vi "PC_JKS_v3.vi"() -> ()   [LabVIEW 2014]
panel:
  out "Strains":dbl[](array[numeric])
  out "Bosch.controller.values":dbl[](array[numeric])
  out "Mixed":dbl[](array[numeric])
  out "Override.values":dbl[](array[numeric])
  in  "Plot loop time":i64=50
  out "Comp":dbl[](array[numeric])
  out "Ramp":dbl[](array[numeric])
  out "Valves":dbl[](array[numeric])
  out "Sensors":dbl[](array[numeric])
  out "Time [s]":dbl
  out "Start.log":bool
  out "Log active 2":bool
  in  "Tab Control":T1(tab)
  in  "Stop logging":bool
  out "Numeric":i32
  out "Log active":bool
  in  "Log time (s)":dbl=20.0 caption="Time Target (s)"
  out "Elapsed Time (s)":dbl
  in  "Log frequency [ms]":u32=10
  in  "Start logging":bool
  out "Ready to save":bool
  in  "Filename":string="File"
  in  "Path":string="C:\\Dokumenter\\Dropbox\\Phd\\UiA\\Measurement\\Green_rig_data\\"
  in  "Prepare log":bool
  out "Waiting":bool
  out "U_PVG":dbl
  out "U_HAWE":dbl
  out "u_DCV":dbl=63.567989349365234
  out "P.B.HP":dbl=63.611995697021484
  out "u_Bosch":dbl
  out "FB.DCV":dbl=-1.8625760078430176
  out "P.B":dbl=70.21202850341797
  out "P.A":dbl=21.1690616607666
  out "P.return":dbl=0.036249998956918716
  out "P.pump":dbl=0.9932812452316284
  out "x.c":dbl=-0.41861194372177124
  out "P.B.LP":dbl=-0.3017437160015106
  out "P.A1":dbl=21.6378116607666
  out "Q.B":dbl=0.178985595703125
  out "FB.Bosch":dbl=0.0007812500116415322
  out "P.comp":dbl=0.15499994158744812
  out "u_DCV_comp":dbl
  out "Ramp.tr [s]":dbl
  out "Ramp.t.ramp [s]":dbl
  out "Ramp.ymax":dbl
  out "Ramp.direction":dbl
  out "Ramp.td [s]":dbl
  out "Comp.kF.gain":dbl
  out "Comp.Q.to.U.gain":dbl
  out "U_Bosch":dbl
  out "x.c.dot":dbl=63.611995697021484
  out "P.B.LP.v2":dbl=63.611995697021484
  out "Fake PB pressure":dbl
  out "Bosch Operation mode":dbl
  out "Bosch.p.term":dbl
  out "Bosch.i.term":dbl
  out "Bosch.d.term":dbl
  out "dL lowpass cutoff freq [Hz]":dbl
  out "dL HP cutoff freq [Hz]":dbl
  out "Pb highpass cutoff freq [Hz]":dbl
  out "Pb lowpass cutoff freq [Hz]":dbl
  out "Lower pressure limit [bar]":dbl
  out "Upper pressure limit [bar]":dbl
  out "Pressure (lowpass / direct (off))":dbl
  out "dpOpen (bar)":dbl
  out "Proportional.Gain":dbl
  out "Integral.Gain":dbl
  out "Derivative.Gain":dbl
  out "Bosch.ff.term":dbl
  out "Strain_unfiltered":dbl
  out "Strain_filtered":dbl
  out "plot_p_A_p_B":T2(graph)
  out "Pressure secondary circuit":T3(graph)
  out "plot_pressures":T4(graph)=[{"plot3"=[{"timer"=10600.0390625, "p_A"=21.1690616607666, "p_A1"=-0.41861194372177124}, {"timer"=10599.939453125, "p_A"=21.2081241607666, "p_A1"=-0.3771619200706482}, {"timer"=10599.859375, "p_A"=20.9737491607666, "p_A1"=-0.33571189641952515}, {"timer"=10599.7578125, "p_A"=20.7003116607666, "p_A1"=-0.25281187891960144}, {"timer"=10599.658203125, "p_A"=20.5245304107666, "p_A1"=-0.2942619025707245}, {"timer"=10599.55859375, "p_A"=20.8565616607666, "p_A1"=-0.25281187891960144}, {"timer"=10599.439453125, "p_A"=20.5049991607666, "p_A1"=-0.25281187891960144}, {"timer"=10599.337890625, "p_A"=20.0557804107666, "p_A1"=-0.2113618403673172}, {"timer"=10599.2578125, "p_A"=19.587032318115234, "p_A1"=-0.2942619025707245}, {"timer"=10599.158203125, "p_A"=19.743282318115234, "p_A1"=-0.1284618079662323}, {"timer"=10599.05859375, "p_A"=19.450313568115234, "p_A1"=-0.25281187891960144}, {"timer"=10598.958984375, "p_A"=19.333126068115234, "p_A1"=-0.2113618403673172}, {"timer"=10598.837890625, "p_A"=18.630001068115234, "p_A1"=-0.25281187891960144}, {"timer"=10598.73828125, "p_A"=18.864376068115234, "p_A1"=-0.33571189641952515}, {"timer"=10598.638671875, "p_A"=18.239376068115234, "p_A1"=-0.25281187891960144}, {"timer"=10598.55859375, "p_A"=18.141719818115234, "p_A1"=-0.25281187891960144}, {"timer"=10598.458984375, "p_A"=17.712032318115234, "p_A1"=-0.33571189641952515}, {"timer"=10598.359375, "p_A"=17.477657318115234, "p_A1"=-0.2942619025707245}, {"timer"=10598.23828125, "p_A"=17.380001068115234, "p_A1"=-0.2113618403673172}, {"timer"=10598.138671875, "p_A"=17.145626068115234, "p_A1"=-0.41861194372177124}, {"timer"=10598.05859375, "p_A"=16.891719818115234, "p_A1"=-0.33571189641952515}, {"timer"=10597.958984375, "p_A"=16.520626068115234, "p_A1"=-0.3771619200706482}, {"timer"=10597.859375, "p_A"=16.383907318115234, "p_A1"=-0.3771619200706482}, {"timer"=10597.7578125, "p_A"=15.934687614440918, "p_A1"=-0.41861194372177124}, {"timer"=10597.658203125, "p_A"=15.778437614440918, "p_A1"=-0.41861194372177124}, {"timer"=10597.55859375, "p_A"=15.524531364440918, "p_A1"=-0.2942619025707245}, {"timer"=10597.458984375, "p_A"=15.231562614440918, "p_A1"=-0.2942619025707245}, {"timer"=10597.359375, "p_A"=15.172968864440918, "p_A1"=-0.41861194372177124}, {"timer"=10597.23828125, "p_A"=14.684687614440918, "p_A1"=-0.25281187891960144}, {"timer"=10597.158203125, "p_A"=14.294062614440918, "p_A1"=-0.33571189641952515}, {"timer"=10597.05859375, "p_A"=14.294062614440918, "p_A1"=-0.2942619025707245}, {"timer"=10596.958984375, "p_A"=13.688593864440918, "p_A1"=-0.2942619025707245}, {"timer"=10596.859375, "p_A"=13.766718864440918, "p_A1"=-0.2942619025707245}, {"timer"=10596.7578125, "p_A"=13.571406364440918, "p_A1"=-0.3771619200706482}, {"timer"=10596.658203125, "p_A"=13.180781364440918, "p_A1"=-0.2942619025707245}, {"timer"=10596.55859375, "p_A"=12.809687614440918, "p_A1"=-0.2113618403673172}, {"timer"=10596.458984375, "p_A"=12.653437614440918, "p_A1"=-0.25281187891960144}, {"timer"=10596.359375, "p_A"=12.477656364440918, "p_A1"=-0.25281187891960144}, {"timer"=10596.2578125, "p_A"=12.008906364440918, "p_A1"=-0.2113618403673172}, {"timer"=10596.158203125, "p_A"=12.008906364440918, "p_A1"=-0.2942619025707245}, {"timer"=10596.05859375, "p_A"=11.364375114440918, "p_A1"=-0.25281187891960144}, {"timer"=10595.939453125, "p_A"=11.208125114440918, "p_A1"=-0.25281187891960144}, {"timer"=10595.859375, "p_A"=10.817500114440918, "p_A1"=-0.25281187891960144}, {"timer"=10595.7578125, "p_A"=10.505000114440918, "p_A1"=-0.33571189641952515}, {"timer"=10595.658203125, "p_A"=10.661250114440918, "p_A1"=-0.2942619025707245}, {"timer"=10595.5390625, "p_A"=9.919062614440918, "p_A1"=-0.33571189641952515}, {"timer"=10595.458984375, "p_A"=10.055781364440918, "p_A1"=-0.4600619673728943}, {"timer"=10595.359375, "p_A"=9.567500114440918, "p_A1"=-0.2942619025707245}, {"timer"=10595.2578125, "p_A"=9.274531364440918, "p_A1"=-0.33571189641952515}, {"timer"=10595.158203125, "p_A"=9.020625114440918, "p_A1"=-0.25281187891960144}, {"timer"=10595.0390625, "p_A"=8.981562614440918, "p_A1"=-0.33571189641952515}, {"timer"=10594.958984375, "p_A"=8.766718864440918, "p_A1"=-0.2942619025707245}, {"timer"=10594.859375, "p_A"=8.044062614440918, "p_A1"=-0.3771619200706482}, {"timer"=10594.7578125, "p_A"=7.98546838760376, "p_A1"=-0.2942619025707245}, {"timer"=10594.658203125, "p_A"=7.80968713760376, "p_A1"=-0.2942619025707245}, {"timer"=10594.55859375, "p_A"=7.39953088760376, "p_A1"=-0.41861194372177124}, {"timer"=10594.458984375, "p_A"=7.28234338760376, "p_A1"=-0.25281187891960144}, {"timer"=10594.359375, "p_A"=6.57921838760376, "p_A1"=-0.2113618403673172}, {"timer"=10594.23828125, "p_A"=6.52062463760376, "p_A1"=-0.33571189641952515}, {"timer"=10594.138671875, "p_A"=6.16906213760376, "p_A1"=-0.3771619200706482}, {"timer"=10594.05859375, "p_A"=5.99328088760376, "p_A1"=-0.33571189641952515}, {"timer"=10593.939453125, "p_A"=6.03234338760376, "p_A1"=-0.41861194372177124}, {"timer"=10593.837890625, "p_A"=5.48546838760376, "p_A1"=-0.33571189641952515}, {"timer"=10593.7578125, "p_A"=5.36828088760376, "p_A1"=-0.2942619025707245}, {"timer"=10593.658203125, "p_A"=4.938593864440918, "p_A1"=-0.3771619200706482}, {"timer"=10593.5390625, "p_A"=4.528437614440918, "p_A1"=-0.33571189641952515}, {"timer"=10593.439453125, "p_A"=4.528437614440918, "p_A1"=-0.3771619200706482}, {"timer"=10593.337890625, "p_A"=4.040156364440918, "p_A1"=-0.3771619200706482}, {"timer"=10593.2578125, "p_A"=3.883906364440918, "p_A1"=-0.33571189641952515}, {"timer"=10593.158203125, "p_A"=3.454218864440918, "p_A1"=-0.25281187891960144}, {"timer"=10593.05859375, "p_A"=2.887812614440918, "p_A1"=-0.25281187891960144}, {"timer"=10592.939453125, "p_A"=2.770625114440918, "p_A1"=-0.2942619025707245}, {"timer"=10592.859375, "p_A"=2.419062614440918, "p_A1"=-0.41861194372177124}, {"timer"=10592.7578125, "p_A"=2.106562614440918, "p_A1"=-0.3771619200706482}, {"timer"=10592.658203125, "p_A"=2.087031364440918, "p_A1"=-0.33571189641952515}, {"timer"=10592.5390625, "p_A"=1.598750114440918, "p_A1"=-0.33571189641952515}, {"timer"=10592.458984375, "p_A"=1.0714062452316284, "p_A1"=-0.2942619025707245}, {"timer"=10592.359375, "p_A"=0.8565624952316284, "p_A1"=-0.2942619025707245}, {"timer"=10592.2578125, "p_A"=0.07531249523162842, "p_A1"=-0.41861194372177124}, {"timer"=10592.158203125, "p_A"=-0.0028125010430812836, "p_A1"=-0.5015120506286621}, {"timer"=10592.05859375, "p_A"=0.6221874952316284, "p_A1"=-0.3771619200706482}, {"timer"=10591.958984375, "p_A"=12.380000114440918, "p_A1"=-0.2942619025707245}, {"timer"=10591.859375, "p_A"=45.07530975341797, "p_A1"=-0.2942619025707245}, {"timer"=10591.7578125, "p_A"=45.60265350341797, "p_A1"=-0.25281187891960144}, {"timer"=10591.638671875, "p_A"=46.20812225341797, "p_A1"=-0.41861194372177124}, {"timer"=10591.55859375, "p_A"=64.82140350341797, "p_A1"=-0.16991183161735535}, {"timer"=10591.439453125, "p_A"=96.40343475341797, "p_A1"=1.405189037322998}, {"timer"=10591.337890625, "p_A"=96.32530975341797, "p_A1"=1.6124391555786133}, {"timer"=10591.2578125, "p_A"=88.02452850341797, "p_A1"=1.6538891792297363}, {"timer"=10591.158203125, "p_A"=90.11437225341797, "p_A1"=1.6953392028808594}, {"timer"=10591.0390625, "p_A"=100.99327850341797, "p_A1"=3.8921902179718018}, {"timer"=10590.939453125, "p_A"=90.21202850341797, "p_A1"=4.4724907875061035}, {"timer"=10590.837890625, "p_A"=83.98155975341797, "p_A1"=4.969890594482422}, {"timer"=10590.7578125, "p_A"=99.46984100341797, "p_A1"=5.011341094970703}, {"timer"=10590.658203125, "p_A"=99.46984100341797, "p_A1"=5.177141189575195}, {"timer"=10590.55859375, "p_A"=99.64562225341797, "p_A1"=5.094240665435791}, {"timer"=10590.439453125, "p_A"=99.56749725341797, "p_A1"=5.218591213226318}, {"timer"=10590.359375, "p_A"=99.45030975341797, "p_A1"=5.052791118621826}, {"timer"=10590.2578125, "p_A"=99.60655975341797, "p_A1"=5.135690689086914}, {"timer"=10590.158203125, "p_A"=99.45030975341797, "p_A1"=5.094240665435791}, {"timer"=10590.0390625, "p_A"=99.62609100341797, "p_A1"=5.260040760040283}, {"timer"=10589.939453125, "p_A"=99.62609100341797, "p_A1"=5.135690689086914}, {"timer"=10589.837890625, "p_A"=99.64562225341797, "p_A1"=5.218591213226318}, {"timer"=10589.73828125, "p_A"=99.46984100341797, "p_A1"=5.177141189575195}, {"timer"=10589.658203125, "p_A"=99.60655975341797, "p_A1"=5.177141189575195}, {"timer"=10589.5390625, "p_A"=99.64562225341797, "p_A1"=5.218591213226318}, {"timer"=10589.458984375, "p_A"=99.66515350341797, "p_A1"=5.301490783691406}, {"timer"=10589.359375, "p_A"=99.50890350341797, "p_A1"=5.3429412841796875}, {"timer"=10589.23828125, "p_A"=99.50890350341797, "p_A1"=5.218591213226318}, {"timer"=10589.158203125, "p_A"=99.48937225341797, "p_A1"=5.260040760040283}, {"timer"=10589.05859375, "p_A"=99.45030975341797, "p_A1"=5.260040760040283}, {"timer"=10588.958984375, "p_A"=99.29405975341797, "p_A1"=5.301490783691406}, {"timer"=10588.859375, "p_A"=99.35265350341797, "p_A1"=5.301490783691406}, {"timer"=10588.7578125, "p_A"=99.52843475341797, "p_A1"=5.260040760040283}, {"timer"=10588.658203125, "p_A"=99.39171600341797, "p_A1"=5.3429412841796875}, {"timer"=10588.55859375, "p_A"=99.76280975341797, "p_A1"=5.3843913078308105}, {"timer"=10588.439453125, "p_A"=99.48937225341797, "p_A1"=5.3843913078308105}, {"timer"=10588.359375, "p_A"=99.50890350341797, "p_A1"=5.3429412841796875}, {"timer"=10588.2578125, "p_A"=99.50890350341797, "p_A1"=5.425840854644775}, {"timer"=10588.158203125, "p_A"=99.39171600341797, "p_A1"=5.3843913078308105}, {"timer"=10588.0390625, "p_A"=99.41124725341797, "p_A1"=5.3429412841796875}, {"timer"=10587.939453125, "p_A"=99.48937225341797, "p_A1"=5.467290878295898}, {"timer"=10587.859375, "p_A"=99.46984100341797, "p_A1"=5.425840854644775}, {"timer"=10587.7578125, "p_A"=99.43077850341797, "p_A1"=5.50874137878418}, {"timer"=10587.638671875, "p_A"=99.60655975341797, "p_A1"=5.467290878295898}, {"timer"=10587.55859375, "p_A"=99.41124725341797, "p_A1"=5.425840854644775}, {"timer"=10587.458984375, "p_A"=99.56749725341797, "p_A1"=5.3843913078308105}, {"timer"=10587.337890625, "p_A"=99.17687225341797, "p_A1"=5.50874137878418}, {"timer"=10587.23828125, "p_A"=99.56749725341797, "p_A1"=5.50874137878418}, {"timer"=10587.158203125, "p_A"=99.54796600341797, "p_A1"=5.50874137878418}, {"timer"=10587.05859375, "p_A"=99.45030975341797, "p_A1"=5.467290878295898}, {"timer"=10586.958984375, "p_A"=99.50890350341797, "p_A1"=5.467290878295898}, {"timer"=10586.859375, "p_A"=99.54796600341797, "p_A1"=5.467290878295898}, {"timer"=10586.7578125, "p_A"=99.45030975341797, "p_A1"=5.50874137878418}, {"timer"=10586.658203125, "p_A"=99.46984100341797, "p_A1"=5.50874137878418}, {"timer"=10586.55859375, "p_A"=99.54796600341797, "p_A1"=5.591640949249268}, {"timer"=10586.458984375, "p_A"=99.45030975341797, "p_A1"=5.715991497039795}, {"timer"=10586.359375, "p_A"=99.48937225341797, "p_A1"=5.715991497039795}, {"timer"=10586.2578125, "p_A"=99.25499725341797, "p_A1"=5.591640949249268}, {"timer"=10586.158203125, "p_A"=99.86046600341797, "p_A1"=5.550191402435303}, {"timer"=10586.05859375, "p_A"=99.35265350341797, "p_A1"=5.633090972900391}, {"timer"=10585.958984375, "p_A"=99.54796600341797, "p_A1"=5.591640949249268}, {"timer"=10585.859375, "p_A"=99.31359100341797, "p_A1"=5.550191402435303}, {"timer"=10585.7578125, "p_A"=99.39171600341797, "p_A1"=5.715991497039795}, {"timer"=10585.658203125, "p_A"=99.37218475341797, "p_A1"=5.75744104385376}, {"timer"=10585.55859375, "p_A"=99.37218475341797, "p_A1"=5.633090972900391}, {"timer"=10585.458984375, "p_A"=99.21593475341797, "p_A1"=5.674541473388672}, {"timer"=10585.359375, "p_A"=99.23546600341797, "p_A1"=5.674541473388672}, {"timer"=10585.2578125, "p_A"=99.43077850341797, "p_A1"=5.715991497039795}, {"timer"=10585.158203125, "p_A"=99.37218475341797, "p_A1"=5.75744104385376}, {"timer"=10585.05859375, "p_A"=99.54796600341797, "p_A1"=5.75744104385376}, {"timer"=10584.958984375, "p_A"=99.45030975341797, "p_A1"=5.798891067504883}, {"timer"=10584.837890625, "p_A"=99.39171600341797, "p_A1"=5.715991497039795}, {"timer"=10584.7578125, "p_A"=99.60655975341797, "p_A1"=5.75744104385376}, {"timer"=10584.658203125, "p_A"=99.48937225341797, "p_A1"=5.798891067504883}, {"timer"=10584.55859375, "p_A"=99.39171600341797, "p_A1"=5.715991497039795}, {"timer"=10584.458984375, "p_A"=99.35265350341797, "p_A1"=5.674541473388672}, {"timer"=10584.359375, "p_A"=99.21593475341797, "p_A1"=5.715991497039795}, {"timer"=10584.2578125, "p_A"=99.50890350341797, "p_A1"=5.798891067504883}, {"timer"=10584.158203125, "p_A"=99.58702850341797, "p_A1"=5.840341567993164}, {"timer"=10584.05859375, "p_A"=99.39171600341797, "p_A1"=5.881791591644287}, {"timer"=10583.958984375, "p_A"=99.50890350341797, "p_A1"=5.881791591644287}, {"timer"=10583.859375, "p_A"=99.41124725341797, "p_A1"=5.92324161529541}, {"timer"=10583.7578125, "p_A"=99.33312225341797, "p_A1"=5.840341567993164}, {"timer"=10583.658203125, "p_A"=99.33312225341797, "p_A1"=5.840341567993164}, {"timer"=10583.55859375, "p_A"=99.52843475341797, "p_A1"=5.92324161529541}, {"timer"=10583.458984375, "p_A"=99.33312225341797, "p_A1"=5.840341567993164}, {"timer"=10583.359375, "p_A"=99.52843475341797, "p_A1"=6.006141662597656}, {"timer"=10583.2578125, "p_A"=99.72374725341797, "p_A1"=5.964691162109375}, {"timer"=10583.158203125, "p_A"=99.48937225341797, "p_A1"=6.006141662597656}, {"timer"=10583.05859375, "p_A"=99.41124725341797, "p_A1"=6.006141662597656}, {"timer"=10582.958984375, "p_A"=99.45030975341797, "p_A1"=6.006141662597656}, {"timer"=10582.859375, "p_A"=99.43077850341797, "p_A1"=5.964691162109375}, {"timer"=10582.7578125, "p_A"=99.41124725341797, "p_A1"=6.006141662597656}, {"timer"=10582.658203125, "p_A"=99.37218475341797, "p_A1"=6.006141662597656}, {"timer"=10582.55859375, "p_A"=99.41124725341797, "p_A1"=5.964691162109375}, {"timer"=10582.458984375, "p_A"=99.58702850341797, "p_A1"=6.006141662597656}, {"timer"=10582.359375, "p_A"=99.37218475341797, "p_A1"=6.047591686248779}, {"timer"=10582.2578125, "p_A"=99.50890350341797, "p_A1"=6.089041709899902}, {"timer"=10582.158203125, "p_A"=99.35265350341797, "p_A1"=6.089041709899902}, {"timer"=10582.0390625, "p_A"=99.60655975341797, "p_A1"=6.047591686248779}, {"timer"=10581.958984375, "p_A"=99.76280975341797, "p_A1"=6.089041709899902}, {"timer"=10581.837890625, "p_A"=99.43077850341797, "p_A1"=6.006141662597656}, {"timer"=10581.73828125, "p_A"=99.37218475341797, "p_A1"=6.130491256713867}, {"timer"=10581.658203125, "p_A"=99.27452850341797, "p_A1"=6.089041709899902}, {"timer"=10581.55859375, "p_A"=99.48937225341797, "p_A1"=6.2548418045043945}, {"timer"=10581.458984375, "p_A"=99.46984100341797, "p_A1"=6.171941757202148}, {"timer"=10581.359375, "p_A"=99.33312225341797, "p_A1"=6.2133917808532715}, {"timer"=10581.23828125, "p_A"=99.25499725341797, "p_A1"=6.2133917808532715}, {"timer"=10581.158203125, "p_A"=99.58702850341797, "p_A1"=6.296291351318359}, {"timer"=10581.05859375, "p_A"=99.31359100341797, "p_A1"=6.296291351318359}, {"timer"=10580.958984375, "p_A"=99.37218475341797, "p_A1"=6.2133917808532715}, {"timer"=10580.859375, "p_A"=99.25499725341797, "p_A1"=6.379191875457764}, {"timer"=10580.7578125, "p_A"=99.27452850341797, "p_A1"=6.379191875457764}, {"timer"=10580.658203125, "p_A"=99.41124725341797, "p_A1"=6.379191875457764}, {"timer"=10580.55859375, "p_A"=99.62609100341797, "p_A1"=6.462091445922852}, {"timer"=10580.458984375, "p_A"=99.35265350341797, "p_A1"=6.337741851806641}, {"timer"=10580.359375, "p_A"=99.29405975341797, "p_A1"=6.462091445922852}, {"timer"=10580.2578125, "p_A"=99.09874725341797, "p_A1"=6.420641899108887}, {"timer"=10580.158203125, "p_A"=99.39171600341797, "p_A1"=6.379191875457764}, {"timer"=10580.05859375, "p_A"=99.33312225341797, "p_A1"=6.420641899108887}, {"timer"=10579.939453125, "p_A"=99.39171600341797, "p_A1"=6.544991970062256}, {"timer"=10579.837890625, "p_A"=99.29405975341797, "p_A1"=6.586441993713379}, {"timer"=10579.7578125, "p_A"=99.17687225341797, "p_A1"=6.544991970062256}, {"timer"=10579.658203125, "p_A"=99.48937225341797, "p_A1"=6.586441993713379}, {"timer"=10579.55859375, "p_A"=99.23546600341797, "p_A1"=6.503541946411133}, {"timer"=10579.439453125, "p_A"=99.33312225341797, "p_A1"=6.462091445922852}, {"timer"=10579.337890625, "p_A"=99.21593475341797, "p_A1"=6.586441993713379}, {"timer"=10579.23828125, "p_A"=99.60655975341797, "p_A1"=6.544991970062256}, {"timer"=10579.138671875, "p_A"=99.39171600341797, "p_A1"=6.544991970062256}, {"timer"=10579.0390625, "p_A"=99.46984100341797, "p_A1"=6.462091445922852}, {"timer"=10578.939453125, "p_A"=99.33312225341797, "p_A1"=6.503541946411133}, {"timer"=10578.837890625, "p_A"=99.21593475341797, "p_A1"=6.544991970062256}, {"timer"=10578.73828125, "p_A"=99.35265350341797, "p_A1"=6.586441993713379}, {"timer"=10578.638671875, "p_A"=99.31359100341797, "p_A1"=6.503541946411133}, {"timer"=10578.5390625, "p_A"=99.19640350341797, "p_A1"=6.544991970062256}, {"timer"=10578.439453125, "p_A"=99.68468475341797, "p_A1"=6.627891540527344}, {"timer"=10578.337890625, "p_A"=99.07921600341797, "p_A1"=6.503541946411133}, {"timer"=10578.23828125, "p_A"=99.29405975341797, "p_A1"=6.627891540527344}, {"timer"=10578.138671875, "p_A"=99.41124725341797, "p_A1"=6.669342041015625}, {"timer"=10578.0390625, "p_A"=99.54796600341797, "p_A1"=6.669342041015625}, {"timer"=10577.939453125, "p_A"=99.15734100341797, "p_A1"=6.627891540527344}, {"timer"=10577.837890625, "p_A"=99.33312225341797, "p_A1"=6.627891540527344}, {"timer"=10577.73828125, "p_A"=99.45030975341797, "p_A1"=6.586441993713379}, {"timer"=10577.638671875, "p_A"=99.19640350341797, "p_A1"=6.669342041015625}, {"timer"=10577.5390625, "p_A"=99.17687225341797, "p_A1"=6.627891540527344}, {"timer"=10577.439453125, "p_A"=99.29405975341797, "p_A1"=6.669342041015625}, {"timer"=10577.337890625, "p_A"=99.37218475341797, "p_A1"=6.669342041015625}, {"timer"=10577.23828125, "p_A"=99.45030975341797, "p_A1"=6.669342041015625}, {"timer"=10577.138671875, "p_A"=99.37218475341797, "p_A1"=6.752242088317871}, {"timer"=10577.0390625, "p_A"=99.46984100341797, "p_A1"=6.752242088317871}, {"timer"=10576.939453125, "p_A"=99.27452850341797, "p_A1"=6.835142135620117}, {"timer"=10576.837890625, "p_A"=99.19640350341797, "p_A1"=6.793691635131836}, {"timer"=10576.73828125, "p_A"=99.29405975341797, "p_A1"=6.752242088317871}, {"timer"=10576.638671875, "p_A"=99.29405975341797, "p_A1"=6.793691635131836}, {"timer"=10576.5390625, "p_A"=99.09874725341797, "p_A1"=6.793691635131836}, {"timer"=10576.439453125, "p_A"=99.21593475341797, "p_A1"=6.918042182922363}, {"timer"=10576.337890625, "p_A"=99.25499725341797, "p_A1"=6.835142135620117}, {"timer"=10576.23828125, "p_A"=99.25499725341797, "p_A1"=6.752242088317871}, {"timer"=10576.138671875, "p_A"=99.23546600341797, "p_A1"=6.835142135620117}, {"timer"=10576.0390625, "p_A"=99.09874725341797, "p_A1"=6.87659215927124}, {"timer"=10575.939453125, "p_A"=99.35265350341797, "p_A1"=6.918042182922363}, {"timer"=10575.837890625, "p_A"=99.29405975341797, "p_A1"=6.793691635131836}, {"timer"=10575.73828125, "p_A"=99.33312225341797, "p_A1"=6.87659215927124}, {"timer"=10575.638671875, "p_A"=99.45030975341797, "p_A1"=6.835142135620117}, {"timer"=10575.5390625, "p_A"=99.29405975341797, "p_A1"=6.87659215927124}, {"timer"=10575.439453125, "p_A"=99.17687225341797, "p_A1"=6.918042182922363}, {"timer"=10575.337890625, "p_A"=99.11827850341797, "p_A1"=6.959491729736328}, {"timer"=10575.23828125, "p_A"=99.13780975341797, "p_A1"=6.87659215927124}, {"timer"=10575.138671875, "p_A"=99.09874725341797, "p_A1"=6.918042182922363}, {"timer"=10575.0390625, "p_A"=99.39171600341797, "p_A1"=6.918042182922363}, {"timer"=10574.939453125, "p_A"=99.48937225341797, "p_A1"=7.042392253875732}, {"timer"=10574.837890625, "p_A"=99.41124725341797, "p_A1"=6.918042182922363}, {"timer"=10574.73828125, "p_A"=99.45030975341797, "p_A1"=6.918042182922363}, {"timer"=10574.638671875, "p_A"=99.23546600341797, "p_A1"=7.000941753387451}, {"timer"=10574.5390625, "p_A"=99.29405975341797, "p_A1"=6.87659215927124}, {"timer"=10574.439453125, "p_A"=99.35265350341797, "p_A1"=6.87659215927124}, {"timer"=10574.337890625, "p_A"=99.29405975341797, "p_A1"=6.959491729736328}, {"timer"=10574.23828125, "p_A"=99.37218475341797, "p_A1"=7.042392253875732}, {"timer"=10574.138671875, "p_A"=99.25499725341797, "p_A1"=7.000941753387451}, {"timer"=10574.0390625, "p_A"=99.25499725341797, "p_A1"=7.000941753387451}, {"timer"=10573.939453125, "p_A"=99.25499725341797, "p_A1"=6.959491729736328}, {"timer"=10573.837890625, "p_A"=99.37218475341797, "p_A1"=7.0838422775268555}, {"timer"=10573.73828125, "p_A"=99.23546600341797, "p_A1"=7.000941753387451}, {"timer"=10573.638671875, "p_A"=99.17687225341797, "p_A1"=7.042392253875732}, {"timer"=10573.5390625, "p_A"=99.33312225341797, "p_A1"=7.000941753387451}, {"timer"=10573.439453125, "p_A"=99.19640350341797, "p_A1"=7.042392253875732}, {"timer"=10573.337890625, "p_A"=99.33312225341797, "p_A1"=7.12529182434082}, {"timer"=10573.23828125, "p_A"=99.31359100341797, "p_A1"=6.959491729736328}, {"timer"=10573.138671875, "p_A"=99.15734100341797, "p_A1"=7.000941753387451}, {"timer"=10573.0390625, "p_A"=99.27452850341797, "p_A1"=7.000941753387451}, {"timer"=10572.939453125, "p_A"=98.96202850341797, "p_A1"=6.959491729736328}, {"timer"=10572.837890625, "p_A"=99.33312225341797, "p_A1"=7.0838422775268555}, {"timer"=10572.73828125, "p_A"=99.31359100341797, "p_A1"=7.12529182434082}, {"timer"=10572.638671875, "p_A"=99.27452850341797, "p_A1"=7.042392253875732}, {"timer"=10572.5390625, "p_A"=99.15734100341797, "p_A1"=7.0838422775268555}, {"timer"=10572.439453125, "p_A"=99.33312225341797, "p_A1"=7.0838422775268555}, {"timer"=10572.337890625, "p_A"=99.31359100341797, "p_A1"=7.042392253875732}, {"timer"=10572.23828125, "p_A"=99.25499725341797, "p_A1"=7.0838422775268555}, {"timer"=10572.138671875, "p_A"=99.48937225341797, "p_A1"=7.0838422775268555}, {"timer"=10572.0390625, "p_A"=99.21593475341797, "p_A1"=7.0838422775268555}, {"timer"=10571.939453125, "p_A"=98.96202850341797, "p_A1"=7.0838422775268555}, {"timer"=10571.837890625, "p_A"=99.25499725341797, "p_A1"=7.042392253875732}, {"timer"=10571.73828125, "p_A"=99.17687225341797, "p_A1"=7.12529182434082}, {"timer"=10571.638671875, "p_A"=99.31359100341797, "p_A1"=7.12529182434082}, {"timer"=10571.5390625, "p_A"=99.13780975341797, "p_A1"=7.166741847991943}, {"timer"=10571.439453125, "p_A"=99.41124725341797, "p_A1"=7.0838422775268555}, {"timer"=10571.337890625, "p_A"=99.39171600341797, "p_A1"=7.166741847991943}, {"timer"=10571.23828125, "p_A"=99.09874725341797, "p_A1"=7.12529182434082}, {"timer"=10571.138671875, "p_A"=99.31359100341797, "p_A1"=7.12529182434082}, {"timer"=10571.0390625, "p_A"=99.09874725341797, "p_A1"=7.000941753387451}, {"timer"=10570.939453125, "p_A"=99.25499725341797, "p_A1"=7.166741847991943}, {"timer"=10570.837890625, "p_A"=99.19640350341797, "p_A1"=7.042392253875732}, {"timer"=10570.73828125, "p_A"=99.25499725341797, "p_A1"=7.0838422775268555}, {"timer"=10570.638671875, "p_A"=99.19640350341797, "p_A1"=7.166741847991943}, {"timer"=10570.5390625, "p_A"=99.25499725341797, "p_A1"=7.12529182434082}, {"timer"=10570.439453125, "p_A"=99.21593475341797, "p_A1"=7.166741847991943}, {"timer"=10570.337890625, "p_A"=99.31359100341797, "p_A1"=7.12529182434082}, {"timer"=10570.23828125, "p_A"=99.11827850341797, "p_A1"=7.0838422775268555}, {"timer"=10570.138671875, "p_A"=99.35265350341797, "p_A1"=7.0838422775268555}, {"timer"=10570.0390625, "p_A"=99.35265350341797, "p_A1"=7.12529182434082}, {"timer"=10569.939453125, "p_A"=99.39171600341797, "p_A1"=7.12529182434082}, {"timer"=10569.837890625, "p_A"=98.92296600341797, "p_A1"=7.208192348480225}, {"timer"=10569.73828125, "p_A"=99.00109100341797, "p_A1"=7.166741847991943}, {"timer"=10569.638671875, "p_A"=98.96202850341797, "p_A1"=7.12529182434082}, {"timer"=10569.5390625, "p_A"=99.04015350341797, "p_A1"=7.12529182434082}, {"timer"=10569.439453125, "p_A"=99.07921600341797, "p_A1"=7.166741847991943}, {"timer"=10569.337890625, "p_A"=99.17687225341797, "p_A1"=7.12529182434082}, {"timer"=10569.23828125, "p_A"=99.17687225341797, "p_A1"=7.12529182434082}, {"timer"=10569.138671875, "p_A"=99.11827850341797, "p_A1"=7.166741847991943}, {"timer"=10569.0390625, "p_A"=99.13780975341797, "p_A1"=7.0838422775268555}, {"timer"=10568.939453125, "p_A"=99.02062225341797, "p_A1"=7.166741847991943}, {"timer"=10568.837890625, "p_A"=99.13780975341797, "p_A1"=7.166741847991943}, {"timer"=10568.73828125, "p_A"=99.05968475341797, "p_A1"=7.166741847991943}, {"timer"=10568.638671875, "p_A"=99.21593475341797, "p_A1"=7.12529182434082}, {"timer"=10568.5390625, "p_A"=99.21593475341797, "p_A1"=7.166741847991943}, {"timer"=10568.439453125, "p_A"=99.04015350341797, "p_A1"=7.208192348480225}, {"timer"=10568.337890625, "p_A"=99.09874725341797, "p_A1"=7.12529182434082}, {"timer"=10568.23828125, "p_A"=99.21593475341797, "p_A1"=7.12529182434082}, {"timer"=10568.138671875, "p_A"=99.05968475341797, "p_A1"=7.208192348480225}, {"timer"=10568.0390625, "p_A"=99.37218475341797, "p_A1"=7.208192348480225}, {"timer"=10567.939453125, "p_A"=99.31359100341797, "p_A1"=7.208192348480225}, {"timer"=10567.837890625, "p_A"=99.07921600341797, "p_A1"=7.208192348480225}, {"timer"=10567.73828125, "p_A"=99.05968475341797, "p_A1"=7.208192348480225}, {"timer"=10567.638671875, "p_A"=99.23546600341797, "p_A1"=7.249642372131348}, {"timer"=10567.5390625, "p_A"=99.17687225341797, "p_A1"=7.249642372131348}, {"timer"=10567.439453125, "p_A"=99.07921600341797, "p_A1"=7.208192348480225}, {"timer"=10567.337890625, "p_A"=99.19640350341797, "p_A1"=7.208192348480225}, {"timer"=10567.23828125, "p_A"=99.00109100341797, "p_A1"=7.208192348480225}, {"timer"=10567.138671875, "p_A"=99.02062225341797, "p_A1"=7.208192348480225}, {"timer"=10567.0390625, "p_A"=99.19640350341797, "p_A1"=7.208192348480225}, {"timer"=10566.939453125, "p_A"=99.35265350341797, "p_A1"=7.208192348480225}, {"timer"=10566.837890625, "p_A"=98.94249725341797, "p_A1"=7.208192348480225}, {"timer"=10566.73828125, "p_A"=99.27452850341797, "p_A1"=7.249642372131348}, {"timer"=10566.638671875, "p_A"=98.86437225341797, "p_A1"=7.166741847991943}, {"timer"=10566.5390625, "p_A"=99.00109100341797, "p_A1"=7.249642372131348}, {"timer"=10566.439453125, "p_A"=98.92296600341797, "p_A1"=7.166741847991943}, {"timer"=10566.337890625, "p_A"=99.15734100341797, "p_A1"=7.166741847991943}, {"timer"=10566.23828125, "p_A"=99.04015350341797, "p_A1"=7.166741847991943}, {"timer"=10566.138671875, "p_A"=99.35265350341797, "p_A1"=7.208192348480225}, {"timer"=10566.0390625, "p_A"=99.09874725341797, "p_A1"=7.208192348480225}, {"timer"=10565.939453125, "p_A"=99.13780975341797, "p_A1"=7.249642372131348}, {"timer"=10565.837890625, "p_A"=99.17687225341797, "p_A1"=7.208192348480225}, {"timer"=10565.73828125, "p_A"=99.35265350341797, "p_A1"=7.208192348480225}, {"timer"=10565.638671875, "p_A"=99.15734100341797, "p_A1"=7.249642372131348}, {"timer"=10565.5390625, "p_A"=99.27452850341797, "p_A1"=7.208192348480225}, {"timer"=10565.439453125, "p_A"=98.94249725341797, "p_A1"=7.249642372131348}, {"timer"=10565.337890625, "p_A"=99.04015350341797, "p_A1"=7.208192348480225}, {"timer"=10565.23828125, "p_A"=99.11827850341797, "p_A1"=7.249642372131348}, {"timer"=10565.138671875, "p_A"=98.98155975341797, "p_A1"=7.208192348480225}, {"timer"=10565.0390625, "p_A"=99.02062225341797, "p_A1"=7.249642372131348}, {"timer"=10564.939453125, "p_A"=99.31359100341797, "p_A1"=7.249642372131348}, {"timer"=10564.837890625, "p_A"=99.07921600341797, "p_A1"=7.249642372131348}, {"timer"=10564.73828125, "p_A"=99.21593475341797, "p_A1"=7.208192348480225}, {"timer"=10564.638671875, "p_A"=99.27452850341797, "p_A1"=7.2910919189453125}, {"timer"=10564.5390625, "p_A"=99.27452850341797, "p_A1"=7.249642372131348}, {"timer"=10564.439453125, "p_A"=99.02062225341797, "p_A1"=7.249642372131348}, {"timer"=10564.337890625, "p_A"=99.23546600341797, "p_A1"=7.249642372131348}, {"timer"=10564.23828125, "p_A"=99.00109100341797, "p_A1"=7.249642372131348}, {"timer"=10564.138671875, "p_A"=99.23546600341797, "p_A1"=7.249642372131348}, {"timer"=10564.0390625, "p_A"=99.02062225341797, "p_A1"=7.249642372131348}, {"timer"=10563.939453125, "p_A"=99.19640350341797, "p_A1"=7.249642372131348}, {"timer"=10563.837890625, "p_A"=98.88390350341797, "p_A1"=7.249642372131348}, {"timer"=10563.73828125, "p_A"=99.11827850341797, "p_A1"=7.208192348480225}, {"timer"=10563.638671875, "p_A"=99.23546600341797, "p_A1"=7.249642372131348}, {"timer"=10563.5390625, "p_A"=99.21593475341797, "p_A1"=7.249642372131348}, {"timer"=10563.439453125, "p_A"=99.02062225341797, "p_A1"=7.249642372131348}, {"timer"=10563.337890625, "p_A"=99.11827850341797, "p_A1"=7.2910919189453125}, {"timer"=10563.23828125, "p_A"=99.02062225341797, "p_A1"=7.249642372131348}, {"timer"=10563.138671875, "p_A"=98.88390350341797, "p_A1"=7.249642372131348}, {"timer"=10563.0390625, "p_A"=99.13780975341797, "p_A1"=7.2910919189453125}, {"timer"=10562.939453125, "p_A"=98.68859100341797, "p_A1"=7.249642372131348}, {"timer"=10562.837890625, "p_A"=98.86437225341797, "p_A1"=7.249642372131348}, {"timer"=10562.73828125, "p_A"=98.94249725341797, "p_A1"=7.2910919189453125}, {"timer"=10562.638671875, "p_A"=99.04015350341797, "p_A1"=7.249642372131348}, {"timer"=10562.5390625, "p_A"=99.00109100341797, "p_A1"=7.249642372131348}, {"timer"=10562.439453125, "p_A"=98.84484100341797, "p_A1"=7.249642372131348}, {"timer"=10562.337890625, "p_A"=99.07921600341797, "p_A1"=7.249642372131348}, {"timer"=10562.23828125, "p_A"=99.02062225341797, "p_A1"=7.2910919189453125}, {"timer"=10562.138671875, "p_A"=99.15734100341797, "p_A1"=7.249642372131348}, {"timer"=10562.0390625, "p_A"=99.04015350341797, "p_A1"=7.249642372131348}, {"timer"=10561.939453125, "p_A"=99.13780975341797, "p_A1"=7.249642372131348}, {"timer"=10561.837890625, "p_A"=99.13780975341797, "p_A1"=7.2910919189453125}, {"timer"=10561.73828125, "p_A"=99.21593475341797, "p_A1"=7.2910919189453125}, {"timer"=10561.638671875, "p_A"=98.98155975341797, "p_A1"=7.249642372131348}, {"timer"=10561.5390625, "p_A"=99.04015350341797, "p_A1"=7.249642372131348}, {"timer"=10561.439453125, "p_A"=99.23546600341797, "p_A1"=7.2910919189453125}, {"timer"=10561.337890625, "p_A"=98.88390350341797, "p_A1"=7.249642372131348}, {"timer"=10561.23828125, "p_A"=99.17687225341797, "p_A1"=7.2910919189453125}, {"timer"=10561.138671875, "p_A"=99.27452850341797, "p_A1"=7.2910919189453125}, {"timer"=10561.0390625, "p_A"=99.11827850341797, "p_A1"=7.249642372131348}, {"timer"=10560.939453125, "p_A"=98.80577850341797, "p_A1"=7.249642372131348}, {"timer"=10560.837890625, "p_A"=99.17687225341797, "p_A1"=7.249642372131348}, {"timer"=10560.73828125, "p_A"=99.17687225341797, "p_A1"=7.2910919189453125}, {"timer"=10560.638671875, "p_A"=99.05968475341797, "p_A1"=7.249642372131348}, {"timer"=10560.5390625, "p_A"=99.04015350341797, "p_A1"=7.249642372131348}, {"timer"=10560.439453125, "p_A"=99.04015350341797, "p_A1"=7.249642372131348}, {"timer"=10560.337890625, "p_A"=99.13780975341797, "p_A1"=7.2910919189453125}, {"timer"=10560.23828125, "p_A"=98.94249725341797, "p_A1"=7.249642372131348}, {"timer"=10560.138671875, "p_A"=99.02062225341797, "p_A1"=7.2910919189453125}, {"timer"=10560.0390625, "p_A"=99.04015350341797, "p_A1"=7.249642372131348}, {"timer"=10559.939453125, "p_A"=99.09874725341797, "p_A1"=7.249642372131348}, {"timer"=10559.837890625, "p_A"=98.82530975341797, "p_A1"=7.2910919189453125}, {"timer"=10559.73828125, "p_A"=98.92296600341797, "p_A1"=7.2910919189453125}, {"timer"=10559.638671875, "p_A"=98.98155975341797, "p_A1"=7.249642372131348}, {"timer"=10559.5390625, "p_A"=98.76671600341797, "p_A1"=7.249642372131348}, {"timer"=10559.439453125, "p_A"=99.07921600341797, "p_A1"=7.2910919189453125}, {"timer"=10559.337890625, "p_A"=98.98155975341797, "p_A1"=7.2910919189453125}, {"timer"=10559.23828125, "p_A"=99.04015350341797, "p_A1"=7.2910919189453125}, {"timer"=10559.138671875, "p_A"=99.00109100341797, "p_A1"=7.249642372131348}, {"timer"=10559.0390625, "p_A"=98.96202850341797, "p_A1"=7.2910919189453125}, {"timer"=10558.939453125, "p_A"=99.13780975341797, "p_A1"=7.2910919189453125}, {"timer"=10558.837890625, "p_A"=98.92296600341797, "p_A1"=7.2910919189453125}, {"timer"=10558.73828125, "p_A"=98.82530975341797, "p_A1"=7.2910919189453125}, {"timer"=10558.619140625, "p_A"=99.05968475341797, "p_A1"=7.2910919189453125}, {"timer"=10558.5390625, "p_A"=98.88390350341797, "p_A1"=7.2910919189453125}, {"timer"=10558.439453125, "p_A"=98.92296600341797, "p_A1"=7.2910919189453125}, {"timer"=10558.337890625, "p_A"=98.96202850341797, "p_A1"=7.2910919189453125}, {"timer"=10558.21875, "p_A"=98.68859100341797, "p_A1"=7.2910919189453125}, {"timer"=10558.138671875, "p_A"=98.92296600341797, "p_A1"=7.2910919189453125}, {"timer"=10558.0390625, "p_A"=98.96202850341797, "p_A1"=7.2910919189453125}, {"timer"=10557.939453125, "p_A"=98.88390350341797, "p_A1"=7.249642372131348}, {"timer"=10557.837890625, "p_A"=98.94249725341797, "p_A1"=7.2910919189453125}, {"timer"=10557.73828125, "p_A"=99.15734100341797, "p_A1"=7.2910919189453125}, {"timer"=10557.638671875, "p_A"=99.07921600341797, "p_A1"=7.2910919189453125}, {"timer"=10557.5390625, "p_A"=99.09874725341797, "p_A1"=7.2910919189453125}, {"timer"=10557.439453125, "p_A"=98.82530975341797, "p_A1"=7.2910919189453125}, {"timer"=10557.337890625, "p_A"=98.90343475341797, "p_A1"=7.2910919189453125}, {"timer"=10557.23828125, "p_A"=98.96202850341797, "p_A1"=7.2910919189453125}, {"timer"=10557.138671875, "p_A"=99.07921600341797, "p_A1"=7.2910919189453125}, {"timer"=10557.0390625, "p_A"=98.76671600341797, "p_A1"=7.2910919189453125}, {"timer"=10556.939453125, "p_A"=99.02062225341797, "p_A1"=7.2910919189453125}, {"timer"=10556.837890625, "p_A"=99.00109100341797, "p_A1"=7.2910919189453125}, {"timer"=10556.73828125, "p_A"=98.92296600341797, "p_A1"=7.2910919189453125}, {"timer"=10556.638671875, "p_A"=98.66905975341797, "p_A1"=7.2910919189453125}, {"timer"=10556.5390625, "p_A"=98.80577850341797, "p_A1"=7.2910919189453125}, {"timer"=10556.439453125, "p_A"=98.92296600341797, "p_A1"=7.2910919189453125}, {"timer"=10556.337890625, "p_A"=99.02062225341797, "p_A1"=7.2910919189453125}, {"timer"=10556.21875, "p_A"=98.92296600341797, "p_A1"=7.2910919189453125}, {"timer"=10556.138671875, "p_A"=98.90343475341797, "p_A1"=7.2910919189453125}, {"timer"=10556.0390625, "p_A"=98.90343475341797, "p_A1"=7.2910919189453125}, {"timer"=10555.939453125, "p_A"=98.74718475341797, "p_A1"=7.2910919189453125}, {"timer"=10555.837890625, "p_A"=98.86437225341797, "p_A1"=7.2910919189453125}, {"timer"=10555.73828125, "p_A"=99.09874725341797, "p_A1"=7.2910919189453125}, {"timer"=10555.638671875, "p_A"=98.82530975341797, "p_A1"=7.3325419425964355}, {"timer"=10555.5390625, "p_A"=98.61046600341797, "p_A1"=7.2910919189453125}, {"timer"=10555.439453125, "p_A"=98.82530975341797, "p_A1"=7.3325419425964355}, {"timer"=10555.337890625, "p_A"=98.80577850341797, "p_A1"=7.2910919189453125}, {"timer"=10555.23828125, "p_A"=98.96202850341797, "p_A1"=7.2910919189453125}, {"timer"=10555.138671875, "p_A"=98.82530975341797, "p_A1"=7.2910919189453125}, {"timer"=10555.0390625, "p_A"=98.88390350341797, "p_A1"=7.2910919189453125}, {"timer"=10554.939453125, "p_A"=98.68859100341797, "p_A1"=7.2910919189453125}, {"timer"=10554.837890625, "p_A"=99.09874725341797, "p_A1"=7.2910919189453125}, {"timer"=10554.73828125, "p_A"=98.80577850341797, "p_A1"=7.2910919189453125}, {"timer"=10554.638671875, "p_A"=98.98155975341797, "p_A1"=7.3325419425964355}, {"timer"=10554.5390625, "p_A"=98.88390350341797, "p_A1"=7.2910919189453125}, {"timer"=10554.439453125, "p_A"=98.92296600341797, "p_A1"=7.2910919189453125}, {"timer"=10554.337890625, "p_A"=98.76671600341797, "p_A1"=7.3325419425964355}, {"timer"=10554.23828125, "p_A"=98.82530975341797, "p_A1"=7.2910919189453125}, {"timer"=10554.138671875, "p_A"=98.88390350341797, "p_A1"=7.2910919189453125}, {"timer"=10554.0390625, "p_A"=99.04015350341797, "p_A1"=7.2910919189453125}, {"timer"=10553.939453125, "p_A"=99.19640350341797, "p_A1"=7.2910919189453125}, {"timer"=10553.837890625, "p_A"=98.84484100341797, "p_A1"=7.2910919189453125}, {"timer"=10553.73828125, "p_A"=99.07921600341797, "p_A1"=7.2910919189453125}, {"timer"=10553.638671875, "p_A"=98.61046600341797, "p_A1"=7.2910919189453125}, {"timer"=10553.5390625, "p_A"=98.80577850341797, "p_A1"=7.2910919189453125}, {"timer"=10553.439453125, "p_A"=98.98155975341797, "p_A1"=7.2910919189453125}, {"timer"=10553.337890625, "p_A"=98.82530975341797, "p_A1"=7.2910919189453125}, {"timer"=10553.23828125, "p_A"=98.72765350341797, "p_A1"=7.2910919189453125}, {"timer"=10553.138671875, "p_A"=99.04015350341797, "p_A1"=7.2910919189453125}, {"timer"=10553.0390625, "p_A"=98.80577850341797, "p_A1"=7.3325419425964355}, {"timer"=10552.939453125, "p_A"=98.61046600341797, "p_A1"=7.2910919189453125}, {"timer"=10552.837890625, "p_A"=99.11827850341797, "p_A1"=7.2910919189453125}, {"timer"=10552.73828125, "p_A"=98.92296600341797, "p_A1"=7.2910919189453125}, {"timer"=10552.638671875, "p_A"=98.78624725341797, "p_A1"=7.3325419425964355}, {"timer"=10552.5390625, "p_A"=98.86437225341797, "p_A1"=7.2910919189453125}, {"timer"=10552.439453125, "p_A"=98.66905975341797, "p_A1"=7.3325419425964355}, {"timer"=10552.337890625, "p_A"=98.92296600341797, "p_A1"=7.2910919189453125}, {"timer"=10552.23828125, "p_A"=98.70812225341797, "p_A1"=7.3325419425964355}, {"timer"=10552.138671875, "p_A"=98.78624725341797, "p_A1"=7.3325419425964355}, {"timer"=10552.0390625, "p_A"=98.64952850341797, "p_A1"=7.2910919189453125}, {"timer"=10551.939453125, "p_A"=98.98155975341797, "p_A1"=7.2910919189453125}, {"timer"=10551.818359375, "p_A"=98.78624725341797, "p_A1"=7.2910919189453125}, {"timer"=10551.73828125, "p_A"=98.43468475341797, "p_A1"=7.3325419425964355}, {"timer"=10551.619140625, "p_A"=98.76671600341797, "p_A1"=7.2910919189453125}, {"timer"=10551.5390625, "p_A"=98.68859100341797, "p_A1"=7.2910919189453125}, {"timer"=10551.439453125, "p_A"=98.78624725341797, "p_A1"=7.3325419425964355}, {"timer"=10551.337890625, "p_A"=98.92296600341797, "p_A1"=7.3325419425964355}, {"timer"=10551.23828125, "p_A"=98.74718475341797, "p_A1"=7.3325419425964355}, {"timer"=10551.138671875, "p_A"=98.61046600341797, "p_A1"=7.3325419425964355}, {"timer"=10551.0390625, "p_A"=98.92296600341797, "p_A1"=7.2910919189453125}, {"timer"=10550.939453125, "p_A"=98.88390350341797, "p_A1"=7.2910919189453125}, {"timer"=10550.837890625, "p_A"=98.62999725341797, "p_A1"=7.2910919189453125}, {"timer"=10550.73828125, "p_A"=98.68859100341797, "p_A1"=7.3325419425964355}, {"timer"=10550.638671875, "p_A"=98.84484100341797, "p_A1"=7.3325419425964355}, {"timer"=10550.5390625, "p_A"=98.80577850341797, "p_A1"=7.3325419425964355}, {"timer"=10550.439453125, "p_A"=98.78624725341797, "p_A1"=7.2910919189453125}, {"timer"=10550.337890625, "p_A"=98.57140350341797, "p_A1"=7.3325419425964355}, {"timer"=10550.23828125, "p_A"=98.76671600341797, "p_A1"=7.2910919189453125}, {"timer"=10550.138671875, "p_A"=98.64952850341797, "p_A1"=7.3325419425964355}, {"timer"=10550.0390625, "p_A"=98.59093475341797, "p_A1"=7.3325419425964355}, {"timer"=10549.939453125, "p_A"=98.62999725341797, "p_A1"=7.3325419425964355}, {"timer"=10549.837890625, "p_A"=98.86437225341797, "p_A1"=7.3325419425964355}, {"timer"=10549.73828125, "p_A"=98.78624725341797, "p_A1"=7.3325419425964355}, {"timer"=10549.638671875, "p_A"=98.80577850341797, "p_A1"=7.3325419425964355}, {"timer"=10549.5390625, "p_A"=98.59093475341797, "p_A1"=7.3325419425964355}, {"timer"=10549.439453125, "p_A"=98.66905975341797, "p_A1"=7.3325419425964355}, {"timer"=10549.337890625, "p_A"=98.61046600341797, "p_A1"=7.2910919189453125}, {"timer"=10549.23828125, "p_A"=98.74718475341797, "p_A1"=7.3325419425964355}, {"timer"=10549.138671875, "p_A"=98.84484100341797, "p_A1"=7.3325419425964355}, {"timer"=10549.0390625, "p_A"=98.53234100341797, "p_A1"=7.2910919189453125}, {"timer"=10548.939453125, "p_A"=98.74718475341797, "p_A1"=7.3325419425964355}, {"timer"=10548.837890625, "p_A"=98.86437225341797, "p_A1"=7.3325419425964355}, {"timer"=10548.73828125, "p_A"=98.76671600341797, "p_A1"=7.3325419425964355}, {"timer"=10548.638671875, "p_A"=98.64952850341797, "p_A1"=7.3325419425964355}, {"timer"=10548.5390625, "p_A"=98.68859100341797, "p_A1"=7.3325419425964355}, {"timer"=10548.439453125, "p_A"=98.68859100341797, "p_A1"=7.3325419425964355}, {"timer"=10548.337890625, "p_A"=98.61046600341797, "p_A1"=7.3325419425964355}, {"timer"=10548.23828125, "p_A"=98.72765350341797, "p_A1"=7.3325419425964355}, {"timer"=10548.138671875, "p_A"=98.72765350341797, "p_A1"=7.3325419425964355}, {"timer"=10548.0390625, "p_A"=98.72765350341797, "p_A1"=7.3325419425964355}, {"timer"=10547.939453125, "p_A"=98.68859100341797, "p_A1"=7.3325419425964355}, {"timer"=10547.837890625, "p_A"=98.74718475341797, "p_A1"=7.3325419425964355}, {"timer"=10547.73828125, "p_A"=98.84484100341797, "p_A1"=7.3325419425964355}, {"timer"=10547.638671875, "p_A"=98.80577850341797, "p_A1"=7.3325419425964355}, {"timer"=10547.5390625, "p_A"=98.76671600341797, "p_A1"=7.3325419425964355}, {"timer"=10547.439453125, "p_A"=98.41515350341797, "p_A1"=7.2910919189453125}, {"timer"=10547.337890625, "p_A"=98.39562225341797, "p_A1"=7.3325419425964355}, {"timer"=10547.23828125, "p_A"=98.49327850341797, "p_A1"=7.3325419425964355}, {"timer"=10547.138671875, "p_A"=98.74718475341797, "p_A1"=7.3325419425964355}, {"timer"=10547.0390625, "p_A"=98.94249725341797, "p_A1"=7.3325419425964355}, {"timer"=10546.939453125, "p_A"=98.80577850341797, "p_A1"=7.3325419425964355}, {"timer"=10546.837890625, "p_A"=98.62999725341797, "p_A1"=7.3325419425964355}, {"timer"=10546.73828125, "p_A"=98.66905975341797, "p_A1"=7.3325419425964355}, {"timer"=10546.638671875, "p_A"=98.43468475341797, "p_A1"=7.3325419425964355}, {"timer"=10546.5390625, "p_A"=98.84484100341797, "p_A1"=7.3325419425964355}, {"timer"=10546.439453125, "p_A"=98.74718475341797, "p_A1"=7.3325419425964355}, {"timer"=10546.337890625, "p_A"=98.64952850341797, "p_A1"=7.3325419425964355}, {"timer"=10546.23828125, "p_A"=98.62999725341797, "p_A1"=7.3325419425964355}, {"timer"=10546.138671875, "p_A"=98.62999725341797, "p_A1"=7.3325419425964355}, {"timer"=10546.0390625, "p_A"=98.62999725341797, "p_A1"=7.3325419425964355}, {"timer"=10545.939453125, "p_A"=98.72765350341797, "p_A1"=7.3325419425964355}, {"timer"=10545.837890625, "p_A"=98.43468475341797, "p_A1"=7.3325419425964355}, {"timer"=10545.73828125, "p_A"=98.57140350341797, "p_A1"=7.3325419425964355}, {"timer"=10545.638671875, "p_A"=98.51280975341797, "p_A1"=7.3325419425964355}, {"timer"=10545.5390625, "p_A"=98.49327850341797, "p_A1"=7.3325419425964355}, {"timer"=10545.439453125, "p_A"=98.72765350341797, "p_A1"=7.3325419425964355}, {"timer"=10545.337890625, "p_A"=98.61046600341797, "p_A1"=7.3325419425964355}, {"timer"=10545.23828125, "p_A"=98.53234100341797, "p_A1"=7.3325419425964355}, {"timer"=10545.138671875, "p_A"=98.57140350341797, "p_A1"=7.3325419425964355}, {"timer"=10545.0390625, "p_A"=98.53234100341797, "p_A1"=7.3325419425964355}, {"timer"=10544.939453125, "p_A"=98.64952850341797, "p_A1"=7.3325419425964355}, {"timer"=10544.837890625, "p_A"=98.45421600341797, "p_A1"=7.3325419425964355}, {"timer"=10544.73828125, "p_A"=98.62999725341797, "p_A1"=7.3325419425964355}, {"timer"=10544.638671875, "p_A"=98.74718475341797, "p_A1"=7.3325419425964355}, {"timer"=10544.5390625, "p_A"=98.33702850341797, "p_A1"=7.3325419425964355}, {"timer"=10544.439453125, "p_A"=98.57140350341797, "p_A1"=7.3325419425964355}, {"timer"=10544.337890625, "p_A"=98.70812225341797, "p_A1"=7.3325419425964355}, {"timer"=10544.23828125, "p_A"=98.51280975341797, "p_A1"=7.3325419425964355}, {"timer"=10544.138671875, "p_A"=98.84484100341797, "p_A1"=7.3325419425964355}, {"timer"=10544.0390625, "p_A"=98.59093475341797, "p_A1"=7.3325419425964355}, {"timer"=10543.939453125, "p_A"=98.47374725341797, "p_A1"=7.3325419425964355}, {"timer"=10543.837890625, "p_A"=98.59093475341797, "p_A1"=7.3325419425964355}, {"timer"=10543.73828125, "p_A"=98.53234100341797, "p_A1"=7.3325419425964355}, {"timer"=10543.638671875, "p_A"=98.39562225341797, "p_A1"=7.3325419425964355}, {"timer"=10543.5390625, "p_A"=98.55187225341797, "p_A1"=7.3325419425964355}, {"timer"=10543.439453125, "p_A"=98.49327850341797, "p_A1"=7.3325419425964355}, {"timer"=10543.337890625, "p_A"=98.55187225341797, "p_A1"=7.3325419425964355}, {"timer"=10543.23828125, "p_A"=98.57140350341797, "p_A1"=7.3325419425964355}, {"timer"=10543.138671875, "p_A"=98.55187225341797, "p_A1"=7.3325419425964355}, {"timer"=10543.0390625, "p_A"=98.62999725341797, "p_A1"=7.3325419425964355}, {"timer"=10542.939453125, "p_A"=98.86437225341797, "p_A1"=7.3325419425964355}, {"timer"=10542.837890625, "p_A"=98.68859100341797, "p_A1"=7.3325419425964355}, {"timer"=10542.73828125, "p_A"=98.51280975341797, "p_A1"=7.3325419425964355}, {"timer"=10542.638671875, "p_A"=98.51280975341797, "p_A1"=7.3325419425964355}, {"timer"=10542.5390625, "p_A"=98.21984100341797, "p_A1"=7.3325419425964355}, {"timer"=10542.439453125, "p_A"=98.62999725341797, "p_A1"=7.3325419425964355}, {"timer"=10542.337890625, "p_A"=98.43468475341797, "p_A1"=7.3325419425964355}, {"timer"=10542.23828125, "p_A"=98.35655975341797, "p_A1"=7.3325419425964355}, {"timer"=10542.138671875, "p_A"=98.61046600341797, "p_A1"=7.3325419425964355}, {"timer"=10542.0390625, "p_A"=98.45421600341797, "p_A1"=7.3325419425964355}, {"timer"=10541.939453125, "p_A"=98.37609100341797, "p_A1"=7.3325419425964355}, {"timer"=10541.837890625, "p_A"=98.55187225341797, "p_A1"=7.3325419425964355}, {"timer"=10541.73828125, "p_A"=98.49327850341797, "p_A1"=7.3325419425964355}, {"timer"=10541.638671875, "p_A"=98.39562225341797, "p_A1"=7.3325419425964355}, {"timer"=10541.5390625, "p_A"=98.53234100341797, "p_A1"=7.3325419425964355}, {"timer"=10541.439453125, "p_A"=98.66905975341797, "p_A1"=7.3325419425964355}, {"timer"=10541.337890625, "p_A"=98.39562225341797, "p_A1"=7.3325419425964355}, {"timer"=10541.23828125, "p_A"=98.55187225341797, "p_A1"=7.3325419425964355}, {"timer"=10541.138671875, "p_A"=98.20030975341797, "p_A1"=7.3325419425964355}, {"timer"=10541.0390625, "p_A"=98.45421600341797, "p_A1"=7.3325419425964355}, {"timer"=10540.939453125, "p_A"=98.39562225341797, "p_A1"=7.3325419425964355}, {"timer"=10540.837890625, "p_A"=98.49327850341797, "p_A1"=7.3325419425964355}, {"timer"=10540.73828125, "p_A"=98.51280975341797, "p_A1"=7.3325419425964355}, {"timer"=10540.638671875, "p_A"=98.47374725341797, "p_A1"=7.3325419425964355}, {"timer"=10540.5390625, "p_A"=98.27843475341797, "p_A1"=7.3325419425964355}, {"timer"=10540.439453125, "p_A"=98.55187225341797, "p_A1"=7.3325419425964355}, {"timer"=10540.337890625, "p_A"=98.49327850341797, "p_A1"=7.3325419425964355}, {"timer"=10540.23828125, "p_A"=98.41515350341797, "p_A1"=7.3325419425964355}, {"timer"=10540.138671875, "p_A"=98.59093475341797, "p_A1"=7.3325419425964355}, {"timer"=10540.0390625, "p_A"=98.57140350341797, "p_A1"=7.3325419425964355}]}, ...(3 in all)]
  out "Strain":T5(graph)
  out "l_cyl":T6(graph)
  out "l_cyl_dot":T5(graph)
  out "Q_B":T7(graph)
  out "Valves":T8(graph)
  out "p_A_p_B":cluster{"timer":sgl, "p_A":sgl, "p_A1":sgl}[](array[cluster])=[{"timer"=10600.039, "p_A"=21.169062, "p_A1"=-0.41861194}, {"timer"=10599.939, "p_A"=21.208124, "p_A1"=-0.37716192}, {"timer"=10599.859, "p_A"=20.97375, "p_A1"=-0.3357119}, {"timer"=10599.758, "p_A"=20.700312, "p_A1"=-0.25281188}, {"timer"=10599.658, "p_A"=20.52453, "p_A1"=-0.2942619}, {"timer"=10599.559, "p_A"=20.856562, "p_A1"=-0.25281188}, {"timer"=10599.439, "p_A"=20.505, "p_A1"=-0.25281188}, {"timer"=10599.338, "p_A"=20.05578, "p_A1"=-0.21136184}, {"timer"=10599.258, "p_A"=19.587032, "p_A1"=-0.2942619}, {"timer"=10599.158, "p_A"=19.743282, "p_A1"=-0.12846181}, {"timer"=10599.059, "p_A"=19.450314, "p_A1"=-0.25281188}, {"timer"=10598.959, "p_A"=19.333126, "p_A1"=-0.21136184}, {"timer"=10598.838, "p_A"=18.630001, "p_A1"=-0.25281188}, {"timer"=10598.738, "p_A"=18.864376, "p_A1"=-0.3357119}, {"timer"=10598.639, "p_A"=18.239376, "p_A1"=-0.25281188}, {"timer"=10598.559, "p_A"=18.14172, "p_A1"=-0.25281188}, {"timer"=10598.459, "p_A"=17.712032, "p_A1"=-0.3357119}, {"timer"=10598.359, "p_A"=17.477657, "p_A1"=-0.2942619}, {"timer"=10598.238, "p_A"=17.380001, "p_A1"=-0.21136184}, {"timer"=10598.139, "p_A"=17.145626, "p_A1"=-0.41861194}, {"timer"=10598.059, "p_A"=16.89172, "p_A1"=-0.3357119}, {"timer"=10597.959, "p_A"=16.520626, "p_A1"=-0.37716192}, {"timer"=10597.859, "p_A"=16.383907, "p_A1"=-0.37716192}, {"timer"=10597.758, "p_A"=15.934688, "p_A1"=-0.41861194}, {"timer"=10597.658, "p_A"=15.778438, "p_A1"=-0.41861194}, {"timer"=10597.559, "p_A"=15.524531, "p_A1"=-0.2942619}, {"timer"=10597.459, "p_A"=15.231563, "p_A1"=-0.2942619}, {"timer"=10597.359, "p_A"=15.172969, "p_A1"=-0.41861194}, {"timer"=10597.238, "p_A"=14.684688, "p_A1"=-0.25281188}, {"timer"=10597.158, "p_A"=14.294063, "p_A1"=-0.3357119}, {"timer"=10597.059, "p_A"=14.294063, "p_A1"=-0.2942619}, {"timer"=10596.959, "p_A"=13.688594, "p_A1"=-0.2942619}, {"timer"=10596.859, "p_A"=13.766719, "p_A1"=-0.2942619}, {"timer"=10596.758, "p_A"=13.571406, "p_A1"=-0.37716192}, {"timer"=10596.658, "p_A"=13.180781, "p_A1"=-0.2942619}, {"timer"=10596.559, "p_A"=12.809688, "p_A1"=-0.21136184}, {"timer"=10596.459, "p_A"=12.653438, "p_A1"=-0.25281188}, {"timer"=10596.359, "p_A"=12.477656, "p_A1"=-0.25281188}, {"timer"=10596.258, "p_A"=12.008906, "p_A1"=-0.21136184}, {"timer"=10596.158, "p_A"=12.008906, "p_A1"=-0.2942619}, {"timer"=10596.059, "p_A"=11.364375, "p_A1"=-0.25281188}, {"timer"=10595.939, "p_A"=11.208125, "p_A1"=-0.25281188}, {"timer"=10595.859, "p_A"=10.8175, "p_A1"=-0.25281188}, {"timer"=10595.758, "p_A"=10.505, "p_A1"=-0.3357119}, {"timer"=10595.658, "p_A"=10.66125, "p_A1"=-0.2942619}, {"timer"=10595.539, "p_A"=9.919063, "p_A1"=-0.3357119}, {"timer"=10595.459, "p_A"=10.055781, "p_A1"=-0.46006197}, {"timer"=10595.359, "p_A"=9.5675, "p_A1"=-0.2942619}, {"timer"=10595.258, "p_A"=9.274531, "p_A1"=-0.3357119}, {"timer"=10595.158, "p_A"=9.020625, "p_A1"=-0.25281188}, {"timer"=10595.039, "p_A"=8.981563, "p_A1"=-0.3357119}, {"timer"=10594.959, "p_A"=8.766719, "p_A1"=-0.2942619}, {"timer"=10594.859, "p_A"=8.044063, "p_A1"=-0.37716192}, {"timer"=10594.758, "p_A"=7.9854684, "p_A1"=-0.2942619}, {"timer"=10594.658, "p_A"=7.809687, "p_A1"=-0.2942619}, {"timer"=10594.559, "p_A"=7.399531, "p_A1"=-0.41861194}, {"timer"=10594.459, "p_A"=7.2823434, "p_A1"=-0.25281188}, {"timer"=10594.359, "p_A"=6.5792184, "p_A1"=-0.21136184}, {"timer"=10594.238, "p_A"=6.5206246, "p_A1"=-0.3357119}, {"timer"=10594.139, "p_A"=6.169062, "p_A1"=-0.37716192}, {"timer"=10594.059, "p_A"=5.993281, "p_A1"=-0.3357119}, {"timer"=10593.939, "p_A"=6.0323434, "p_A1"=-0.41861194}, {"timer"=10593.838, "p_A"=5.4854684, "p_A1"=-0.3357119}, {"timer"=10593.758, "p_A"=5.368281, "p_A1"=-0.2942619}, {"timer"=10593.658, "p_A"=4.938594, "p_A1"=-0.37716192}, {"timer"=10593.539, "p_A"=4.5284376, "p_A1"=-0.3357119}, {"timer"=10593.439, "p_A"=4.5284376, "p_A1"=-0.37716192}, {"timer"=10593.338, "p_A"=4.0401564, "p_A1"=-0.37716192}, {"timer"=10593.258, "p_A"=3.8839064, "p_A1"=-0.3357119}, {"timer"=10593.158, "p_A"=3.4542189, "p_A1"=-0.25281188}, {"timer"=10593.059, "p_A"=2.8878126, "p_A1"=-0.25281188}, {"timer"=10592.939, "p_A"=2.770625, "p_A1"=-0.2942619}, {"timer"=10592.859, "p_A"=2.4190626, "p_A1"=-0.41861194}, {"timer"=10592.758, "p_A"=2.1065626, "p_A1"=-0.37716192}, {"timer"=10592.658, "p_A"=2.0870314, "p_A1"=-0.3357119}, {"timer"=10592.539, "p_A"=1.5987501, "p_A1"=-0.3357119}, {"timer"=10592.459, "p_A"=1.0714062, "p_A1"=-0.2942619}, {"timer"=10592.359, "p_A"=0.8565625, "p_A1"=-0.2942619}, {"timer"=10592.258, "p_A"=0.075312495, "p_A1"=-0.41861194}, {"timer"=10592.158, "p_A"=-0.002812501, "p_A1"=-0.50151205}, {"timer"=10592.059, "p_A"=0.6221875, "p_A1"=-0.37716192}, {"timer"=10591.959, "p_A"=12.38, "p_A1"=-0.2942619}, {"timer"=10591.859, "p_A"=45.07531, "p_A1"=-0.2942619}, {"timer"=10591.758, "p_A"=45.602654, "p_A1"=-0.25281188}, {"timer"=10591.639, "p_A"=46.208122, "p_A1"=-0.41861194}, {"timer"=10591.559, "p_A"=64.8214, "p_A1"=-0.16991183}, {"timer"=10591.439, "p_A"=96.403435, "p_A1"=1.405189}, {"timer"=10591.338, "p_A"=96.32531, "p_A1"=1.6124392}, {"timer"=10591.258, "p_A"=88.02453, "p_A1"=1.6538892}, {"timer"=10591.158, "p_A"=90.11437, "p_A1"=1.6953392}, {"timer"=10591.039, "p_A"=100.99328, "p_A1"=3.8921902}, {"timer"=10590.939, "p_A"=90.21203, "p_A1"=4.472491}, {"timer"=10590.838, "p_A"=83.98156, "p_A1"=4.9698906}, {"timer"=10590.758, "p_A"=99.46984, "p_A1"=5.011341}, {"timer"=10590.658, "p_A"=99.46984, "p_A1"=5.177141}, {"timer"=10590.559, "p_A"=99.64562, "p_A1"=5.0942407}, {"timer"=10590.439, "p_A"=99.5675, "p_A1"=5.218591}, {"timer"=10590.359, "p_A"=99.45031, "p_A1"=5.052791}, {"timer"=10590.258, "p_A"=99.60656, "p_A1"=5.1356907}, {"timer"=10590.158, "p_A"=99.45031, "p_A1"=5.0942407}, {"timer"=10590.039, "p_A"=99.62609, "p_A1"=5.2600408}, {"timer"=10589.939, "p_A"=99.62609, "p_A1"=5.1356907}, {"timer"=10589.838, "p_A"=99.64562, "p_A1"=5.218591}, {"timer"=10589.738, "p_A"=99.46984, "p_A1"=5.177141}, {"timer"=10589.658, "p_A"=99.60656, "p_A1"=5.177141}, {"timer"=10589.539, "p_A"=99.64562, "p_A1"=5.218591}, {"timer"=10589.459, "p_A"=99.66515, "p_A1"=5.301491}, {"timer"=10589.359, "p_A"=99.5089, "p_A1"=5.3429413}, {"timer"=10589.238, "p_A"=99.5089, "p_A1"=5.218591}, {"timer"=10589.158, "p_A"=99.48937, "p_A1"=5.2600408}, {"timer"=10589.059, "p_A"=99.45031, "p_A1"=5.2600408}, {"timer"=10588.959, "p_A"=99.29406, "p_A1"=5.301491}, {"timer"=10588.859, "p_A"=99.35265, "p_A1"=5.301491}, {"timer"=10588.758, "p_A"=99.528435, "p_A1"=5.2600408}, {"timer"=10588.658, "p_A"=99.391716, "p_A1"=5.3429413}, {"timer"=10588.559, "p_A"=99.76281, "p_A1"=5.3843913}, {"timer"=10588.439, "p_A"=99.48937, "p_A1"=5.3843913}, {"timer"=10588.359, "p_A"=99.5089, "p_A1"=5.3429413}, {"timer"=10588.258, "p_A"=99.5089, "p_A1"=5.425841}, {"timer"=10588.158, "p_A"=99.391716, "p_A1"=5.3843913}, {"timer"=10588.039, "p_A"=99.41125, "p_A1"=5.3429413}, {"timer"=10587.939, "p_A"=99.48937, "p_A1"=5.467291}, {"timer"=10587.859, "p_A"=99.46984, "p_A1"=5.425841}, {"timer"=10587.758, "p_A"=99.43078, "p_A1"=5.5087414}, {"timer"=10587.639, "p_A"=99.60656, "p_A1"=5.467291}, {"timer"=10587.559, "p_A"=99.41125, "p_A1"=5.425841}, {"timer"=10587.459, "p_A"=99.5675, "p_A1"=5.3843913}, {"timer"=10587.338, "p_A"=99.17687, "p_A1"=5.5087414}, {"timer"=10587.238, "p_A"=99.5675, "p_A1"=5.5087414}, {"timer"=10587.158, "p_A"=99.547966, "p_A1"=5.5087414}, {"timer"=10587.059, "p_A"=99.45031, "p_A1"=5.467291}, {"timer"=10586.959, "p_A"=99.5089, "p_A1"=5.467291}, {"timer"=10586.859, "p_A"=99.547966, "p_A1"=5.467291}, {"timer"=10586.758, "p_A"=99.45031, "p_A1"=5.5087414}, {"timer"=10586.658, "p_A"=99.46984, "p_A1"=5.5087414}, {"timer"=10586.559, "p_A"=99.547966, "p_A1"=5.591641}, {"timer"=10586.459, "p_A"=99.45031, "p_A1"=5.7159915}, {"timer"=10586.359, "p_A"=99.48937, "p_A1"=5.7159915}, {"timer"=10586.258, "p_A"=99.255, "p_A1"=5.591641}, {"timer"=10586.158, "p_A"=99.860466, "p_A1"=5.5501914}, {"timer"=10586.059, "p_A"=99.35265, "p_A1"=5.633091}, {"timer"=10585.959, "p_A"=99.547966, "p_A1"=5.591641}, {"timer"=10585.859, "p_A"=99.31359, "p_A1"=5.5501914}, {"timer"=10585.758, "p_A"=99.391716, "p_A1"=5.7159915}, {"timer"=10585.658, "p_A"=99.372185, "p_A1"=5.757441}, {"timer"=10585.559, "p_A"=99.372185, "p_A1"=5.633091}, {"timer"=10585.459, "p_A"=99.215935, "p_A1"=5.6745415}, {"timer"=10585.359, "p_A"=99.235466, "p_A1"=5.6745415}, {"timer"=10585.258, "p_A"=99.43078, "p_A1"=5.7159915}, {"timer"=10585.158, "p_A"=99.372185, "p_A1"=5.757441}, {"timer"=10585.059, "p_A"=99.547966, "p_A1"=5.757441}, {"timer"=10584.959, "p_A"=99.45031, "p_A1"=5.798891}, {"timer"=10584.838, "p_A"=99.391716, "p_A1"=5.7159915}, {"timer"=10584.758, "p_A"=99.60656, "p_A1"=5.757441}, {"timer"=10584.658, "p_A"=99.48937, "p_A1"=5.798891}, {"timer"=10584.559, "p_A"=99.391716, "p_A1"=5.7159915}, {"timer"=10584.459, "p_A"=99.35265, "p_A1"=5.6745415}, {"timer"=10584.359, "p_A"=99.215935, "p_A1"=5.7159915}, {"timer"=10584.258, "p_A"=99.5089, "p_A1"=5.798891}, {"timer"=10584.158, "p_A"=99.58703, "p_A1"=5.8403416}, {"timer"=10584.059, "p_A"=99.391716, "p_A1"=5.8817916}, {"timer"=10583.959, "p_A"=99.5089, "p_A1"=5.8817916}, {"timer"=10583.859, "p_A"=99.41125, "p_A1"=5.9232416}, {"timer"=10583.758, "p_A"=99.33312, "p_A1"=5.8403416}, {"timer"=10583.658, "p_A"=99.33312, "p_A1"=5.8403416}, {"timer"=10583.559, "p_A"=99.528435, "p_A1"=5.9232416}, {"timer"=10583.459, "p_A"=99.33312, "p_A1"=5.8403416}, {"timer"=10583.359, "p_A"=99.528435, "p_A1"=6.0061417}, {"timer"=10583.258, "p_A"=99.72375, "p_A1"=5.964691}, {"timer"=10583.158, "p_A"=99.48937, "p_A1"=6.0061417}, {"timer"=10583.059, "p_A"=99.41125, "p_A1"=6.0061417}, {"timer"=10582.959, "p_A"=99.45031, "p_A1"=6.0061417}, {"timer"=10582.859, "p_A"=99.43078, "p_A1"=5.964691}, {"timer"=10582.758, "p_A"=99.41125, "p_A1"=6.0061417}, {"timer"=10582.658, "p_A"=99.372185, "p_A1"=6.0061417}, {"timer"=10582.559, "p_A"=99.41125, "p_A1"=5.964691}, {"timer"=10582.459, "p_A"=99.58703, "p_A1"=6.0061417}, {"timer"=10582.359, "p_A"=99.372185, "p_A1"=6.0475917}, {"timer"=10582.258, "p_A"=99.5089, "p_A1"=6.0890417}, {"timer"=10582.158, "p_A"=99.35265, "p_A1"=6.0890417}, {"timer"=10582.039, "p_A"=99.60656, "p_A1"=6.0475917}, {"timer"=10581.959, "p_A"=99.76281, "p_A1"=6.0890417}, {"timer"=10581.838, "p_A"=99.43078, "p_A1"=6.0061417}, {"timer"=10581.738, "p_A"=99.372185, "p_A1"=6.1304913}, {"timer"=10581.658, "p_A"=99.27453, "p_A1"=6.0890417}, {"timer"=10581.559, "p_A"=99.48937, "p_A1"=6.254842}, {"timer"=10581.459, "p_A"=99.46984, "p_A1"=6.1719418}, {"timer"=10581.359, "p_A"=99.33312, "p_A1"=6.213392}, {"timer"=10581.238, "p_A"=99.255, "p_A1"=6.213392}, {"timer"=10581.158, "p_A"=99.58703, "p_A1"=6.2962914}, {"timer"=10581.059, "p_A"=99.31359, "p_A1"=6.2962914}, {"timer"=10580.959, "p_A"=99.372185, "p_A1"=6.213392}, {"timer"=10580.859, "p_A"=99.255, "p_A1"=6.379192}, {"timer"=10580.758, "p_A"=99.27453, "p_A1"=6.379192}, {"timer"=10580.658, "p_A"=99.41125, "p_A1"=6.379192}, {"timer"=10580.559, "p_A"=99.62609, "p_A1"=6.4620914}, {"timer"=10580.459, "p_A"=99.35265, "p_A1"=6.337742}, {"timer"=10580.359, "p_A"=99.29406, "p_A1"=6.4620914}, {"timer"=10580.258, "p_A"=99.09875, "p_A1"=6.420642}, {"timer"=10580.158, "p_A"=99.391716, "p_A1"=6.379192}, {"timer"=10580.059, "p_A"=99.33312, "p_A1"=6.420642}, {"timer"=10579.939, "p_A"=99.391716, "p_A1"=6.544992}, {"timer"=10579.838, "p_A"=99.29406, "p_A1"=6.586442}, {"timer"=10579.758, "p_A"=99.17687, "p_A1"=6.544992}, {"timer"=10579.658, "p_A"=99.48937, "p_A1"=6.586442}, {"timer"=10579.559, "p_A"=99.235466, "p_A1"=6.503542}, {"timer"=10579.439, "p_A"=99.33312, "p_A1"=6.4620914}, {"timer"=10579.338, "p_A"=99.215935, "p_A1"=6.586442}, {"timer"=10579.238, "p_A"=99.60656, "p_A1"=6.544992}, {"timer"=10579.139, "p_A"=99.391716, "p_A1"=6.544992}, {"timer"=10579.039, "p_A"=99.46984, "p_A1"=6.4620914}, {"timer"=10578.939, "p_A"=99.33312, "p_A1"=6.503542}, {"timer"=10578.838, "p_A"=99.215935, "p_A1"=6.544992}, {"timer"=10578.738, "p_A"=99.35265, "p_A1"=6.586442}, {"timer"=10578.639, "p_A"=99.31359, "p_A1"=6.503542}, {"timer"=10578.539, "p_A"=99.1964, "p_A1"=6.544992}, {"timer"=10578.439, "p_A"=99.684685, "p_A1"=6.6278915}, {"timer"=10578.338, "p_A"=99.079216, "p_A1"=6.503542}, {"timer"=10578.238, "p_A"=99.29406, "p_A1"=6.6278915}, {"timer"=10578.139, "p_A"=99.41125, "p_A1"=6.669342}, {"timer"=10578.039, "p_A"=99.547966, "p_A1"=6.669342}, {"timer"=10577.939, "p_A"=99.15734, "p_A1"=6.6278915}, {"timer"=10577.838, "p_A"=99.33312, "p_A1"=6.6278915}, {"timer"=10577.738, "p_A"=99.45031, "p_A1"=6.586442}, {"timer"=10577.639, "p_A"=99.1964, "p_A1"=6.669342}, {"timer"=10577.539, "p_A"=99.17687, "p_A1"=6.6278915}, {"timer"=10577.439, "p_A"=99.29406, "p_A1"=6.669342}, {"timer"=10577.338, "p_A"=99.372185, "p_A1"=6.669342}, {"timer"=10577.238, "p_A"=99.45031, "p_A1"=6.669342}, {"timer"=10577.139, "p_A"=99.372185, "p_A1"=6.752242}, {"timer"=10577.039, "p_A"=99.46984, "p_A1"=6.752242}, {"timer"=10576.939, "p_A"=99.27453, "p_A1"=6.835142}, {"timer"=10576.838, "p_A"=99.1964, "p_A1"=6.7936916}, {"timer"=10576.738, "p_A"=99.29406, "p_A1"=6.752242}, {"timer"=10576.639, "p_A"=99.29406, "p_A1"=6.7936916}, {"timer"=10576.539, "p_A"=99.09875, "p_A1"=6.7936916}, {"timer"=10576.439, "p_A"=99.215935, "p_A1"=6.918042}, {"timer"=10576.338, "p_A"=99.255, "p_A1"=6.835142}, {"timer"=10576.238, "p_A"=99.255, "p_A1"=6.752242}, {"timer"=10576.139, "p_A"=99.235466, "p_A1"=6.835142}, {"timer"=10576.039, "p_A"=99.09875, "p_A1"=6.876592}, {"timer"=10575.939, "p_A"=99.35265, "p_A1"=6.918042}, {"timer"=10575.838, "p_A"=99.29406, "p_A1"=6.7936916}, {"timer"=10575.738, "p_A"=99.33312, "p_A1"=6.876592}, {"timer"=10575.639, "p_A"=99.45031, "p_A1"=6.835142}, {"timer"=10575.539, "p_A"=99.29406, "p_A1"=6.876592}, {"timer"=10575.439, "p_A"=99.17687, "p_A1"=6.918042}, {"timer"=10575.338, "p_A"=99.11828, "p_A1"=6.9594917}, {"timer"=10575.238, "p_A"=99.13781, "p_A1"=6.876592}, {"timer"=10575.139, "p_A"=99.09875, "p_A1"=6.918042}, {"timer"=10575.039, "p_A"=99.391716, "p_A1"=6.918042}, {"timer"=10574.939, "p_A"=99.48937, "p_A1"=7.0423923}, {"timer"=10574.838, "p_A"=99.41125, "p_A1"=6.918042}, {"timer"=10574.738, "p_A"=99.45031, "p_A1"=6.918042}, {"timer"=10574.639, "p_A"=99.235466, "p_A1"=7.0009418}, {"timer"=10574.539, "p_A"=99.29406, "p_A1"=6.876592}, {"timer"=10574.439, "p_A"=99.35265, "p_A1"=6.876592}, {"timer"=10574.338, "p_A"=99.29406, "p_A1"=6.9594917}, {"timer"=10574.238, "p_A"=99.372185, "p_A1"=7.0423923}, {"timer"=10574.139, "p_A"=99.255, "p_A1"=7.0009418}, {"timer"=10574.039, "p_A"=99.255, "p_A1"=7.0009418}, {"timer"=10573.939, "p_A"=99.255, "p_A1"=6.9594917}, {"timer"=10573.838, "p_A"=99.372185, "p_A1"=7.0838423}, {"timer"=10573.738, "p_A"=99.235466, "p_A1"=7.0009418}, {"timer"=10573.639, "p_A"=99.17687, "p_A1"=7.0423923}, {"timer"=10573.539, "p_A"=99.33312, "p_A1"=7.0009418}, {"timer"=10573.439, "p_A"=99.1964, "p_A1"=7.0423923}, {"timer"=10573.338, "p_A"=99.33312, "p_A1"=7.125292}, {"timer"=10573.238, "p_A"=99.31359, "p_A1"=6.9594917}, {"timer"=10573.139, "p_A"=99.15734, "p_A1"=7.0009418}, {"timer"=10573.039, "p_A"=99.27453, "p_A1"=7.0009418}, {"timer"=10572.939, "p_A"=98.96203, "p_A1"=6.9594917}, {"timer"=10572.838, "p_A"=99.33312, "p_A1"=7.0838423}, {"timer"=10572.738, "p_A"=99.31359, "p_A1"=7.125292}, {"timer"=10572.639, "p_A"=99.27453, "p_A1"=7.0423923}, {"timer"=10572.539, "p_A"=99.15734, "p_A1"=7.0838423}, {"timer"=10572.439, "p_A"=99.33312, "p_A1"=7.0838423}, {"timer"=10572.338, "p_A"=99.31359, "p_A1"=7.0423923}, {"timer"=10572.238, "p_A"=99.255, "p_A1"=7.0838423}, {"timer"=10572.139, "p_A"=99.48937, "p_A1"=7.0838423}, {"timer"=10572.039, "p_A"=99.215935, "p_A1"=7.0838423}, {"timer"=10571.939, "p_A"=98.96203, "p_A1"=7.0838423}, {"timer"=10571.838, "p_A"=99.255, "p_A1"=7.0423923}, {"timer"=10571.738, "p_A"=99.17687, "p_A1"=7.125292}, {"timer"=10571.639, "p_A"=99.31359, "p_A1"=7.125292}, {"timer"=10571.539, "p_A"=99.13781, "p_A1"=7.166742}, {"timer"=10571.439, "p_A"=99.41125, "p_A1"=7.0838423}, {"timer"=10571.338, "p_A"=99.391716, "p_A1"=7.166742}, {"timer"=10571.238, "p_A"=99.09875, "p_A1"=7.125292}, {"timer"=10571.139, "p_A"=99.31359, "p_A1"=7.125292}, {"timer"=10571.039, "p_A"=99.09875, "p_A1"=7.0009418}, {"timer"=10570.939, "p_A"=99.255, "p_A1"=7.166742}, {"timer"=10570.838, "p_A"=99.1964, "p_A1"=7.0423923}, {"timer"=10570.738, "p_A"=99.255, "p_A1"=7.0838423}, {"timer"=10570.639, "p_A"=99.1964, "p_A1"=7.166742}, {"timer"=10570.539, "p_A"=99.255, "p_A1"=7.125292}, {"timer"=10570.439, "p_A"=99.215935, "p_A1"=7.166742}, {"timer"=10570.338, "p_A"=99.31359, "p_A1"=7.125292}, {"timer"=10570.238, "p_A"=99.11828, "p_A1"=7.0838423}, {"timer"=10570.139, "p_A"=99.35265, "p_A1"=7.0838423}, {"timer"=10570.039, "p_A"=99.35265, "p_A1"=7.125292}, {"timer"=10569.939, "p_A"=99.391716, "p_A1"=7.125292}, {"timer"=10569.838, "p_A"=98.922966, "p_A1"=7.2081923}, {"timer"=10569.738, "p_A"=99.00109, "p_A1"=7.166742}, {"timer"=10569.639, "p_A"=98.96203, "p_A1"=7.125292}, {"timer"=10569.539, "p_A"=99.04015, "p_A1"=7.125292}, {"timer"=10569.439, "p_A"=99.079216, "p_A1"=7.166742}, {"timer"=10569.338, "p_A"=99.17687, "p_A1"=7.125292}, {"timer"=10569.238, "p_A"=99.17687, "p_A1"=7.125292}, {"timer"=10569.139, "p_A"=99.11828, "p_A1"=7.166742}, {"timer"=10569.039, "p_A"=99.13781, "p_A1"=7.0838423}, {"timer"=10568.939, "p_A"=99.02062, "p_A1"=7.166742}, {"timer"=10568.838, "p_A"=99.13781, "p_A1"=7.166742}, {"timer"=10568.738, "p_A"=99.059685, "p_A1"=7.166742}, {"timer"=10568.639, "p_A"=99.215935, "p_A1"=7.125292}, {"timer"=10568.539, "p_A"=99.215935, "p_A1"=7.166742}, {"timer"=10568.439, "p_A"=99.04015, "p_A1"=7.2081923}, {"timer"=10568.338, "p_A"=99.09875, "p_A1"=7.125292}, {"timer"=10568.238, "p_A"=99.215935, "p_A1"=7.125292}, {"timer"=10568.139, "p_A"=99.059685, "p_A1"=7.2081923}, {"timer"=10568.039, "p_A"=99.372185, "p_A1"=7.2081923}, {"timer"=10567.939, "p_A"=99.31359, "p_A1"=7.2081923}, {"timer"=10567.838, "p_A"=99.079216, "p_A1"=7.2081923}, {"timer"=10567.738, "p_A"=99.059685, "p_A1"=7.2081923}, {"timer"=10567.639, "p_A"=99.235466, "p_A1"=7.2496424}, {"timer"=10567.539, "p_A"=99.17687, "p_A1"=7.2496424}, {"timer"=10567.439, "p_A"=99.079216, "p_A1"=7.2081923}, {"timer"=10567.338, "p_A"=99.1964, "p_A1"=7.2081923}, {"timer"=10567.238, "p_A"=99.00109, "p_A1"=7.2081923}, {"timer"=10567.139, "p_A"=99.02062, "p_A1"=7.2081923}, {"timer"=10567.039, "p_A"=99.1964, "p_A1"=7.2081923}, {"timer"=10566.939, "p_A"=99.35265, "p_A1"=7.2081923}, {"timer"=10566.838, "p_A"=98.9425, "p_A1"=7.2081923}, {"timer"=10566.738, "p_A"=99.27453, "p_A1"=7.2496424}, {"timer"=10566.639, "p_A"=98.86437, "p_A1"=7.166742}, {"timer"=10566.539, "p_A"=99.00109, "p_A1"=7.2496424}, {"timer"=10566.439, "p_A"=98.922966, "p_A1"=7.166742}, {"timer"=10566.338, "p_A"=99.15734, "p_A1"=7.166742}, {"timer"=10566.238, "p_A"=99.04015, "p_A1"=7.166742}, {"timer"=10566.139, "p_A"=99.35265, "p_A1"=7.2081923}, {"timer"=10566.039, "p_A"=99.09875, "p_A1"=7.2081923}, {"timer"=10565.939, "p_A"=99.13781, "p_A1"=7.2496424}, {"timer"=10565.838, "p_A"=99.17687, "p_A1"=7.2081923}, {"timer"=10565.738, "p_A"=99.35265, "p_A1"=7.2081923}, {"timer"=10565.639, "p_A"=99.15734, "p_A1"=7.2496424}, {"timer"=10565.539, "p_A"=99.27453, "p_A1"=7.2081923}, {"timer"=10565.439, "p_A"=98.9425, "p_A1"=7.2496424}, {"timer"=10565.338, "p_A"=99.04015, "p_A1"=7.2081923}, {"timer"=10565.238, "p_A"=99.11828, "p_A1"=7.2496424}, {"timer"=10565.139, "p_A"=98.98156, "p_A1"=7.2081923}, {"timer"=10565.039, "p_A"=99.02062, "p_A1"=7.2496424}, {"timer"=10564.939, "p_A"=99.31359, "p_A1"=7.2496424}, {"timer"=10564.838, "p_A"=99.079216, "p_A1"=7.2496424}, {"timer"=10564.738, "p_A"=99.215935, "p_A1"=7.2081923}, {"timer"=10564.639, "p_A"=99.27453, "p_A1"=7.291092}, {"timer"=10564.539, "p_A"=99.27453, "p_A1"=7.2496424}, {"timer"=10564.439, "p_A"=99.02062, "p_A1"=7.2496424}, {"timer"=10564.338, "p_A"=99.235466, "p_A1"=7.2496424}, {"timer"=10564.238, "p_A"=99.00109, "p_A1"=7.2496424}, {"timer"=10564.139, "p_A"=99.235466, "p_A1"=7.2496424}, {"timer"=10564.039, "p_A"=99.02062, "p_A1"=7.2496424}, {"timer"=10563.939, "p_A"=99.1964, "p_A1"=7.2496424}, {"timer"=10563.838, "p_A"=98.8839, "p_A1"=7.2496424}, {"timer"=10563.738, "p_A"=99.11828, "p_A1"=7.2081923}, {"timer"=10563.639, "p_A"=99.235466, "p_A1"=7.2496424}, {"timer"=10563.539, "p_A"=99.215935, "p_A1"=7.2496424}, {"timer"=10563.439, "p_A"=99.02062, "p_A1"=7.2496424}, {"timer"=10563.338, "p_A"=99.11828, "p_A1"=7.291092}, {"timer"=10563.238, "p_A"=99.02062, "p_A1"=7.2496424}, {"timer"=10563.139, "p_A"=98.8839, "p_A1"=7.2496424}, {"timer"=10563.039, "p_A"=99.13781, "p_A1"=7.291092}, {"timer"=10562.939, "p_A"=98.68859, "p_A1"=7.2496424}, {"timer"=10562.838, "p_A"=98.86437, "p_A1"=7.2496424}, {"timer"=10562.738, "p_A"=98.9425, "p_A1"=7.291092}, {"timer"=10562.639, "p_A"=99.04015, "p_A1"=7.2496424}, {"timer"=10562.539, "p_A"=99.00109, "p_A1"=7.2496424}, {"timer"=10562.439, "p_A"=98.84484, "p_A1"=7.2496424}, {"timer"=10562.338, "p_A"=99.079216, "p_A1"=7.2496424}, {"timer"=10562.238, "p_A"=99.02062, "p_A1"=7.291092}, {"timer"=10562.139, "p_A"=99.15734, "p_A1"=7.2496424}, {"timer"=10562.039, "p_A"=99.04015, "p_A1"=7.2496424}, {"timer"=10561.939, "p_A"=99.13781, "p_A1"=7.2496424}, {"timer"=10561.838, "p_A"=99.13781, "p_A1"=7.291092}, {"timer"=10561.738, "p_A"=99.215935, "p_A1"=7.291092}, {"timer"=10561.639, "p_A"=98.98156, "p_A1"=7.2496424}, {"timer"=10561.539, "p_A"=99.04015, "p_A1"=7.2496424}, {"timer"=10561.439, "p_A"=99.235466, "p_A1"=7.291092}, {"timer"=10561.338, "p_A"=98.8839, "p_A1"=7.2496424}, {"timer"=10561.238, "p_A"=99.17687, "p_A1"=7.291092}, {"timer"=10561.139, "p_A"=99.27453, "p_A1"=7.291092}, {"timer"=10561.039, "p_A"=99.11828, "p_A1"=7.2496424}, {"timer"=10560.939, "p_A"=98.80578, "p_A1"=7.2496424}, {"timer"=10560.838, "p_A"=99.17687, "p_A1"=7.2496424}, {"timer"=10560.738, "p_A"=99.17687, "p_A1"=7.291092}, {"timer"=10560.639, "p_A"=99.059685, "p_A1"=7.2496424}, {"timer"=10560.539, "p_A"=99.04015, "p_A1"=7.2496424}, {"timer"=10560.439, "p_A"=99.04015, "p_A1"=7.2496424}, {"timer"=10560.338, "p_A"=99.13781, "p_A1"=7.291092}, {"timer"=10560.238, "p_A"=98.9425, "p_A1"=7.2496424}, {"timer"=10560.139, "p_A"=99.02062, "p_A1"=7.291092}, {"timer"=10560.039, "p_A"=99.04015, "p_A1"=7.2496424}, {"timer"=10559.939, "p_A"=99.09875, "p_A1"=7.2496424}, {"timer"=10559.838, "p_A"=98.82531, "p_A1"=7.291092}, {"timer"=10559.738, "p_A"=98.922966, "p_A1"=7.291092}, {"timer"=10559.639, "p_A"=98.98156, "p_A1"=7.2496424}, {"timer"=10559.539, "p_A"=98.766716, "p_A1"=7.2496424}, {"timer"=10559.439, "p_A"=99.079216, "p_A1"=7.291092}, {"timer"=10559.338, "p_A"=98.98156, "p_A1"=7.291092}, {"timer"=10559.238, "p_A"=99.04015, "p_A1"=7.291092}, {"timer"=10559.139, "p_A"=99.00109, "p_A1"=7.2496424}, {"timer"=10559.039, "p_A"=98.96203, "p_A1"=7.291092}, {"timer"=10558.939, "p_A"=99.13781, "p_A1"=7.291092}, {"timer"=10558.838, "p_A"=98.922966, "p_A1"=7.291092}, {"timer"=10558.738, "p_A"=98.82531, "p_A1"=7.291092}, {"timer"=10558.619, "p_A"=99.059685, "p_A1"=7.291092}, {"timer"=10558.539, "p_A"=98.8839, "p_A1"=7.291092}, {"timer"=10558.439, "p_A"=98.922966, "p_A1"=7.291092}, {"timer"=10558.338, "p_A"=98.96203, "p_A1"=7.291092}, {"timer"=10558.219, "p_A"=98.68859, "p_A1"=7.291092}, {"timer"=10558.139, "p_A"=98.922966, "p_A1"=7.291092}, {"timer"=10558.039, "p_A"=98.96203, "p_A1"=7.291092}, {"timer"=10557.939, "p_A"=98.8839, "p_A1"=7.2496424}, {"timer"=10557.838, "p_A"=98.9425, "p_A1"=7.291092}, {"timer"=10557.738, "p_A"=99.15734, "p_A1"=7.291092}, {"timer"=10557.639, "p_A"=99.079216, "p_A1"=7.291092}, {"timer"=10557.539, "p_A"=99.09875, "p_A1"=7.291092}, {"timer"=10557.439, "p_A"=98.82531, "p_A1"=7.291092}, {"timer"=10557.338, "p_A"=98.903435, "p_A1"=7.291092}, {"timer"=10557.238, "p_A"=98.96203, "p_A1"=7.291092}, {"timer"=10557.139, "p_A"=99.079216, "p_A1"=7.291092}, {"timer"=10557.039, "p_A"=98.766716, "p_A1"=7.291092}, {"timer"=10556.939, "p_A"=99.02062, "p_A1"=7.291092}, {"timer"=10556.838, "p_A"=99.00109, "p_A1"=7.291092}, {"timer"=10556.738, "p_A"=98.922966, "p_A1"=7.291092}, {"timer"=10556.639, "p_A"=98.66906, "p_A1"=7.291092}, {"timer"=10556.539, "p_A"=98.80578, "p_A1"=7.291092}, {"timer"=10556.439, "p_A"=98.922966, "p_A1"=7.291092}, {"timer"=10556.338, "p_A"=99.02062, "p_A1"=7.291092}, {"timer"=10556.219, "p_A"=98.922966, "p_A1"=7.291092}, {"timer"=10556.139, "p_A"=98.903435, "p_A1"=7.291092}, {"timer"=10556.039, "p_A"=98.903435, "p_A1"=7.291092}, {"timer"=10555.939, "p_A"=98.747185, "p_A1"=7.291092}, {"timer"=10555.838, "p_A"=98.86437, "p_A1"=7.291092}, {"timer"=10555.738, "p_A"=99.09875, "p_A1"=7.291092}, {"timer"=10555.639, "p_A"=98.82531, "p_A1"=7.332542}, {"timer"=10555.539, "p_A"=98.610466, "p_A1"=7.291092}, {"timer"=10555.439, "p_A"=98.82531, "p_A1"=7.332542}, {"timer"=10555.338, "p_A"=98.80578, "p_A1"=7.291092}, {"timer"=10555.238, "p_A"=98.96203, "p_A1"=7.291092}, {"timer"=10555.139, "p_A"=98.82531, "p_A1"=7.291092}, {"timer"=10555.039, "p_A"=98.8839, "p_A1"=7.291092}, {"timer"=10554.939, "p_A"=98.68859, "p_A1"=7.291092}, {"timer"=10554.838, "p_A"=99.09875, "p_A1"=7.291092}, {"timer"=10554.738, "p_A"=98.80578, "p_A1"=7.291092}, {"timer"=10554.639, "p_A"=98.98156, "p_A1"=7.332542}, {"timer"=10554.539, "p_A"=98.8839, "p_A1"=7.291092}, {"timer"=10554.439, "p_A"=98.922966, "p_A1"=7.291092}, {"timer"=10554.338, "p_A"=98.766716, "p_A1"=7.332542}, {"timer"=10554.238, "p_A"=98.82531, "p_A1"=7.291092}, {"timer"=10554.139, "p_A"=98.8839, "p_A1"=7.291092}, {"timer"=10554.039, "p_A"=99.04015, "p_A1"=7.291092}, {"timer"=10553.939, "p_A"=99.1964, "p_A1"=7.291092}, {"timer"=10553.838, "p_A"=98.84484, "p_A1"=7.291092}, {"timer"=10553.738, "p_A"=99.079216, "p_A1"=7.291092}, {"timer"=10553.639, "p_A"=98.610466, "p_A1"=7.291092}, {"timer"=10553.539, "p_A"=98.80578, "p_A1"=7.291092}, {"timer"=10553.439, "p_A"=98.98156, "p_A1"=7.291092}, {"timer"=10553.338, "p_A"=98.82531, "p_A1"=7.291092}, {"timer"=10553.238, "p_A"=98.72765, "p_A1"=7.291092}, {"timer"=10553.139, "p_A"=99.04015, "p_A1"=7.291092}, {"timer"=10553.039, "p_A"=98.80578, "p_A1"=7.332542}, {"timer"=10552.939, "p_A"=98.610466, "p_A1"=7.291092}, {"timer"=10552.838, "p_A"=99.11828, "p_A1"=7.291092}, {"timer"=10552.738, "p_A"=98.922966, "p_A1"=7.291092}, {"timer"=10552.639, "p_A"=98.78625, "p_A1"=7.332542}, {"timer"=10552.539, "p_A"=98.86437, "p_A1"=7.291092}, {"timer"=10552.439, "p_A"=98.66906, "p_A1"=7.332542}, {"timer"=10552.338, "p_A"=98.922966, "p_A1"=7.291092}, {"timer"=10552.238, "p_A"=98.70812, "p_A1"=7.332542}, {"timer"=10552.139, "p_A"=98.78625, "p_A1"=7.332542}, {"timer"=10552.039, "p_A"=98.64953, "p_A1"=7.291092}, {"timer"=10551.939, "p_A"=98.98156, "p_A1"=7.291092}, {"timer"=10551.818, "p_A"=98.78625, "p_A1"=7.291092}, {"timer"=10551.738, "p_A"=98.434685, "p_A1"=7.332542}, {"timer"=10551.619, "p_A"=98.766716, "p_A1"=7.291092}, {"timer"=10551.539, "p_A"=98.68859, "p_A1"=7.291092}, {"timer"=10551.439, "p_A"=98.78625, "p_A1"=7.332542}, {"timer"=10551.338, "p_A"=98.922966, "p_A1"=7.332542}, {"timer"=10551.238, "p_A"=98.747185, "p_A1"=7.332542}, {"timer"=10551.139, "p_A"=98.610466, "p_A1"=7.332542}, {"timer"=10551.039, "p_A"=98.922966, "p_A1"=7.291092}, {"timer"=10550.939, "p_A"=98.8839, "p_A1"=7.291092}, {"timer"=10550.838, "p_A"=98.63, "p_A1"=7.291092}, {"timer"=10550.738, "p_A"=98.68859, "p_A1"=7.332542}, {"timer"=10550.639, "p_A"=98.84484, "p_A1"=7.332542}, {"timer"=10550.539, "p_A"=98.80578, "p_A1"=7.332542}, {"timer"=10550.439, "p_A"=98.78625, "p_A1"=7.291092}, {"timer"=10550.338, "p_A"=98.5714, "p_A1"=7.332542}, {"timer"=10550.238, "p_A"=98.766716, "p_A1"=7.291092}, {"timer"=10550.139, "p_A"=98.64953, "p_A1"=7.332542}, {"timer"=10550.039, "p_A"=98.590935, "p_A1"=7.332542}, {"timer"=10549.939, "p_A"=98.63, "p_A1"=7.332542}, {"timer"=10549.838, "p_A"=98.86437, "p_A1"=7.332542}, {"timer"=10549.738, "p_A"=98.78625, "p_A1"=7.332542}, {"timer"=10549.639, "p_A"=98.80578, "p_A1"=7.332542}, {"timer"=10549.539, "p_A"=98.590935, "p_A1"=7.332542}, {"timer"=10549.439, "p_A"=98.66906, "p_A1"=7.332542}, {"timer"=10549.338, "p_A"=98.610466, "p_A1"=7.291092}, {"timer"=10549.238, "p_A"=98.747185, "p_A1"=7.332542}, {"timer"=10549.139, "p_A"=98.84484, "p_A1"=7.332542}, {"timer"=10549.039, "p_A"=98.53234, "p_A1"=7.291092}, {"timer"=10548.939, "p_A"=98.747185, "p_A1"=7.332542}, {"timer"=10548.838, "p_A"=98.86437, "p_A1"=7.332542}, {"timer"=10548.738, "p_A"=98.766716, "p_A1"=7.332542}, {"timer"=10548.639, "p_A"=98.64953, "p_A1"=7.332542}, {"timer"=10548.539, "p_A"=98.68859, "p_A1"=7.332542}, {"timer"=10548.439, "p_A"=98.68859, "p_A1"=7.332542}, {"timer"=10548.338, "p_A"=98.610466, "p_A1"=7.332542}, {"timer"=10548.238, "p_A"=98.72765, "p_A1"=7.332542}, {"timer"=10548.139, "p_A"=98.72765, "p_A1"=7.332542}, {"timer"=10548.039, "p_A"=98.72765, "p_A1"=7.332542}, {"timer"=10547.939, "p_A"=98.68859, "p_A1"=7.332542}, {"timer"=10547.838, "p_A"=98.747185, "p_A1"=7.332542}, {"timer"=10547.738, "p_A"=98.84484, "p_A1"=7.332542}, {"timer"=10547.639, "p_A"=98.80578, "p_A1"=7.332542}, {"timer"=10547.539, "p_A"=98.766716, "p_A1"=7.332542}, {"timer"=10547.439, "p_A"=98.41515, "p_A1"=7.291092}, {"timer"=10547.338, "p_A"=98.39562, "p_A1"=7.332542}, {"timer"=10547.238, "p_A"=98.49328, "p_A1"=7.332542}, {"timer"=10547.139, "p_A"=98.747185, "p_A1"=7.332542}, {"timer"=10547.039, "p_A"=98.9425, "p_A1"=7.332542}, {"timer"=10546.939, "p_A"=98.80578, "p_A1"=7.332542}, {"timer"=10546.838, "p_A"=98.63, "p_A1"=7.332542}, {"timer"=10546.738, "p_A"=98.66906, "p_A1"=7.332542}, {"timer"=10546.639, "p_A"=98.434685, "p_A1"=7.332542}, {"timer"=10546.539, "p_A"=98.84484, "p_A1"=7.332542}, {"timer"=10546.439, "p_A"=98.747185, "p_A1"=7.332542}, {"timer"=10546.338, "p_A"=98.64953, "p_A1"=7.332542}, {"timer"=10546.238, "p_A"=98.63, "p_A1"=7.332542}, {"timer"=10546.139, "p_A"=98.63, "p_A1"=7.332542}, {"timer"=10546.039, "p_A"=98.63, "p_A1"=7.332542}, {"timer"=10545.939, "p_A"=98.72765, "p_A1"=7.332542}, {"timer"=10545.838, "p_A"=98.434685, "p_A1"=7.332542}, {"timer"=10545.738, "p_A"=98.5714, "p_A1"=7.332542}, {"timer"=10545.639, "p_A"=98.51281, "p_A1"=7.332542}, {"timer"=10545.539, "p_A"=98.49328, "p_A1"=7.332542}, {"timer"=10545.439, "p_A"=98.72765, "p_A1"=7.332542}, {"timer"=10545.338, "p_A"=98.610466, "p_A1"=7.332542}, {"timer"=10545.238, "p_A"=98.53234, "p_A1"=7.332542}, {"timer"=10545.139, "p_A"=98.5714, "p_A1"=7.332542}, {"timer"=10545.039, "p_A"=98.53234, "p_A1"=7.332542}, {"timer"=10544.939, "p_A"=98.64953, "p_A1"=7.332542}, {"timer"=10544.838, "p_A"=98.454216, "p_A1"=7.332542}, {"timer"=10544.738, "p_A"=98.63, "p_A1"=7.332542}, {"timer"=10544.639, "p_A"=98.747185, "p_A1"=7.332542}, {"timer"=10544.539, "p_A"=98.33703, "p_A1"=7.332542}, {"timer"=10544.439, "p_A"=98.5714, "p_A1"=7.332542}, {"timer"=10544.338, "p_A"=98.70812, "p_A1"=7.332542}, {"timer"=10544.238, "p_A"=98.51281, "p_A1"=7.332542}, {"timer"=10544.139, "p_A"=98.84484, "p_A1"=7.332542}, {"timer"=10544.039, "p_A"=98.590935, "p_A1"=7.332542}, {"timer"=10543.939, "p_A"=98.47375, "p_A1"=7.332542}, {"timer"=10543.838, "p_A"=98.590935, "p_A1"=7.332542}, {"timer"=10543.738, "p_A"=98.53234, "p_A1"=7.332542}, {"timer"=10543.639, "p_A"=98.39562, "p_A1"=7.332542}, {"timer"=10543.539, "p_A"=98.55187, "p_A1"=7.332542}, {"timer"=10543.439, "p_A"=98.49328, "p_A1"=7.332542}, {"timer"=10543.338, "p_A"=98.55187, "p_A1"=7.332542}, {"timer"=10543.238, "p_A"=98.5714, "p_A1"=7.332542}, {"timer"=10543.139, "p_A"=98.55187, "p_A1"=7.332542}, {"timer"=10543.039, "p_A"=98.63, "p_A1"=7.332542}, {"timer"=10542.939, "p_A"=98.86437, "p_A1"=7.332542}, {"timer"=10542.838, "p_A"=98.68859, "p_A1"=7.332542}, {"timer"=10542.738, "p_A"=98.51281, "p_A1"=7.332542}, {"timer"=10542.639, "p_A"=98.51281, "p_A1"=7.332542}, {"timer"=10542.539, "p_A"=98.21984, "p_A1"=7.332542}, {"timer"=10542.439, "p_A"=98.63, "p_A1"=7.332542}, {"timer"=10542.338, "p_A"=98.434685, "p_A1"=7.332542}, {"timer"=10542.238, "p_A"=98.35656, "p_A1"=7.332542}, {"timer"=10542.139, "p_A"=98.610466, "p_A1"=7.332542}, {"timer"=10542.039, "p_A"=98.454216, "p_A1"=7.332542}, {"timer"=10541.939, "p_A"=98.37609, "p_A1"=7.332542}, {"timer"=10541.838, "p_A"=98.55187, "p_A1"=7.332542}, {"timer"=10541.738, "p_A"=98.49328, "p_A1"=7.332542}, {"timer"=10541.639, "p_A"=98.39562, "p_A1"=7.332542}, {"timer"=10541.539, "p_A"=98.53234, "p_A1"=7.332542}, {"timer"=10541.439, "p_A"=98.66906, "p_A1"=7.332542}, {"timer"=10541.338, "p_A"=98.39562, "p_A1"=7.332542}, {"timer"=10541.238, "p_A"=98.55187, "p_A1"=7.332542}, {"timer"=10541.139, "p_A"=98.20031, "p_A1"=7.332542}, {"timer"=10541.039, "p_A"=98.454216, "p_A1"=7.332542}, {"timer"=10540.939, "p_A"=98.39562, "p_A1"=7.332542}, {"timer"=10540.838, "p_A"=98.49328, "p_A1"=7.332542}, {"timer"=10540.738, "p_A"=98.51281, "p_A1"=7.332542}, {"timer"=10540.639, "p_A"=98.47375, "p_A1"=7.332542}, {"timer"=10540.539, "p_A"=98.278435, "p_A1"=7.332542}, {"timer"=10540.439, "p_A"=98.55187, "p_A1"=7.332542}, {"timer"=10540.338, "p_A"=98.49328, "p_A1"=7.332542}, {"timer"=10540.238, "p_A"=98.41515, "p_A1"=7.332542}, {"timer"=10540.139, "p_A"=98.590935, "p_A1"=7.332542}, {"timer"=10540.039, "p_A"=98.5714, "p_A1"=7.332542}]
  out "p_A1_p_comp":cluster{"timer":sgl, "p_A":sgl, "p_A1":sgl}[](array[cluster])=[{"timer"=10600.039, "p_A"=21.637812, "p_A1"=0.15499994}, {"timer"=10599.939, "p_A"=21.637812, "p_A1"=0.03781244}, {"timer"=10599.859, "p_A"=21.383905, "p_A1"=0.03781244}, {"timer"=10599.758, "p_A"=21.266718, "p_A1"=-0.0012500584}, {"timer"=10599.658, "p_A"=20.895624, "p_A1"=0.07687494}, {"timer"=10599.559, "p_A"=20.876093, "p_A1"=0.13546869}, {"timer"=10599.439, "p_A"=20.329218, "p_A1"=0.03781244}, {"timer"=10599.338, "p_A"=20.446405, "p_A1"=0.07687494}, {"timer"=10599.258, "p_A"=20.05578, "p_A1"=0.03781244}, {"timer"=10599.158, "p_A"=19.880001, "p_A1"=0.03781244}, {"timer"=10599.059, "p_A"=19.606564, "p_A1"=0.03781244}, {"timer"=10598.959, "p_A"=19.333126, "p_A1"=-0.04031256}, {"timer"=10598.838, "p_A"=19.215939, "p_A1"=-0.0012500584}, {"timer"=10598.738, "p_A"=18.844845, "p_A1"=0.03781244}, {"timer"=10598.639, "p_A"=18.649532, "p_A1"=-0.020781308}, {"timer"=10598.559, "p_A"=18.45422, "p_A1"=0.07687494}, {"timer"=10598.459, "p_A"=18.239376, "p_A1"=0.018281192}, {"timer"=10598.359, "p_A"=17.98547, "p_A1"=0.018281192}, {"timer"=10598.238, "p_A"=17.67297, "p_A1"=-0.0012500584}, {"timer"=10598.139, "p_A"=17.438595, "p_A1"=0.07687494}, {"timer"=10598.059, "p_A"=17.04797, "p_A1"=0.05734369}, {"timer"=10597.959, "p_A"=16.89172, "p_A1"=0.018281192}, {"timer"=10597.859, "p_A"=16.833126, "p_A1"=-0.0012500584}, {"timer"=10597.758, "p_A"=16.42297, "p_A1"=0.07687494}, {"timer"=10597.658, "p_A"=15.993281, "p_A1"=-0.05984381}, {"timer"=10597.559, "p_A"=15.915156, "p_A1"=-0.0012500584}, {"timer"=10597.459, "p_A"=15.524531, "p_A1"=0.018281192}, {"timer"=10597.359, "p_A"=15.290156, "p_A1"=0.018281192}, {"timer"=10597.238, "p_A"=14.938594, "p_A1"=-0.04031256}, {"timer"=10597.158, "p_A"=14.5675, "p_A1"=-0.04031256}, {"timer"=10597.059, "p_A"=14.333125, "p_A1"=0.07687494}, {"timer"=10596.959, "p_A"=14.391719, "p_A1"=0.07687494}, {"timer"=10596.859, "p_A"=14.118281, "p_A1"=0.11593744}, {"timer"=10596.758, "p_A"=13.844844, "p_A1"=0.11593744}, {"timer"=10596.658, "p_A"=13.3175, "p_A1"=0.05734369}, {"timer"=10596.559, "p_A"=13.024531, "p_A1"=0.018281192}, {"timer"=10596.459, "p_A"=12.790156, "p_A1"=-0.0012500584}, {"timer"=10596.359, "p_A"=12.594844, "p_A1"=-0.0012500584}, {"timer"=10596.258, "p_A"=12.477656, "p_A1"=0.05734369}, {"timer"=10596.158, "p_A"=12.028438, "p_A1"=0.13546869}, {"timer"=10596.059, "p_A"=12.145625, "p_A1"=0.11593744}, {"timer"=10595.939, "p_A"=11.676875, "p_A1"=0.07687494}, {"timer"=10595.859, "p_A"=11.110469, "p_A1"=0.09640619}, {"timer"=10595.758, "p_A"=10.778438, "p_A1"=0.018281192}, {"timer"=10595.658, "p_A"=10.758906, "p_A1"=0.07687494}, {"timer"=10595.539, "p_A"=10.563594, "p_A1"=0.09640619}, {"timer"=10595.459, "p_A"=9.958125, "p_A1"=0.07687494}, {"timer"=10595.359, "p_A"=9.821406, "p_A1"=0.17453119}, {"timer"=10595.258, "p_A"=9.606563, "p_A1"=0.11593744}, {"timer"=10595.158, "p_A"=9.489375, "p_A1"=0.09640619}, {"timer"=10595.039, "p_A"=9.196406, "p_A1"=-0.0012500584}, {"timer"=10594.959, "p_A"=8.981563, "p_A1"=0.03781244}, {"timer"=10594.859, "p_A"=8.571406, "p_A1"=0.09640619}, {"timer"=10594.758, "p_A"=8.141719, "p_A1"=0.05734369}, {"timer"=10594.658, "p_A"=7.7510934, "p_A1"=0.03781244}, {"timer"=10594.559, "p_A"=7.497187, "p_A1"=0.09640619}, {"timer"=10594.459, "p_A"=7.633906, "p_A1"=0.17453119}, {"timer"=10594.359, "p_A"=7.0674996, "p_A1"=0.018281192}, {"timer"=10594.238, "p_A"=6.715937, "p_A1"=0.03781244}, {"timer"=10594.139, "p_A"=6.462031, "p_A1"=0.03781244}, {"timer"=10594.059, "p_A"=6.4424996, "p_A1"=-0.0012500584}, {"timer"=10593.939, "p_A"=6.012812, "p_A1"=0.05734369}, {"timer"=10593.838, "p_A"=5.622187, "p_A1"=-0.0012500584}, {"timer"=10593.758, "p_A"=5.368281, "p_A1"=0.07687494}, {"timer"=10593.658, "p_A"=5.231562, "p_A1"=0.03781244}, {"timer"=10593.539, "p_A"=4.8214064, "p_A1"=0.018281192}, {"timer"=10593.439, "p_A"=4.626094, "p_A1"=0.13546869}, {"timer"=10593.338, "p_A"=4.3526564, "p_A1"=-0.020781308}, {"timer"=10593.258, "p_A"=3.9815626, "p_A1"=0.07687494}, {"timer"=10593.158, "p_A"=3.7471876, "p_A1"=0.05734369}, {"timer"=10593.059, "p_A"=3.239375, "p_A1"=-0.04031256}, {"timer"=10592.939, "p_A"=3.1221876, "p_A1"=0.05734369}, {"timer"=10592.859, "p_A"=2.7510939, "p_A1"=-0.020781308}, {"timer"=10592.758, "p_A"=2.458125, "p_A1"=0.018281192}, {"timer"=10592.658, "p_A"=1.8526564, "p_A1"=0.13546869}, {"timer"=10592.539, "p_A"=1.6768751, "p_A1"=0.15499994}, {"timer"=10592.459, "p_A"=1.5206251, "p_A1"=0.07687494}, {"timer"=10592.359, "p_A"=1.3643751, "p_A1"=-0.0012500584}, {"timer"=10592.258, "p_A"=1.051875, "p_A1"=0.018281192}, {"timer"=10592.158, "p_A"=0.64171875, "p_A1"=-0.0012500584}, {"timer"=10592.059, "p_A"=0.87609375, "p_A1"=0.09640619}, {"timer"=10591.959, "p_A"=10.97375, "p_A1"=0.11593744}, {"timer"=10591.859, "p_A"=2.7901564, "p_A1"=0.018281192}, {"timer"=10591.758, "p_A"=4.079219, "p_A1"=-0.020781308}, {"timer"=10591.639, "p_A"=-0.06140625, "p_A1"=0.018281192}, {"timer"=10591.559, "p_A"=2.7315626, "p_A1"=0.018281192}, {"timer"=10591.439, "p_A"=8.044063, "p_A1"=0.07687494}, {"timer"=10591.338, "p_A"=6.774531, "p_A1"=-0.07937506}, {"timer"=10591.258, "p_A"=5.680781, "p_A1"=-0.05984381}, {"timer"=10591.158, "p_A"=5.055781, "p_A1"=-0.04031256}, {"timer"=10591.039, "p_A"=9.665156, "p_A1"=0.03781244}, {"timer"=10590.939, "p_A"=15.34875, "p_A1"=0.07687494}, {"timer"=10590.838, "p_A"=51.364372, "p_A1"=0.5260937}, {"timer"=10590.758, "p_A"=99.78234, "p_A1"=0.07687494}, {"timer"=10590.658, "p_A"=99.62609, "p_A1"=-0.0012500584}, {"timer"=10590.559, "p_A"=99.860466, "p_A1"=0.07687494}, {"timer"=10590.439, "p_A"=99.58703, "p_A1"=0.03781244}, {"timer"=10590.359, "p_A"=99.72375, "p_A1"=0.018281192}, {"timer"=10590.258, "p_A"=99.8214, "p_A1"=0.03781244}, {"timer"=10590.158, "p_A"=99.8214, "p_A1"=0.07687494}, {"timer"=10590.039, "p_A"=99.704216, "p_A1"=0.018281192}, {"timer"=10589.939, "p_A"=99.76281, "p_A1"=-0.04031256}, {"timer"=10589.838, "p_A"=99.547966, "p_A1"=0.018281192}, {"timer"=10589.738, "p_A"=99.95812, "p_A1"=0.05734369}, {"timer"=10589.658, "p_A"=99.80187, "p_A1"=0.05734369}, {"timer"=10589.539, "p_A"=99.78234, "p_A1"=0.03781244}, {"timer"=10589.459, "p_A"=99.64562, "p_A1"=0.05734369}, {"timer"=10589.359, "p_A"=99.58703, "p_A1"=0.018281192}, {"timer"=10589.238, "p_A"=99.89953, "p_A1"=-0.0012500584}, {"timer"=10589.158, "p_A"=99.66515, "p_A1"=0.03781244}, {"timer"=10589.059, "p_A"=99.66515, "p_A1"=0.09640619}, {"timer"=10588.959, "p_A"=99.45031, "p_A1"=-0.0012500584}, {"timer"=10588.859, "p_A"=99.97765, "p_A1"=0.07687494}, {"timer"=10588.758, "p_A"=99.89953, "p_A1"=0.15499994}, {"timer"=10588.658, "p_A"=99.62609, "p_A1"=0.07687494}, {"timer"=10588.559, "p_A"=99.58703, "p_A1"=0.03781244}, {"timer"=10588.439, "p_A"=99.8214, "p_A1"=0.07687494}, {"timer"=10588.359, "p_A"=99.66515, "p_A1"=0.03781244}, {"timer"=10588.258, "p_A"=99.88, "p_A1"=0.13546869}, {"timer"=10588.158, "p_A"=99.528435, "p_A1"=-0.04031256}, {"timer"=10588.039, "p_A"=99.62609, "p_A1"=-0.05984381}, {"timer"=10587.939, "p_A"=99.840935, "p_A1"=0.13546869}, {"timer"=10587.859, "p_A"=99.78234, "p_A1"=0.07687494}, {"timer"=10587.758, "p_A"=99.5089, "p_A1"=0.13546869}, {"timer"=10587.639, "p_A"=99.62609, "p_A1"=0.018281192}, {"timer"=10587.559, "p_A"=99.60656, "p_A1"=-0.020781308}, {"timer"=10587.459, "p_A"=99.31359, "p_A1"=0.05734369}, {"timer"=10587.338, "p_A"=99.528435, "p_A1"=-0.0012500584}, {"timer"=10587.238, "p_A"=99.17687, "p_A1"=0.05734369}, {"timer"=10587.158, "p_A"=99.5675, "p_A1"=0.19406244}, {"timer"=10587.059, "p_A"=99.35265, "p_A1"=-0.020781308}, {"timer"=10586.959, "p_A"=99.78234, "p_A1"=0.09640619}, {"timer"=10586.859, "p_A"=99.76281, "p_A1"=0.09640619}, {"timer"=10586.758, "p_A"=99.35265, "p_A1"=0.09640619}, {"timer"=10586.658, "p_A"=99.91906, "p_A1"=-0.020781308}, {"timer"=10586.559, "p_A"=99.684685, "p_A1"=0.05734369}, {"timer"=10586.459, "p_A"=99.74328, "p_A1"=0.09640619}, {"timer"=10586.359, "p_A"=99.60656, "p_A1"=0.11593744}, {"timer"=10586.258, "p_A"=99.8214, "p_A1"=-0.04031256}, {"timer"=10586.158, "p_A"=99.8214, "p_A1"=0.09640619}, {"timer"=10586.059, "p_A"=99.547966, "p_A1"=0.07687494}, {"timer"=10585.959, "p_A"=99.60656, "p_A1"=0.11593744}, {"timer"=10585.859, "p_A"=99.93859, "p_A1"=-0.020781308}, {"timer"=10585.758, "p_A"=99.684685, "p_A1"=0.05734369}, {"timer"=10585.658, "p_A"=99.547966, "p_A1"=0.09640619}, {"timer"=10585.559, "p_A"=99.89953, "p_A1"=-0.04031256}, {"timer"=10585.459, "p_A"=99.684685, "p_A1"=0.018281192}, {"timer"=10585.359, "p_A"=99.684685, "p_A1"=0.05734369}, {"timer"=10585.258, "p_A"=99.72375, "p_A1"=0.15499994}, {"timer"=10585.158, "p_A"=99.46984, "p_A1"=0.03781244}, {"timer"=10585.059, "p_A"=99.76281, "p_A1"=0.09640619}, {"timer"=10584.959, "p_A"=99.62609, "p_A1"=-0.05984381}, {"timer"=10584.838, "p_A"=99.60656, "p_A1"=0.07687494}, {"timer"=10584.758, "p_A"=99.547966, "p_A1"=0.07687494}, {"timer"=10584.658, "p_A"=99.58703, "p_A1"=0.17453119}, {"timer"=10584.559, "p_A"=99.684685, "p_A1"=0.05734369}, {"timer"=10584.459, "p_A"=99.60656, "p_A1"=0.07687494}, {"timer"=10584.359, "p_A"=99.704216, "p_A1"=-0.020781308}, {"timer"=10584.258, "p_A"=99.860466, "p_A1"=0.03781244}, {"timer"=10584.158, "p_A"=99.684685, "p_A1"=-0.05984381}, {"timer"=10584.059, "p_A"=99.704216, "p_A1"=0.05734369}, {"timer"=10583.959, "p_A"=99.8214, "p_A1"=0.11593744}, {"timer"=10583.859, "p_A"=99.66515, "p_A1"=0.13546869}, {"timer"=10583.758, "p_A"=99.64562, "p_A1"=0.018281192}, {"timer"=10583.658, "p_A"=99.74328, "p_A1"=0.05734369}, {"timer"=10583.559, "p_A"=99.95812, "p_A1"=0.13546869}, {"timer"=10583.459, "p_A"=99.528435, "p_A1"=0.018281192}, {"timer"=10583.359, "p_A"=99.64562, "p_A1"=0.018281192}, {"timer"=10583.258, "p_A"=99.60656, "p_A1"=-0.0012500584}, {"timer"=10583.158, "p_A"=99.72375, "p_A1"=0.05734369}, {"timer"=10583.059, "p_A"=99.74328, "p_A1"=-0.0012500584}, {"timer"=10582.959, "p_A"=99.33312, "p_A1"=0.05734369}, {"timer"=10582.859, "p_A"=99.58703, "p_A1"=0.05734369}, {"timer"=10582.758, "p_A"=99.41125, "p_A1"=0.018281192}, {"timer"=10582.658, "p_A"=99.60656, "p_A1"=0.05734369}, {"timer"=10582.559, "p_A"=99.48937, "p_A1"=0.07687494}, {"timer"=10582.459, "p_A"=99.78234, "p_A1"=0.07687494}, {"timer"=10582.359, "p_A"=99.45031, "p_A1"=-0.0012500584}, {"timer"=10582.258, "p_A"=99.5089, "p_A1"=0.05734369}, {"timer"=10582.158, "p_A"=99.62609, "p_A1"=-0.04031256}, {"timer"=10582.039, "p_A"=99.684685, "p_A1"=0.31124994}, {"timer"=10581.959, "p_A"=99.60656, "p_A1"=-0.020781308}, {"timer"=10581.838, "p_A"=99.35265, "p_A1"=0.07687494}, {"timer"=10581.738, "p_A"=99.58703, "p_A1"=0.05734369}, {"timer"=10581.658, "p_A"=99.64562, "p_A1"=0.11593744}, {"timer"=10581.559, "p_A"=99.58703, "p_A1"=0.05734369}, {"timer"=10581.459, "p_A"=99.64562, "p_A1"=0.018281192}, {"timer"=10581.359, "p_A"=99.46984, "p_A1"=0.03781244}, {"timer"=10581.238, "p_A"=99.547966, "p_A1"=0.05734369}, {"timer"=10581.158, "p_A"=99.64562, "p_A1"=0.05734369}, {"timer"=10581.059, "p_A"=99.46984, "p_A1"=-0.0012500584}, {"timer"=10580.959, "p_A"=99.41125, "p_A1"=-0.020781308}, {"timer"=10580.859, "p_A"=99.72375, "p_A1"=0.03781244}, {"timer"=10580.758, "p_A"=99.547966, "p_A1"=0.09640619}, {"timer"=10580.658, "p_A"=99.78234, "p_A1"=0.09640619}, {"timer"=10580.559, "p_A"=99.391716, "p_A1"=-0.0012500584}, {"timer"=10580.459, "p_A"=99.5675, "p_A1"=0.13546869}, {"timer"=10580.359, "p_A"=99.60656, "p_A1"=0.03781244}, {"timer"=10580.258, "p_A"=99.13781, "p_A1"=-0.0012500584}, {"timer"=10580.158, "p_A"=99.684685, "p_A1"=0.15499994}, {"timer"=10580.059, "p_A"=99.41125, "p_A1"=0.11593744}, {"timer"=10579.939, "p_A"=99.45031, "p_A1"=-0.020781308}, {"timer"=10579.838, "p_A"=99.547966, "p_A1"=0.018281192}, {"timer"=10579.758, "p_A"=99.58703, "p_A1"=0.11593744}, {"timer"=10579.658, "p_A"=99.48937, "p_A1"=0.13546869}, {"timer"=10579.559, "p_A"=99.58703, "p_A1"=-0.04031256}, {"timer"=10579.439, "p_A"=99.860466, "p_A1"=0.018281192}, {"timer"=10579.338, "p_A"=99.5089, "p_A1"=0.03781244}, {"timer"=10579.238, "p_A"=99.5675, "p_A1"=0.03781244}, {"timer"=10579.139, "p_A"=99.46984, "p_A1"=0.05734369}, {"timer"=10579.039, "p_A"=99.31359, "p_A1"=-0.0012500584}, {"timer"=10578.939, "p_A"=99.29406, "p_A1"=0.11593744}, {"timer"=10578.838, "p_A"=99.5675, "p_A1"=-0.0012500584}, {"timer"=10578.738, "p_A"=99.76281, "p_A1"=-0.0012500584}, {"timer"=10578.639, "p_A"=99.58703, "p_A1"=0.07687494}, {"timer"=10578.539, "p_A"=99.372185, "p_A1"=-0.020781308}, {"timer"=10578.439, "p_A"=99.547966, "p_A1"=0.15499994}, {"timer"=10578.338, "p_A"=99.35265, "p_A1"=0.11593744}, {"timer"=10578.238, "p_A"=99.33312, "p_A1"=-0.04031256}, {"timer"=10578.139, "p_A"=99.5675, "p_A1"=0.05734369}, {"timer"=10578.039, "p_A"=99.528435, "p_A1"=0.15499994}, {"timer"=10577.939, "p_A"=99.58703, "p_A1"=0.07687494}, {"timer"=10577.838, "p_A"=99.13781, "p_A1"=0.03781244}, {"timer"=10577.738, "p_A"=99.5675, "p_A1"=0.09640619}, {"timer"=10577.639, "p_A"=99.840935, "p_A1"=0.03781244}, {"timer"=10577.539, "p_A"=99.58703, "p_A1"=0.15499994}, {"timer"=10577.439, "p_A"=99.255, "p_A1"=0.05734369}, {"timer"=10577.338, "p_A"=99.372185, "p_A1"=0.09640619}, {"timer"=10577.238, "p_A"=99.62609, "p_A1"=0.13546869}, {"timer"=10577.139, "p_A"=99.46984, "p_A1"=0.05734369}, {"timer"=10577.039, "p_A"=99.5089, "p_A1"=0.17453119}, {"timer"=10576.939, "p_A"=99.33312, "p_A1"=0.03781244}, {"timer"=10576.838, "p_A"=99.46984, "p_A1"=0.03781244}, {"timer"=10576.738, "p_A"=99.35265, "p_A1"=0.09640619}, {"timer"=10576.639, "p_A"=99.5089, "p_A1"=0.018281192}, {"timer"=10576.539, "p_A"=99.58703, "p_A1"=0.13546869}, {"timer"=10576.439, "p_A"=99.27453, "p_A1"=-0.04031256}, {"timer"=10576.338, "p_A"=99.46984, "p_A1"=0.018281192}, {"timer"=10576.238, "p_A"=99.5089, "p_A1"=0.03781244}, {"timer"=10576.139, "p_A"=99.684685, "p_A1"=-0.04031256}, {"timer"=10576.039, "p_A"=99.41125, "p_A1"=0.018281192}, {"timer"=10575.939, "p_A"=99.35265, "p_A1"=0.09640619}, {"timer"=10575.838, "p_A"=99.72375, "p_A1"=0.07687494}, {"timer"=10575.738, "p_A"=99.528435, "p_A1"=0.03781244}, {"timer"=10575.639, "p_A"=99.391716, "p_A1"=0.13546869}, {"timer"=10575.539, "p_A"=99.43078, "p_A1"=0.11593744}, {"timer"=10575.439, "p_A"=99.43078, "p_A1"=0.09640619}, {"timer"=10575.338, "p_A"=99.391716, "p_A1"=0.05734369}, {"timer"=10575.238, "p_A"=99.45031, "p_A1"=0.03781244}, {"timer"=10575.139, "p_A"=99.60656, "p_A1"=0.07687494}, {"timer"=10575.039, "p_A"=99.58703, "p_A1"=0.03781244}, {"timer"=10574.939, "p_A"=99.64562, "p_A1"=0.11593744}, {"timer"=10574.838, "p_A"=99.46984, "p_A1"=-0.0012500584}, {"timer"=10574.738, "p_A"=99.72375, "p_A1"=0.07687494}, {"timer"=10574.639, "p_A"=99.5675, "p_A1"=-0.09890631}, {"timer"=10574.539, "p_A"=99.391716, "p_A1"=0.03781244}, {"timer"=10574.439, "p_A"=99.372185, "p_A1"=-0.020781308}, {"timer"=10574.338, "p_A"=99.64562, "p_A1"=0.23312494}, {"timer"=10574.238, "p_A"=99.528435, "p_A1"=0.13546869}, {"timer"=10574.139, "p_A"=99.46984, "p_A1"=0.07687494}, {"timer"=10574.039, "p_A"=99.46984, "p_A1"=0.07687494}, {"timer"=10573.939, "p_A"=99.43078, "p_A1"=0.018281192}, {"timer"=10573.838, "p_A"=99.45031, "p_A1"=0.09640619}, {"timer"=10573.738, "p_A"=99.5675, "p_A1"=0.13546869}, {"timer"=10573.639, "p_A"=99.33312, "p_A1"=-0.020781308}, {"timer"=10573.539, "p_A"=99.547966, "p_A1"=-0.020781308}, {"timer"=10573.439, "p_A"=99.46984, "p_A1"=0.03781244}, {"timer"=10573.338, "p_A"=99.41125, "p_A1"=0.018281192}, {"timer"=10573.238, "p_A"=99.43078, "p_A1"=0.03781244}, {"timer"=10573.139, "p_A"=99.62609, "p_A1"=0.09640619}, {"timer"=10573.039, "p_A"=99.528435, "p_A1"=-0.05984381}, {"timer"=10572.939, "p_A"=99.255, "p_A1"=-0.0012500584}, {"timer"=10572.838, "p_A"=99.079216, "p_A1"=0.05734369}, {"timer"=10572.738, "p_A"=99.391716, "p_A1"=-0.04031256}, {"timer"=10572.639, "p_A"=99.46984, "p_A1"=0.07687494}, {"timer"=10572.539, "p_A"=99.11828, "p_A1"=0.03781244}, {"timer"=10572.439, "p_A"=99.33312, "p_A1"=0.05734369}, {"timer"=10572.338, "p_A"=99.62609, "p_A1"=0.11593744}, {"timer"=10572.238, "p_A"=99.46984, "p_A1"=0.018281192}, {"timer"=10572.139, "p_A"=99.60656, "p_A1"=0.03781244}, {"timer"=10572.039, "p_A"=99.372185, "p_A1"=0.018281192}, {"timer"=10571.939, "p_A"=99.5675, "p_A1"=-0.020781308}, {"timer"=10571.838, "p_A"=99.27453, "p_A1"=0.09640619}, {"timer"=10571.738, "p_A"=99.41125, "p_A1"=-0.0012500584}, {"timer"=10571.639, "p_A"=99.31359, "p_A1"=0.03781244}, {"timer"=10571.539, "p_A"=99.528435, "p_A1"=0.05734369}, {"timer"=10571.439, "p_A"=99.1964, "p_A1"=0.03781244}, {"timer"=10571.338, "p_A"=99.13781, "p_A1"=0.15499994}, {"timer"=10571.238, "p_A"=99.41125, "p_A1"=0.11593744}, {"timer"=10571.139, "p_A"=99.29406, "p_A1"=0.07687494}, {"timer"=10571.039, "p_A"=99.48937, "p_A1"=-0.020781308}, {"timer"=10570.939, "p_A"=99.391716, "p_A1"=0.03781244}, {"timer"=10570.838, "p_A"=99.391716, "p_A1"=0.05734369}, {"timer"=10570.738, "p_A"=99.27453, "p_A1"=0.07687494}, {"timer"=10570.639, "p_A"=99.31359, "p_A1"=0.07687494}, {"timer"=10570.539, "p_A"=99.17687, "p_A1"=0.018281192}, {"timer"=10570.439, "p_A"=99.547966, "p_A1"=0.11593744}, {"timer"=10570.338, "p_A"=99.48937, "p_A1"=-0.05984381}, {"timer"=10570.238, "p_A"=99.58703, "p_A1"=0.07687494}, {"timer"=10570.139, "p_A"=99.29406, "p_A1"=0.03781244}, {"timer"=10570.039, "p_A"=99.35265, "p_A1"=0.09640619}, {"timer"=10569.939, "p_A"=99.45031, "p_A1"=0.09640619}, {"timer"=10569.838, "p_A"=99.45031, "p_A1"=0.05734369}, {"timer"=10569.738, "p_A"=99.17687, "p_A1"=0.018281192}, {"timer"=10569.639, "p_A"=99.391716, "p_A1"=0.018281192}, {"timer"=10569.539, "p_A"=99.29406, "p_A1"=0.018281192}, {"timer"=10569.439, "p_A"=99.33312, "p_A1"=-0.020781308}, {"timer"=10569.338, "p_A"=99.5675, "p_A1"=-0.04031256}, {"timer"=10569.238, "p_A"=99.46984, "p_A1"=-0.020781308}, {"timer"=10569.139, "p_A"=99.62609, "p_A1"=-0.020781308}, {"timer"=10569.039, "p_A"=99.33312, "p_A1"=-0.05984381}, {"timer"=10568.939, "p_A"=99.46984, "p_A1"=0.07687494}, {"timer"=10568.838, "p_A"=99.5675, "p_A1"=-0.020781308}, {"timer"=10568.738, "p_A"=99.528435, "p_A1"=-0.0012500584}, {"timer"=10568.639, "p_A"=99.35265, "p_A1"=0.03781244}, {"timer"=10568.539, "p_A"=99.235466, "p_A1"=0.03781244}, {"timer"=10568.439, "p_A"=99.255, "p_A1"=0.05734369}, {"timer"=10568.338, "p_A"=99.31359, "p_A1"=0.03781244}, {"timer"=10568.238, "p_A"=99.27453, "p_A1"=0.07687494}, {"timer"=10568.139, "p_A"=99.35265, "p_A1"=-0.0012500584}, {"timer"=10568.039, "p_A"=99.215935, "p_A1"=0.018281192}, {"timer"=10567.939, "p_A"=99.372185, "p_A1"=-0.04031256}, {"timer"=10567.838, "p_A"=99.58703, "p_A1"=-0.0012500584}, {"timer"=10567.738, "p_A"=99.11828, "p_A1"=-0.020781308}, {"timer"=10567.639, "p_A"=99.391716, "p_A1"=0.05734369}, {"timer"=10567.539, "p_A"=99.41125, "p_A1"=-0.020781308}, {"timer"=10567.439, "p_A"=99.29406, "p_A1"=0.03781244}, {"timer"=10567.338, "p_A"=99.255, "p_A1"=0.13546869}, {"timer"=10567.238, "p_A"=99.31359, "p_A1"=0.05734369}, {"timer"=10567.139, "p_A"=99.45031, "p_A1"=0.018281192}, {"timer"=10567.039, "p_A"=99.5089, "p_A1"=-0.020781308}, {"timer"=10566.939, "p_A"=99.46984, "p_A1"=0.11593744}, {"timer"=10566.838, "p_A"=99.079216, "p_A1"=0.03781244}, {"timer"=10566.738, "p_A"=99.235466, "p_A1"=0.07687494}, {"timer"=10566.639, "p_A"=99.31359, "p_A1"=0.05734369}, {"timer"=10566.539, "p_A"=99.5675, "p_A1"=0.05734369}, {"timer"=10566.439, "p_A"=99.43078, "p_A1"=-0.05984381}, {"timer"=10566.338, "p_A"=99.255, "p_A1"=0.018281192}, {"timer"=10566.238, "p_A"=99.46984, "p_A1"=-0.05984381}, {"timer"=10566.139, "p_A"=99.41125, "p_A1"=0.09640619}, {"timer"=10566.039, "p_A"=99.235466, "p_A1"=0.15499994}, {"timer"=10565.939, "p_A"=99.41125, "p_A1"=-0.020781308}, {"timer"=10565.838, "p_A"=99.1964, "p_A1"=0.05734369}, {"timer"=10565.738, "p_A"=99.391716, "p_A1"=0.13546869}, {"timer"=10565.639, "p_A"=99.29406, "p_A1"=-0.020781308}, {"timer"=10565.539, "p_A"=99.15734, "p_A1"=0.03781244}, {"timer"=10565.439, "p_A"=99.372185, "p_A1"=0.018281192}, {"timer"=10565.338, "p_A"=99.33312, "p_A1"=0.018281192}, {"timer"=10565.238, "p_A"=99.235466, "p_A1"=0.11593744}, {"timer"=10565.139, "p_A"=99.215935, "p_A1"=0.018281192}, {"timer"=10565.039, "p_A"=99.391716, "p_A1"=0.03781244}, {"timer"=10564.939, "p_A"=98.9425, "p_A1"=0.03781244}, {"timer"=10564.838, "p_A"=99.059685, "p_A1"=-0.0012500584}, {"timer"=10564.738, "p_A"=99.35265, "p_A1"=0.018281192}, {"timer"=10564.639, "p_A"=99.33312, "p_A1"=0.018281192}, {"timer"=10564.539, "p_A"=99.29406, "p_A1"=-0.020781308}, {"timer"=10564.439, "p_A"=99.547966, "p_A1"=0.07687494}, {"timer"=10564.338, "p_A"=99.391716, "p_A1"=-0.04031256}, {"timer"=10564.238, "p_A"=99.31359, "p_A1"=-0.020781308}, {"timer"=10564.139, "p_A"=99.27453, "p_A1"=0.018281192}, {"timer"=10564.039, "p_A"=99.27453, "p_A1"=-0.0012500584}, {"timer"=10563.939, "p_A"=99.215935, "p_A1"=0.03781244}, {"timer"=10563.838, "p_A"=99.255, "p_A1"=0.03781244}, {"timer"=10563.738, "p_A"=99.17687, "p_A1"=0.018281192}, {"timer"=10563.639, "p_A"=99.13781, "p_A1"=0.03781244}, {"timer"=10563.539, "p_A"=99.13781, "p_A1"=0.17453119}, {"timer"=10563.439, "p_A"=99.15734, "p_A1"=0.07687494}, {"timer"=10563.338, "p_A"=99.41125, "p_A1"=-0.020781308}, {"timer"=10563.238, "p_A"=99.391716, "p_A1"=0.17453119}, {"timer"=10563.139, "p_A"=99.1964, "p_A1"=0.05734369}, {"timer"=10563.039, "p_A"=99.079216, "p_A1"=-0.09890631}, {"timer"=10562.939, "p_A"=99.13781, "p_A1"=-0.020781308}, {"timer"=10562.838, "p_A"=99.15734, "p_A1"=0.018281192}, {"timer"=10562.738, "p_A"=99.35265, "p_A1"=0.09640619}, {"timer"=10562.639, "p_A"=99.15734, "p_A1"=0.15499994}, {"timer"=10562.539, "p_A"=99.17687, "p_A1"=0.05734369}, {"timer"=10562.439, "p_A"=99.1964, "p_A1"=0.03781244}, {"timer"=10562.338, "p_A"=99.27453, "p_A1"=0.15499994}, {"timer"=10562.238, "p_A"=99.48937, "p_A1"=0.018281192}, {"timer"=10562.139, "p_A"=99.41125, "p_A1"=0.05734369}, {"timer"=10562.039, "p_A"=99.17687, "p_A1"=0.018281192}, {"timer"=10561.939, "p_A"=99.255, "p_A1"=0.018281192}, {"timer"=10561.838, "p_A"=99.17687, "p_A1"=0.05734369}, {"timer"=10561.738, "p_A"=99.29406, "p_A1"=0.07687494}, {"timer"=10561.639, "p_A"=99.11828, "p_A1"=0.07687494}, {"timer"=10561.539, "p_A"=99.33312, "p_A1"=0.07687494}, {"timer"=10561.439, "p_A"=99.11828, "p_A1"=-0.09890631}, {"timer"=10561.338, "p_A"=99.15734, "p_A1"=0.018281192}, {"timer"=10561.238, "p_A"=99.00109, "p_A1"=0.11593744}, {"timer"=10561.139, "p_A"=99.215935, "p_A1"=0.05734369}, {"timer"=10561.039, "p_A"=99.11828, "p_A1"=0.05734369}, {"timer"=10560.939, "p_A"=99.255, "p_A1"=-0.020781308}, {"timer"=10560.838, "p_A"=99.17687, "p_A1"=0.11593744}, {"timer"=10560.738, "p_A"=99.11828, "p_A1"=-0.020781308}, {"timer"=10560.639, "p_A"=99.04015, "p_A1"=0.03781244}, {"timer"=10560.539, "p_A"=99.31359, "p_A1"=0.05734369}, {"timer"=10560.439, "p_A"=99.17687, "p_A1"=0.03781244}, {"timer"=10560.338, "p_A"=98.82531, "p_A1"=0.09640619}, {"timer"=10560.238, "p_A"=99.215935, "p_A1"=-0.020781308}, {"timer"=10560.139, "p_A"=99.079216, "p_A1"=0.018281192}, {"timer"=10560.039, "p_A"=99.17687, "p_A1"=0.03781244}, {"timer"=10559.939, "p_A"=99.02062, "p_A1"=-0.0012500584}, {"timer"=10559.838, "p_A"=99.059685, "p_A1"=-0.0012500584}, {"timer"=10559.738, "p_A"=99.17687, "p_A1"=0.11593744}, {"timer"=10559.639, "p_A"=99.09875, "p_A1"=0.05734369}, {"timer"=10559.539, "p_A"=99.15734, "p_A1"=0.03781244}, {"timer"=10559.439, "p_A"=99.1964, "p_A1"=0.018281192}, {"timer"=10559.338, "p_A"=99.15734, "p_A1"=-0.04031256}, {"timer"=10559.238, "p_A"=99.15734, "p_A1"=-0.04031256}, {"timer"=10559.139, "p_A"=99.079216, "p_A1"=0.03781244}, {"timer"=10559.039, "p_A"=99.15734, "p_A1"=0.03781244}, {"timer"=10558.939, "p_A"=99.29406, "p_A1"=0.13546869}, {"timer"=10558.838, "p_A"=98.86437, "p_A1"=0.05734369}, {"timer"=10558.738, "p_A"=99.09875, "p_A1"=0.11593744}, {"timer"=10558.619, "p_A"=98.96203, "p_A1"=0.11593744}, {"timer"=10558.539, "p_A"=99.15734, "p_A1"=-0.020781308}, {"timer"=10558.439, "p_A"=99.33312, "p_A1"=0.11593744}, {"timer"=10558.338, "p_A"=98.903435, "p_A1"=-0.0012500584}, {"timer"=10558.219, "p_A"=98.96203, "p_A1"=0.03781244}, {"timer"=10558.139, "p_A"=98.8839, "p_A1"=0.07687494}, {"timer"=10558.039, "p_A"=99.17687, "p_A1"=0.09640619}, {"timer"=10557.939, "p_A"=98.98156, "p_A1"=0.05734369}, {"timer"=10557.838, "p_A"=99.29406, "p_A1"=0.05734369}, {"timer"=10557.738, "p_A"=99.255, "p_A1"=0.018281192}, {"timer"=10557.639, "p_A"=99.13781, "p_A1"=0.05734369}, {"timer"=10557.539, "p_A"=99.35265, "p_A1"=0.19406244}, {"timer"=10557.439, "p_A"=98.8839, "p_A1"=0.03781244}, {"timer"=10557.338, "p_A"=98.98156, "p_A1"=0.018281192}, {"timer"=10557.238, "p_A"=98.96203, "p_A1"=0.09640619}, {"timer"=10557.139, "p_A"=99.255, "p_A1"=0.05734369}, {"timer"=10557.039, "p_A"=99.31359, "p_A1"=0.13546869}, {"timer"=10556.939, "p_A"=99.059685, "p_A1"=0.11593744}, {"timer"=10556.838, "p_A"=99.13781, "p_A1"=0.03781244}, {"timer"=10556.738, "p_A"=99.255, "p_A1"=0.07687494}, {"timer"=10556.639, "p_A"=99.09875, "p_A1"=0.018281192}, {"timer"=10556.539, "p_A"=99.059685, "p_A1"=0.11593744}, {"timer"=10556.439, "p_A"=99.33312, "p_A1"=0.07687494}, {"timer"=10556.338, "p_A"=99.079216, "p_A1"=-0.0012500584}, {"timer"=10556.219, "p_A"=99.15734, "p_A1"=0.03781244}, {"timer"=10556.139, "p_A"=98.82531, "p_A1"=0.03781244}, {"timer"=10556.039, "p_A"=98.82531, "p_A1"=0.07687494}, {"timer"=10555.939, "p_A"=99.35265, "p_A1"=0.07687494}, {"timer"=10555.838, "p_A"=98.9425, "p_A1"=0.05734369}, {"timer"=10555.738, "p_A"=99.09875, "p_A1"=-0.020781308}, {"timer"=10555.639, "p_A"=98.96203, "p_A1"=-0.04031256}, {"timer"=10555.539, "p_A"=99.09875, "p_A1"=0.018281192}, {"timer"=10555.439, "p_A"=99.079216, "p_A1"=0.03781244}, {"timer"=10555.338, "p_A"=99.00109, "p_A1"=-0.0012500584}, {"timer"=10555.238, "p_A"=99.079216, "p_A1"=0.03781244}, {"timer"=10555.139, "p_A"=98.9425, "p_A1"=0.13546869}, {"timer"=10555.039, "p_A"=99.11828, "p_A1"=-0.04031256}, {"timer"=10554.939, "p_A"=99.35265, "p_A1"=0.03781244}, {"timer"=10554.838, "p_A"=98.96203, "p_A1"=0.09640619}, {"timer"=10554.738, "p_A"=98.98156, "p_A1"=0.05734369}, {"timer"=10554.639, "p_A"=99.11828, "p_A1"=0.07687494}, {"timer"=10554.539, "p_A"=99.079216, "p_A1"=0.07687494}, {"timer"=10554.439, "p_A"=99.079216, "p_A1"=0.03781244}, {"timer"=10554.338, "p_A"=99.11828, "p_A1"=0.05734369}, {"timer"=10554.238, "p_A"=98.9425, "p_A1"=0.11593744}, {"timer"=10554.139, "p_A"=99.29406, "p_A1"=-0.0012500584}, {"timer"=10554.039, "p_A"=99.29406, "p_A1"=0.03781244}, {"timer"=10553.939, "p_A"=98.766716, "p_A1"=-0.0012500584}, {"timer"=10553.838, "p_A"=99.02062, "p_A1"=0.07687494}, {"timer"=10553.738, "p_A"=99.00109, "p_A1"=0.07687494}, {"timer"=10553.639, "p_A"=99.04015, "p_A1"=0.03781244}, {"timer"=10553.539, "p_A"=98.96203, "p_A1"=0.05734369}, {"timer"=10553.439, "p_A"=98.86437, "p_A1"=-0.020781308}, {"timer"=10553.338, "p_A"=99.04015, "p_A1"=0.07687494}, {"timer"=10553.238, "p_A"=99.059685, "p_A1"=0.17453119}, {"timer"=10553.139, "p_A"=98.80578, "p_A1"=0.05734369}, {"timer"=10553.039, "p_A"=99.15734, "p_A1"=-0.04031256}, {"timer"=10552.939, "p_A"=98.903435, "p_A1"=0.07687494}, {"timer"=10552.838, "p_A"=99.059685, "p_A1"=0.15499994}, {"timer"=10552.738, "p_A"=99.00109, "p_A1"=0.07687494}, {"timer"=10552.639, "p_A"=99.11828, "p_A1"=0.07687494}, {"timer"=10552.539, "p_A"=98.922966, "p_A1"=0.03781244}, {"timer"=10552.439, "p_A"=99.17687, "p_A1"=0.05734369}, {"timer"=10552.338, "p_A"=99.04015, "p_A1"=-0.0012500584}, {"timer"=10552.238, "p_A"=98.9425, "p_A1"=0.03781244}, {"timer"=10552.139, "p_A"=98.84484, "p_A1"=0.03781244}, {"timer"=10552.039, "p_A"=99.04015, "p_A1"=0.11593744}, {"timer"=10551.939, "p_A"=98.766716, "p_A1"=0.03781244}, {"timer"=10551.818, "p_A"=98.86437, "p_A1"=0.05734369}, {"timer"=10551.738, "p_A"=99.13781, "p_A1"=0.05734369}, {"timer"=10551.619, "p_A"=98.747185, "p_A1"=0.07687494}, {"timer"=10551.539, "p_A"=98.96203, "p_A1"=0.018281192}, {"timer"=10551.439, "p_A"=99.079216, "p_A1"=0.13546869}, {"timer"=10551.338, "p_A"=98.70812, "p_A1"=0.15499994}, {"timer"=10551.238, "p_A"=99.059685, "p_A1"=-0.05984381}, {"timer"=10551.139, "p_A"=98.8839, "p_A1"=0.05734369}, {"timer"=10551.039, "p_A"=98.922966, "p_A1"=0.11593744}, {"timer"=10550.939, "p_A"=99.09875, "p_A1"=0.03781244}, {"timer"=10550.838, "p_A"=98.68859, "p_A1"=0.09640619}, {"timer"=10550.738, "p_A"=99.00109, "p_A1"=0.11593744}, {"timer"=10550.639, "p_A"=98.747185, "p_A1"=0.018281192}, {"timer"=10550.539, "p_A"=98.86437, "p_A1"=0.05734369}, {"timer"=10550.439, "p_A"=98.98156, "p_A1"=0.17453119}, {"timer"=10550.338, "p_A"=99.02062, "p_A1"=0.21359369}, {"timer"=10550.238, "p_A"=98.922966, "p_A1"=0.09640619}, {"timer"=10550.139, "p_A"=98.9425, "p_A1"=0.05734369}, {"timer"=10550.039, "p_A"=98.98156, "p_A1"=-0.04031256}, {"timer"=10549.939, "p_A"=99.079216, "p_A1"=0.15499994}, {"timer"=10549.838, "p_A"=99.00109, "p_A1"=0.05734369}, {"timer"=10549.738, "p_A"=98.86437, "p_A1"=0.11593744}, {"timer"=10549.639, "p_A"=98.98156, "p_A1"=0.17453119}, {"timer"=10549.539, "p_A"=98.84484, "p_A1"=-0.020781308}, {"timer"=10549.439, "p_A"=98.86437, "p_A1"=0.03781244}, {"timer"=10549.338, "p_A"=99.02062, "p_A1"=0.07687494}, {"timer"=10549.238, "p_A"=99.04015, "p_A1"=0.03781244}, {"timer"=10549.139, "p_A"=98.8839, "p_A1"=0.018281192}, {"timer"=10549.039, "p_A"=99.11828, "p_A1"=-0.0012500584}, {"timer"=10548.939, "p_A"=98.9425, "p_A1"=0.05734369}, {"timer"=10548.838, "p_A"=98.82531, "p_A1"=0.03781244}, {"timer"=10548.738, "p_A"=99.079216, "p_A1"=0.018281192}, {"timer"=10548.639, "p_A"=99.09875, "p_A1"=0.05734369}, {"timer"=10548.539, "p_A"=98.86437, "p_A1"=-0.0012500584}, {"timer"=10548.439, "p_A"=98.96203, "p_A1"=0.03781244}, {"timer"=10548.338, "p_A"=98.64953, "p_A1"=0.05734369}, {"timer"=10548.238, "p_A"=98.84484, "p_A1"=-0.020781308}, {"timer"=10548.139, "p_A"=98.86437, "p_A1"=0.19406244}, {"timer"=10548.039, "p_A"=99.02062, "p_A1"=0.03781244}, {"timer"=10547.939, "p_A"=98.922966, "p_A1"=0.15499994}, {"timer"=10547.838, "p_A"=98.96203, "p_A1"=-0.05984381}, {"timer"=10547.738, "p_A"=98.64953, "p_A1"=0.05734369}, {"timer"=10547.639, "p_A"=98.922966, "p_A1"=0.07687494}, {"timer"=10547.539, "p_A"=98.84484, "p_A1"=-0.020781308}, {"timer"=10547.439, "p_A"=98.82531, "p_A1"=0.018281192}, {"timer"=10547.338, "p_A"=98.922966, "p_A1"=0.11593744}, {"timer"=10547.238, "p_A"=98.63, "p_A1"=0.07687494}, {"timer"=10547.139, "p_A"=98.86437, "p_A1"=0.05734369}, {"timer"=10547.039, "p_A"=98.78625, "p_A1"=0.03781244}, {"timer"=10546.939, "p_A"=98.70812, "p_A1"=0.05734369}, {"timer"=10546.838, "p_A"=98.64953, "p_A1"=0.03781244}, {"timer"=10546.738, "p_A"=98.55187, "p_A1"=0.05734369}, {"timer"=10546.639, "p_A"=99.059685, "p_A1"=-0.0012500584}, {"timer"=10546.539, "p_A"=98.766716, "p_A1"=-0.020781308}, {"timer"=10546.439, "p_A"=98.96203, "p_A1"=0.11593744}, {"timer"=10546.338, "p_A"=98.766716, "p_A1"=0.018281192}, {"timer"=10546.238, "p_A"=98.82531, "p_A1"=-0.020781308}, {"timer"=10546.139, "p_A"=98.766716, "p_A1"=0.11593744}, {"timer"=10546.039, "p_A"=98.64953, "p_A1"=0.018281192}, {"timer"=10545.939, "p_A"=98.766716, "p_A1"=0.19406244}, {"timer"=10545.838, "p_A"=98.84484, "p_A1"=0.018281192}, {"timer"=10545.738, "p_A"=98.80578, "p_A1"=-0.0012500584}, {"timer"=10545.639, "p_A"=98.9425, "p_A1"=0.09640619}, {"timer"=10545.539, "p_A"=98.55187, "p_A1"=-0.0012500584}, {"timer"=10545.439, "p_A"=98.64953, "p_A1"=0.018281192}, {"timer"=10545.338, "p_A"=98.80578, "p_A1"=-0.0012500584}, {"timer"=10545.238, "p_A"=98.78625, "p_A1"=-0.0012500584}, {"timer"=10545.139, "p_A"=98.9425, "p_A1"=-0.0012500584}, {"timer"=10545.039, "p_A"=98.84484, "p_A1"=0.018281192}, {"timer"=10544.939, "p_A"=98.66906, "p_A1"=0.03781244}, {"timer"=10544.838, "p_A"=98.78625, "p_A1"=0.03781244}, {"timer"=10544.738, "p_A"=98.747185, "p_A1"=0.03781244}, {"timer"=10544.639, "p_A"=98.63, "p_A1"=0.07687494}, {"timer"=10544.539, "p_A"=98.64953, "p_A1"=0.09640619}, {"timer"=10544.439, "p_A"=98.903435, "p_A1"=0.11593744}, {"timer"=10544.338, "p_A"=98.86437, "p_A1"=-0.04031256}, {"timer"=10544.238, "p_A"=98.64953, "p_A1"=-0.020781308}, {"timer"=10544.139, "p_A"=98.922966, "p_A1"=-0.020781308}, {"timer"=10544.039, "p_A"=98.86437, "p_A1"=0.05734369}, {"timer"=10543.939, "p_A"=98.63, "p_A1"=0.018281192}, {"timer"=10543.838, "p_A"=98.84484, "p_A1"=-0.05984381}, {"timer"=10543.738, "p_A"=98.66906, "p_A1"=0.07687494}, {"timer"=10543.639, "p_A"=98.903435, "p_A1"=-0.04031256}, {"timer"=10543.539, "p_A"=98.55187, "p_A1"=0.09640619}, {"timer"=10543.439, "p_A"=98.55187, "p_A1"=-0.0012500584}, {"timer"=10543.338, "p_A"=98.8839, "p_A1"=0.11593744}, {"timer"=10543.238, "p_A"=98.84484, "p_A1"=0.018281192}, {"timer"=10543.139, "p_A"=98.68859, "p_A1"=0.03781244}, {"timer"=10543.039, "p_A"=98.590935, "p_A1"=0.018281192}, {"timer"=10542.939, "p_A"=98.5714, "p_A1"=0.21359369}, {"timer"=10542.838, "p_A"=98.68859, "p_A1"=-0.0012500584}, {"timer"=10542.738, "p_A"=98.610466, "p_A1"=0.018281192}, {"timer"=10542.639, "p_A"=98.47375, "p_A1"=0.11593744}, {"timer"=10542.539, "p_A"=98.66906, "p_A1"=0.07687494}, {"timer"=10542.439, "p_A"=98.903435, "p_A1"=0.07687494}, {"timer"=10542.338, "p_A"=98.766716, "p_A1"=0.13546869}, {"timer"=10542.238, "p_A"=98.55187, "p_A1"=0.03781244}, {"timer"=10542.139, "p_A"=98.66906, "p_A1"=0.03781244}, {"timer"=10542.039, "p_A"=98.82531, "p_A1"=0.15499994}, {"timer"=10541.939, "p_A"=98.68859, "p_A1"=0.018281192}, {"timer"=10541.838, "p_A"=98.434685, "p_A1"=-0.04031256}, {"timer"=10541.738, "p_A"=98.80578, "p_A1"=0.018281192}, {"timer"=10541.639, "p_A"=98.434685, "p_A1"=-0.020781308}, {"timer"=10541.539, "p_A"=98.590935, "p_A1"=0.05734369}, {"timer"=10541.439, "p_A"=98.55187, "p_A1"=0.05734369}, {"timer"=10541.338, "p_A"=98.5714, "p_A1"=0.05734369}, {"timer"=10541.238, "p_A"=98.68859, "p_A1"=0.07687494}, {"timer"=10541.139, "p_A"=98.63, "p_A1"=-0.020781308}, {"timer"=10541.039, "p_A"=98.55187, "p_A1"=0.03781244}, {"timer"=10540.939, "p_A"=98.47375, "p_A1"=-0.020781308}, {"timer"=10540.838, "p_A"=98.66906, "p_A1"=0.11593744}, {"timer"=10540.738, "p_A"=98.63, "p_A1"=0.05734369}, {"timer"=10540.639, "p_A"=98.70812, "p_A1"=-0.020781308}, {"timer"=10540.539, "p_A"=98.55187, "p_A1"=0.11593744}, {"timer"=10540.439, "p_A"=98.33703, "p_A1"=-0.07937506}, {"timer"=10540.338, "p_A"=98.53234, "p_A1"=-0.0012500584}, {"timer"=10540.238, "p_A"=98.5714, "p_A1"=0.03781244}, {"timer"=10540.139, "p_A"=98.590935, "p_A1"=-0.020781308}, {"timer"=10540.039, "p_A"=98.747185, "p_A1"=-0.0012500584}]
  out "p_pump_p_return":cluster{"timer":sgl, "p_A":sgl, "p_A1":sgl}[](array[cluster])=[{"timer"=10600.039, "p_A"=0.99328125, "p_A1"=0.03625}, {"timer"=10599.939, "p_A"=27.165155, "p_A1"=0.03625}, {"timer"=10599.859, "p_A"=79.48937, "p_A1"=-0.022343751}, {"timer"=10599.758, "p_A"=127.55578, "p_A1"=0.114374995}, {"timer"=10599.658, "p_A"=147.4972, "p_A1"=0.05578125}, {"timer"=10599.559, "p_A"=151.91125, "p_A1"=0.114374995}, {"timer"=10599.439, "p_A"=152.55579, "p_A1"=0.075312495}, {"timer"=10599.338, "p_A"=152.36047, "p_A1"=0.03625}, {"timer"=10599.258, "p_A"=154.43079, "p_A1"=-0.002812501}, {"timer"=10599.158, "p_A"=154.82141, "p_A1"=-0.022343751}, {"timer"=10599.059, "p_A"=154.23547, "p_A1"=0.016718749}, {"timer"=10598.959, "p_A"=154.6847, "p_A1"=0.016718749}, {"timer"=10598.838, "p_A"=154.74329, "p_A1"=-0.100468755}, {"timer"=10598.738, "p_A"=154.02063, "p_A1"=-0.002812501}, {"timer"=10598.639, "p_A"=155.05579, "p_A1"=-0.041875}, {"timer"=10598.559, "p_A"=153.96204, "p_A1"=0.016718749}, {"timer"=10598.459, "p_A"=155.11438, "p_A1"=-0.022343751}, {"timer"=10598.359, "p_A"=154.33313, "p_A1"=-0.002812501}, {"timer"=10598.238, "p_A"=154.76282, "p_A1"=0.016718749}, {"timer"=10598.139, "p_A"=154.72375, "p_A1"=0.03625}, {"timer"=10598.059, "p_A"=154.0011, "p_A1"=0.114374995}, {"timer"=10597.959, "p_A"=154.9972, "p_A1"=0.114374995}, {"timer"=10597.859, "p_A"=154.11829, "p_A1"=-0.002812501}, {"timer"=10597.758, "p_A"=154.76282, "p_A1"=0.05578125}, {"timer"=10597.658, "p_A"=154.78235, "p_A1"=0.05578125}, {"timer"=10597.559, "p_A"=154.35266, "p_A1"=0.016718749}, {"timer"=10597.459, "p_A"=155.34875, "p_A1"=0.016718749}, {"timer"=10597.359, "p_A"=154.11829, "p_A1"=-0.002812501}, {"timer"=10597.238, "p_A"=154.97766, "p_A1"=-0.022343751}, {"timer"=10597.158, "p_A"=154.58704, "p_A1"=0.075312495}, {"timer"=10597.059, "p_A"=154.41125, "p_A1"=-0.080937505}, {"timer"=10596.959, "p_A"=155.07532, "p_A1"=0.016718749}, {"timer"=10596.859, "p_A"=154.15735, "p_A1"=0.03625}, {"timer"=10596.758, "p_A"=154.0011, "p_A1"=0.05578125}, {"timer"=10596.658, "p_A"=154.35266, "p_A1"=0.05578125}, {"timer"=10596.559, "p_A"=154.84094, "p_A1"=-0.002812501}, {"timer"=10596.459, "p_A"=154.86047, "p_A1"=0.03625}, {"timer"=10596.359, "p_A"=154.11829, "p_A1"=-0.002812501}, {"timer"=10596.258, "p_A"=155.13391, "p_A1"=0.016718749}, {"timer"=10596.158, "p_A"=154.11829, "p_A1"=0.016718749}, {"timer"=10596.059, "p_A"=155.09485, "p_A1"=0.016718749}, {"timer"=10595.939, "p_A"=154.66516, "p_A1"=0.03625}, {"timer"=10595.859, "p_A"=154.3136, "p_A1"=0.03625}, {"timer"=10595.758, "p_A"=155.1925, "p_A1"=0.016718749}, {"timer"=10595.658, "p_A"=154.0597, "p_A1"=-0.002812501}, {"timer"=10595.539, "p_A"=155.29016, "p_A1"=0.016718749}, {"timer"=10595.459, "p_A"=154.3136, "p_A1"=-0.041875}, {"timer"=10595.359, "p_A"=154.84094, "p_A1"=-0.041875}, {"timer"=10595.258, "p_A"=155.13391, "p_A1"=0.016718749}, {"timer"=10595.158, "p_A"=154.07922, "p_A1"=0.05578125}, {"timer"=10595.039, "p_A"=155.1925, "p_A1"=0.016718749}, {"timer"=10594.959, "p_A"=154.13782, "p_A1"=0.075312495}, {"timer"=10594.859, "p_A"=155.05579, "p_A1"=0.016718749}, {"timer"=10594.758, "p_A"=154.5675, "p_A1"=-0.120000005}, {"timer"=10594.658, "p_A"=154.19641, "p_A1"=0.114374995}, {"timer"=10594.559, "p_A"=155.3097, "p_A1"=0.114374995}, {"timer"=10594.459, "p_A"=154.04016, "p_A1"=0.075312495}, {"timer"=10594.359, "p_A"=155.29016, "p_A1"=0.114374995}, {"timer"=10594.238, "p_A"=154.21594, "p_A1"=0.114374995}, {"timer"=10594.139, "p_A"=154.86047, "p_A1"=0.016718749}, {"timer"=10594.059, "p_A"=154.88, "p_A1"=0.03625}, {"timer"=10593.939, "p_A"=154.21594, "p_A1"=0.05578125}, {"timer"=10593.838, "p_A"=155.15344, "p_A1"=-0.080937505}, {"timer"=10593.758, "p_A"=154.45032, "p_A1"=0.075312495}, {"timer"=10593.658, "p_A"=154.89954, "p_A1"=0.094843745}, {"timer"=10593.539, "p_A"=154.86047, "p_A1"=0.03625}, {"timer"=10593.439, "p_A"=154.19641, "p_A1"=-0.002812501}, {"timer"=10593.338, "p_A"=155.11438, "p_A1"=-0.022343751}, {"timer"=10593.258, "p_A"=154.0597, "p_A1"=0.016718749}, {"timer"=10593.158, "p_A"=155.13391, "p_A1"=-0.002812501}, {"timer"=10593.059, "p_A"=154.46985, "p_A1"=-0.002812501}, {"timer"=10592.939, "p_A"=154.29407, "p_A1"=0.03625}, {"timer"=10592.859, "p_A"=155.03625, "p_A1"=0.075312495}, {"timer"=10592.758, "p_A"=154.11829, "p_A1"=0.016718749}, {"timer"=10592.658, "p_A"=155.01672, "p_A1"=0.094843745}, {"timer"=10592.539, "p_A"=154.17688, "p_A1"=0.05578125}, {"timer"=10592.459, "p_A"=154.46985, "p_A1"=-0.022343751}, {"timer"=10592.359, "p_A"=155.2511, "p_A1"=0.016718749}, {"timer"=10592.258, "p_A"=154.66516, "p_A1"=0.075312495}, {"timer"=10592.158, "p_A"=154.23547, "p_A1"=0.03625}, {"timer"=10592.059, "p_A"=154.43079, "p_A1"=0.075312495}, {"timer"=10591.959, "p_A"=153.84485, "p_A1"=-0.041875}, {"timer"=10591.859, "p_A"=154.76282, "p_A1"=-0.002812501}, {"timer"=10591.758, "p_A"=154.82141, "p_A1"=0.016718749}, {"timer"=10591.639, "p_A"=154.23547, "p_A1"=0.05578125}, {"timer"=10591.559, "p_A"=153.86438, "p_A1"=0.03625}, {"timer"=10591.439, "p_A"=154.60657, "p_A1"=-0.002812501}, {"timer"=10591.338, "p_A"=154.27454, "p_A1"=0.03625}, {"timer"=10591.258, "p_A"=154.19641, "p_A1"=0.016718749}, {"timer"=10591.158, "p_A"=154.58704, "p_A1"=0.075312495}, {"timer"=10591.039, "p_A"=154.43079, "p_A1"=-0.041875}, {"timer"=10590.939, "p_A"=154.3722, "p_A1"=0.05578125}, {"timer"=10590.838, "p_A"=153.76672, "p_A1"=0.1925}, {"timer"=10590.758, "p_A"=154.88, "p_A1"=0.016718749}, {"timer"=10590.658, "p_A"=155.11438, "p_A1"=0.05578125}, {"timer"=10590.559, "p_A"=154.13782, "p_A1"=-0.002812501}, {"timer"=10590.439, "p_A"=155.32922, "p_A1"=0.094843745}, {"timer"=10590.359, "p_A"=153.98157, "p_A1"=0.05578125}, {"timer"=10590.258, "p_A"=154.84094, "p_A1"=0.03625}, {"timer"=10590.158, "p_A"=154.66516, "p_A1"=0.03625}, {"timer"=10590.039, "p_A"=154.48938, "p_A1"=0.03625}, {"timer"=10589.939, "p_A"=155.13391, "p_A1"=-0.002812501}, {"timer"=10589.838, "p_A"=154.21594, "p_A1"=0.075312495}, {"timer"=10589.738, "p_A"=155.1925, "p_A1"=0.03625}, {"timer"=10589.658, "p_A"=154.6847, "p_A1"=-0.022343751}, {"timer"=10589.539, "p_A"=154.70422, "p_A1"=0.075312495}, {"timer"=10589.459, "p_A"=155.13391, "p_A1"=0.094843745}, {"timer"=10589.359, "p_A"=154.04016, "p_A1"=0.114374995}, {"timer"=10589.238, "p_A"=155.13391, "p_A1"=-0.002812501}, {"timer"=10589.158, "p_A"=154.17688, "p_A1"=0.05578125}, {"timer"=10589.059, "p_A"=154.64563, "p_A1"=0.075312495}, {"timer"=10588.959, "p_A"=154.9972, "p_A1"=0.03625}, {"timer"=10588.859, "p_A"=154.3722, "p_A1"=0.05578125}, {"timer"=10588.758, "p_A"=155.23157, "p_A1"=0.05578125}, {"timer"=10588.658, "p_A"=153.9425, "p_A1"=0.016718749}, {"timer"=10588.559, "p_A"=154.88, "p_A1"=0.05578125}, {"timer"=10588.439, "p_A"=154.76282, "p_A1"=0.03625}, {"timer"=10588.359, "p_A"=154.04016, "p_A1"=0.016718749}, {"timer"=10588.258, "p_A"=155.34875, "p_A1"=-0.002812501}, {"timer"=10588.158, "p_A"=154.11829, "p_A1"=-0.041875}, {"timer"=10588.039, "p_A"=155.15344, "p_A1"=0.094843745}, {"timer"=10587.939, "p_A"=154.35266, "p_A1"=0.05578125}, {"timer"=10587.859, "p_A"=154.48938, "p_A1"=0.114374995}, {"timer"=10587.758, "p_A"=155.09485, "p_A1"=0.075312495}, {"timer"=10587.639, "p_A"=154.0597, "p_A1"=0.13390625}, {"timer"=10587.559, "p_A"=155.3097, "p_A1"=0.03625}, {"timer"=10587.459, "p_A"=154.27454, "p_A1"=0.05578125}, {"timer"=10587.338, "p_A"=154.70422, "p_A1"=0.016718749}, {"timer"=10587.238, "p_A"=155.17297, "p_A1"=0.016718749}, {"timer"=10587.158, "p_A"=154.19641, "p_A1"=0.21203125}, {"timer"=10587.059, "p_A"=155.2511, "p_A1"=0.016718749}, {"timer"=10586.959, "p_A"=154.11829, "p_A1"=0.075312495}, {"timer"=10586.859, "p_A"=154.88, "p_A1"=-0.041875}, {"timer"=10586.758, "p_A"=154.54797, "p_A1"=0.17296875}, {"timer"=10586.658, "p_A"=154.48938, "p_A1"=-0.041875}, {"timer"=10586.559, "p_A"=154.255, "p_A1"=0.05578125}, {"timer"=10586.459, "p_A"=154.11829, "p_A1"=0.114374995}, {"timer"=10586.359, "p_A"=155.17297, "p_A1"=0.05578125}, {"timer"=10586.258, "p_A"=154.52844, "p_A1"=0.05578125}, {"timer"=10586.158, "p_A"=154.74329, "p_A1"=0.05578125}, {"timer"=10586.059, "p_A"=155.01672, "p_A1"=0.114374995}, {"timer"=10585.959, "p_A"=153.9425, "p_A1"=0.03625}, {"timer"=10585.859, "p_A"=155.3097, "p_A1"=0.21203125}, {"timer"=10585.758, "p_A"=154.19641, "p_A1"=0.016718749}, {"timer"=10585.658, "p_A"=154.78235, "p_A1"=0.016718749}, {"timer"=10585.559, "p_A"=155.03625, "p_A1"=-0.06140625}, {"timer"=10585.459, "p_A"=154.41125, "p_A1"=0.094843745}, {"timer"=10585.359, "p_A"=155.29016, "p_A1"=0.05578125}, {"timer"=10585.258, "p_A"=154.09875, "p_A1"=0.075312495}, {"timer"=10585.158, "p_A"=155.07532, "p_A1"=-0.022343751}, {"timer"=10585.059, "p_A"=154.78235, "p_A1"=-0.06140625}, {"timer"=10584.959, "p_A"=154.82141, "p_A1"=0.114374995}, {"timer"=10584.838, "p_A"=155.23157, "p_A1"=0.114374995}, {"timer"=10584.758, "p_A"=153.96204, "p_A1"=-0.002812501}, {"timer"=10584.658, "p_A"=155.05579, "p_A1"=0.114374995}, {"timer"=10584.559, "p_A"=154.5675, "p_A1"=0.05578125}, {"timer"=10584.459, "p_A"=154.70422, "p_A1"=0.094843745}, {"timer"=10584.359, "p_A"=155.21204, "p_A1"=0.075312495}, {"timer"=10584.258, "p_A"=154.0597, "p_A1"=0.03625}, {"timer"=10584.158, "p_A"=155.40735, "p_A1"=-0.022343751}, {"timer"=10584.059, "p_A"=154.09875, "p_A1"=0.03625}, {"timer"=10583.959, "p_A"=154.74329, "p_A1"=0.1534375}, {"timer"=10583.859, "p_A"=154.66516, "p_A1"=0.13390625}, {"timer"=10583.758, "p_A"=154.23547, "p_A1"=-0.041875}, {"timer"=10583.658, "p_A"=154.97766, "p_A1"=0.094843745}, {"timer"=10583.559, "p_A"=154.29407, "p_A1"=0.05578125}, {"timer"=10583.459, "p_A"=155.05579, "p_A1"=0.05578125}, {"timer"=10583.359, "p_A"=154.58704, "p_A1"=0.075312495}, {"timer"=10583.258, "p_A"=154.27454, "p_A1"=0.05578125}, {"timer"=10583.158, "p_A"=155.15344, "p_A1"=0.05578125}, {"timer"=10583.059, "p_A"=154.0597, "p_A1"=0.075312495}, {"timer"=10582.959, "p_A"=155.13391, "p_A1"=0.03625}, {"timer"=10582.859, "p_A"=154.54797, "p_A1"=0.05578125}, {"timer"=10582.758, "p_A"=154.39172, "p_A1"=-0.041875}, {"timer"=10582.658, "p_A"=155.32922, "p_A1"=0.114374995}, {"timer"=10582.559, "p_A"=154.255, "p_A1"=-0.041875}, {"timer"=10582.459, "p_A"=155.2511, "p_A1"=0.05578125}, {"timer"=10582.359, "p_A"=154.9386, "p_A1"=0.016718749}, {"timer"=10582.258, "p_A"=154.54797, "p_A1"=0.03625}, {"timer"=10582.158, "p_A"=154.84094, "p_A1"=-0.100468755}, {"timer"=10582.039, "p_A"=154.17688, "p_A1"=0.075312495}, {"timer"=10581.959, "p_A"=155.38782, "p_A1"=0.094843745}, {"timer"=10581.838, "p_A"=154.07922, "p_A1"=0.075312495}, {"timer"=10581.738, "p_A"=155.01672, "p_A1"=0.016718749}, {"timer"=10581.658, "p_A"=154.74329, "p_A1"=0.075312495}, {"timer"=10581.559, "p_A"=154.13782, "p_A1"=-0.022343751}, {"timer"=10581.459, "p_A"=155.2511, "p_A1"=-0.022343751}, {"timer"=10581.359, "p_A"=154.0011, "p_A1"=-0.06140625}, {"timer"=10581.238, "p_A"=154.72375, "p_A1"=0.114374995}, {"timer"=10581.158, "p_A"=154.39172, "p_A1"=0.016718749}, {"timer"=10581.059, "p_A"=154.17688, "p_A1"=0.05578125}, {"timer"=10580.959, "p_A"=155.13391, "p_A1"=-0.022343751}, {"timer"=10580.859, "p_A"=154.0597, "p_A1"=0.016718749}, {"timer"=10580.758, "p_A"=154.86047, "p_A1"=-0.002812501}, {"timer"=10580.658, "p_A"=154.74329, "p_A1"=-0.002812501}, {"timer"=10580.559, "p_A"=154.3722, "p_A1"=0.016718749}, {"timer"=10580.459, "p_A"=155.17297, "p_A1"=-0.022343751}, {"timer"=10580.359, "p_A"=153.90344, "p_A1"=0.016718749}, {"timer"=10580.258, "p_A"=155.01672, "p_A1"=0.05578125}, {"timer"=10580.158, "p_A"=154.33313, "p_A1"=0.094843745}, {"timer"=10580.059, "p_A"=154.66516, "p_A1"=-0.002812501}, {"timer"=10579.939, "p_A"=154.9972, "p_A1"=0.05578125}, {"timer"=10579.838, "p_A"=154.13782, "p_A1"=0.016718749}, {"timer"=10579.758, "p_A"=155.21204, "p_A1"=0.05578125}, {"timer"=10579.658, "p_A"=154.29407, "p_A1"=0.016718749}, {"timer"=10579.559, "p_A"=154.6847, "p_A1"=-0.002812501}, {"timer"=10579.439, "p_A"=154.84094, "p_A1"=0.075312495}, {"timer"=10579.338, "p_A"=153.9425, "p_A1"=-0.002812501}, {"timer"=10579.238, "p_A"=155.32922, "p_A1"=0.03625}, {"timer"=10579.139, "p_A"=153.90344, "p_A1"=0.075312495}, {"timer"=10579.039, "p_A"=154.84094, "p_A1"=0.016718749}, {"timer"=10578.939, "p_A"=154.76282, "p_A1"=0.075312495}, {"timer"=10578.838, "p_A"=154.15735, "p_A1"=0.075312495}, {"timer"=10578.738, "p_A"=155.11438, "p_A1"=0.016718749}, {"timer"=10578.639, "p_A"=154.02063, "p_A1"=0.114374995}, {"timer"=10578.539, "p_A"=154.86047, "p_A1"=0.016718749}, {"timer"=10578.439, "p_A"=154.52844, "p_A1"=-0.022343751}, {"timer"=10578.338, "p_A"=154.11829, "p_A1"=-0.041875}, {"timer"=10578.238, "p_A"=155.23157, "p_A1"=0.03625}, {"timer"=10578.139, "p_A"=154.09875, "p_A1"=0.075312495}, {"timer"=10578.039, "p_A"=155.13391, "p_A1"=0.05578125}, {"timer"=10577.939, "p_A"=154.13782, "p_A1"=-0.041875}, {"timer"=10577.838, "p_A"=154.41125, "p_A1"=-0.002812501}, {"timer"=10577.738, "p_A"=155.03625, "p_A1"=0.13390625}, {"timer"=10577.639, "p_A"=154.09875, "p_A1"=0.03625}, {"timer"=10577.539, "p_A"=154.88, "p_A1"=0.075312495}, {"timer"=10577.439, "p_A"=154.29407, "p_A1"=0.016718749}, {"timer"=10577.338, "p_A"=154.52844, "p_A1"=0.094843745}, {"timer"=10577.238, "p_A"=155.05579, "p_A1"=0.016718749}, {"timer"=10577.139, "p_A"=153.98157, "p_A1"=0.03625}, {"timer"=10577.039, "p_A"=155.27063, "p_A1"=0.075312495}, {"timer"=10576.939, "p_A"=154.46985, "p_A1"=0.016718749}, {"timer"=10576.838, "p_A"=154.86047, "p_A1"=0.05578125}, {"timer"=10576.738, "p_A"=155.11438, "p_A1"=0.13390625}, {"timer"=10576.639, "p_A"=154.07922, "p_A1"=0.075312495}, {"timer"=10576.539, "p_A"=155.05579, "p_A1"=0.1925}, {"timer"=10576.439, "p_A"=154.255, "p_A1"=0.016718749}, {"timer"=10576.338, "p_A"=154.80188, "p_A1"=0.094843745}, {"timer"=10576.238, "p_A"=154.9972, "p_A1"=0.016718749}, {"timer"=10576.139, "p_A"=154.21594, "p_A1"=-0.022343751}, {"timer"=10576.039, "p_A"=155.34875, "p_A1"=0.016718749}, {"timer"=10575.939, "p_A"=154.07922, "p_A1"=0.03625}, {"timer"=10575.838, "p_A"=154.9972, "p_A1"=0.05578125}, {"timer"=10575.738, "p_A"=154.60657, "p_A1"=0.075312495}, {"timer"=10575.639, "p_A"=154.11829, "p_A1"=0.075312495}, {"timer"=10575.539, "p_A"=155.15344, "p_A1"=0.075312495}, {"timer"=10575.439, "p_A"=154.17688, "p_A1"=-0.002812501}, {"timer"=10575.338, "p_A"=155.03625, "p_A1"=-0.041875}, {"timer"=10575.238, "p_A"=154.82141, "p_A1"=0.094843745}, {"timer"=10575.139, "p_A"=154.41125, "p_A1"=-0.041875}, {"timer"=10575.039, "p_A"=154.91907, "p_A1"=0.114374995}, {"timer"=10574.939, "p_A"=154.07922, "p_A1"=0.114374995}, {"timer"=10574.838, "p_A"=155.01672, "p_A1"=0.05578125}, {"timer"=10574.738, "p_A"=154.78235, "p_A1"=0.016718749}, {"timer"=10574.639, "p_A"=154.07922, "p_A1"=-0.06140625}, {"timer"=10574.539, "p_A"=155.21204, "p_A1"=0.05578125}, {"timer"=10574.439, "p_A"=154.02063, "p_A1"=0.114374995}, {"timer"=10574.338, "p_A"=155.1925, "p_A1"=0.05578125}, {"timer"=10574.238, "p_A"=154.52844, "p_A1"=0.075312495}, {"timer"=10574.139, "p_A"=154.0597, "p_A1"=-0.002812501}, {"timer"=10574.039, "p_A"=154.97766, "p_A1"=0.075312495}, {"timer"=10573.939, "p_A"=153.86438, "p_A1"=0.03625}, {"timer"=10573.838, "p_A"=154.76282, "p_A1"=-0.041875}, {"timer"=10573.738, "p_A"=154.74329, "p_A1"=0.05578125}, {"timer"=10573.639, "p_A"=154.41125, "p_A1"=0.075312495}, {"timer"=10573.539, "p_A"=155.11438, "p_A1"=-0.002812501}, {"timer"=10573.439, "p_A"=154.0597, "p_A1"=0.03625}, {"timer"=10573.338, "p_A"=155.07532, "p_A1"=-0.041875}, {"timer"=10573.238, "p_A"=154.45032, "p_A1"=0.114374995}, {"timer"=10573.139, "p_A"=154.255, "p_A1"=0.114374995}, {"timer"=10573.039, "p_A"=155.09485, "p_A1"=0.075312495}, {"timer"=10572.939, "p_A"=154.11829, "p_A1"=0.094843745}, {"timer"=10572.838, "p_A"=155.17297, "p_A1"=0.114374995}, {"timer"=10572.738, "p_A"=154.50891, "p_A1"=0.05578125}, {"timer"=10572.639, "p_A"=154.58704, "p_A1"=0.114374995}, {"timer"=10572.539, "p_A"=155.05579, "p_A1"=-0.06140625}, {"timer"=10572.439, "p_A"=154.09875, "p_A1"=0.13390625}, {"timer"=10572.338, "p_A"=155.15344, "p_A1"=0.094843745}, {"timer"=10572.238, "p_A"=154.11829, "p_A1"=-0.002812501}, {"timer"=10572.139, "p_A"=154.46985, "p_A1"=0.03625}, {"timer"=10572.039, "p_A"=154.70422, "p_A1"=0.114374995}, {"timer"=10571.939, "p_A"=154.09875, "p_A1"=0.03625}, {"timer"=10571.838, "p_A"=155.40735, "p_A1"=0.17296875}, {"timer"=10571.738, "p_A"=154.23547, "p_A1"=-0.002812501}, {"timer"=10571.639, "p_A"=154.41125, "p_A1"=0.016718749}, {"timer"=10571.539, "p_A"=155.11438, "p_A1"=0.05578125}, {"timer"=10571.439, "p_A"=154.17688, "p_A1"=-0.002812501}, {"timer"=10571.338, "p_A"=155.27063, "p_A1"=-0.080937505}, {"timer"=10571.238, "p_A"=154.255, "p_A1"=0.094843745}, {"timer"=10571.139, "p_A"=154.52844, "p_A1"=-0.022343751}, {"timer"=10571.039, "p_A"=155.15344, "p_A1"=-0.041875}, {"timer"=10570.939, "p_A"=154.13782, "p_A1"=-0.041875}, {"timer"=10570.838, "p_A"=155.2511, "p_A1"=-0.06140625}, {"timer"=10570.738, "p_A"=154.19641, "p_A1"=0.03625}, {"timer"=10570.639, "p_A"=154.95813, "p_A1"=-0.022343751}, {"timer"=10570.539, "p_A"=154.82141, "p_A1"=0.03625}, {"timer"=10570.439, "p_A"=153.90344, "p_A1"=-0.041875}, {"timer"=10570.338, "p_A"=155.03625, "p_A1"=-0.022343751}, {"timer"=10570.238, "p_A"=153.9425, "p_A1"=-0.041875}, {"timer"=10570.139, "p_A"=154.95813, "p_A1"=0.075312495}, {"timer"=10570.039, "p_A"=154.82141, "p_A1"=0.075312495}, {"timer"=10569.939, "p_A"=153.98157, "p_A1"=0.016718749}, {"timer"=10569.838, "p_A"=155.32922, "p_A1"=0.03625}, {"timer"=10569.738, "p_A"=154.45032, "p_A1"=0.05578125}, {"timer"=10569.639, "p_A"=154.72375, "p_A1"=-0.022343751}, {"timer"=10569.539, "p_A"=154.74329, "p_A1"=0.016718749}, {"timer"=10569.439, "p_A"=154.3136, "p_A1"=0.05578125}, {"timer"=10569.338, "p_A"=154.88, "p_A1"=-0.041875}, {"timer"=10569.238, "p_A"=154.19641, "p_A1"=0.13390625}, {"timer"=10569.139, "p_A"=154.95813, "p_A1"=-0.002812501}, {"timer"=10569.039, "p_A"=155.05579, "p_A1"=0.03625}, {"timer"=10568.939, "p_A"=154.6261, "p_A1"=0.03625}, {"timer"=10568.838, "p_A"=155.2511, "p_A1"=0.05578125}, {"timer"=10568.738, "p_A"=153.96204, "p_A1"=-0.080937505}, {"timer"=10568.639, "p_A"=154.82141, "p_A1"=0.03625}, {"timer"=10568.539, "p_A"=154.46985, "p_A1"=-0.06140625}, {"timer"=10568.439, "p_A"=154.27454, "p_A1"=0.05578125}, {"timer"=10568.338, "p_A"=155.21204, "p_A1"=0.075312495}, {"timer"=10568.238, "p_A"=154.04016, "p_A1"=0.03625}, {"timer"=10568.139, "p_A"=154.95813, "p_A1"=0.094843745}, {"timer"=10568.039, "p_A"=154.78235, "p_A1"=0.05578125}, {"timer"=10567.939, "p_A"=154.29407, "p_A1"=0.016718749}, {"timer"=10567.838, "p_A"=155.23157, "p_A1"=0.03625}, {"timer"=10567.738, "p_A"=154.15735, "p_A1"=0.05578125}, {"timer"=10567.639, "p_A"=154.84094, "p_A1"=-0.002812501}, {"timer"=10567.539, "p_A"=154.86047, "p_A1"=-0.022343751}, {"timer"=10567.439, "p_A"=154.64563, "p_A1"=0.05578125}, {"timer"=10567.338, "p_A"=155.07532, "p_A1"=0.094843745}, {"timer"=10567.238, "p_A"=154.0597, "p_A1"=-0.002812501}, {"timer"=10567.139, "p_A"=155.01672, "p_A1"=0.075312495}, {"timer"=10567.039, "p_A"=154.76282, "p_A1"=0.016718749}, {"timer"=10566.939, "p_A"=154.27454, "p_A1"=-0.002812501}, {"timer"=10566.838, "p_A"=155.11438, "p_A1"=0.114374995}, {"timer"=10566.738, "p_A"=153.96204, "p_A1"=0.075312495}, {"timer"=10566.639, "p_A"=155.07532, "p_A1"=-0.002812501}, {"timer"=10566.539, "p_A"=154.3722, "p_A1"=-0.06140625}, {"timer"=10566.439, "p_A"=154.29407, "p_A1"=0.05578125}, {"timer"=10566.338, "p_A"=155.29016, "p_A1"=-0.002812501}, {"timer"=10566.238, "p_A"=154.27454, "p_A1"=0.075312495}, {"timer"=10566.139, "p_A"=155.17297, "p_A1"=0.03625}, {"timer"=10566.039, "p_A"=154.3722, "p_A1"=0.03625}, {"timer"=10565.939, "p_A"=154.21594, "p_A1"=-0.022343751}, {"timer"=10565.838, "p_A"=155.01672, "p_A1"=-0.041875}, {"timer"=10565.738, "p_A"=153.98157, "p_A1"=0.016718749}, {"timer"=10565.639, "p_A"=154.86047, "p_A1"=0.05578125}, {"timer"=10565.539, "p_A"=154.84094, "p_A1"=0.03625}, {"timer"=10565.439, "p_A"=154.23547, "p_A1"=0.114374995}, {"timer"=10565.338, "p_A"=155.15344, "p_A1"=0.13390625}, {"timer"=10565.238, "p_A"=154.07922, "p_A1"=0.05578125}, {"timer"=10565.139, "p_A"=155.11438, "p_A1"=0.03625}, {"timer"=10565.039, "p_A"=154.70422, "p_A1"=-0.022343751}, {"timer"=10564.939, "p_A"=154.41125, "p_A1"=0.03625}, {"timer"=10564.838, "p_A"=154.91907, "p_A1"=0.075312495}, {"timer"=10564.738, "p_A"=154.11829, "p_A1"=0.016718749}, {"timer"=10564.639, "p_A"=155.09485, "p_A1"=0.016718749}, {"timer"=10564.539, "p_A"=154.76282, "p_A1"=-0.041875}, {"timer"=10564.439, "p_A"=154.29407, "p_A1"=0.05578125}, {"timer"=10564.338, "p_A"=155.29016, "p_A1"=-0.002812501}, {"timer"=10564.238, "p_A"=154.27454, "p_A1"=0.016718749}, {"timer"=10564.139, "p_A"=155.07532, "p_A1"=-0.041875}, {"timer"=10564.039, "p_A"=154.70422, "p_A1"=0.05578125}, {"timer"=10563.939, "p_A"=154.27454, "p_A1"=-0.022343751}, {"timer"=10563.838, "p_A"=155.17297, "p_A1"=0.075312495}, {"timer"=10563.738, "p_A"=153.9425, "p_A1"=0.03625}, {"timer"=10563.639, "p_A"=155.3097, "p_A1"=0.114374995}, {"timer"=10563.539, "p_A"=154.74329, "p_A1"=0.03625}, {"timer"=10563.439, "p_A"=154.46985, "p_A1"=0.05578125}, {"timer"=10563.338, "p_A"=155.505, "p_A1"=-0.002812501}, {"timer"=10563.238, "p_A"=154.09875, "p_A1"=0.03625}, {"timer"=10563.139, "p_A"=155.09485, "p_A1"=-0.002812501}, {"timer"=10563.039, "p_A"=154.54797, "p_A1"=0.05578125}, {"timer"=10562.939, "p_A"=154.3136, "p_A1"=-0.002812501}, {"timer"=10562.838, "p_A"=154.9972, "p_A1"=-0.002812501}, {"timer"=10562.738, "p_A"=153.9425, "p_A1"=0.114374995}, {"timer"=10562.639, "p_A"=154.84094, "p_A1"=-0.022343751}, {"timer"=10562.539, "p_A"=154.60657, "p_A1"=0.016718749}, {"timer"=10562.439, "p_A"=154.33313, "p_A1"=0.016718749}, {"timer"=10562.338, "p_A"=155.05579, "p_A1"=0.05578125}, {"timer"=10562.238, "p_A"=154.21594, "p_A1"=0.016718749}, {"timer"=10562.139, "p_A"=154.80188, "p_A1"=-0.022343751}, {"timer"=10562.039, "p_A"=154.6847, "p_A1"=0.075312495}, {"timer"=10561.939, "p_A"=154.255, "p_A1"=0.094843745}, {"timer"=10561.838, "p_A"=155.11438, "p_A1"=-0.002812501}, {"timer"=10561.738, "p_A"=154.19641, "p_A1"=0.075312495}, {"timer"=10561.639, "p_A"=155.3097, "p_A1"=-0.06140625}, {"timer"=10561.539, "p_A"=154.58704, "p_A1"=-0.041875}, {"timer"=10561.439, "p_A"=154.52844, "p_A1"=0.016718749}, {"timer"=10561.338, "p_A"=154.84094, "p_A1"=0.075312495}, {"timer"=10561.238, "p_A"=154.0011, "p_A1"=0.1925}, {"timer"=10561.139, "p_A"=155.01672, "p_A1"=0.03625}, {"timer"=10561.039, "p_A"=154.70422, "p_A1"=0.075312495}, {"timer"=10560.939, "p_A"=154.17688, "p_A1"=0.114374995}, {"timer"=10560.838, "p_A"=155.09485, "p_A1"=0.075312495}, {"timer"=10560.738, "p_A"=154.09875, "p_A1"=0.03625}, {"timer"=10560.639, "p_A"=154.86047, "p_A1"=-0.002812501}, {"timer"=10560.539, "p_A"=154.66516, "p_A1"=0.075312495}, {"timer"=10560.439, "p_A"=154.255, "p_A1"=0.094843745}, {"timer"=10560.338, "p_A"=155.03625, "p_A1"=0.016718749}, {"timer"=10560.238, "p_A"=154.02063, "p_A1"=0.05578125}, {"timer"=10560.139, "p_A"=154.91907, "p_A1"=0.016718749}, {"timer"=10560.039, "p_A"=154.6847, "p_A1"=0.05578125}, {"timer"=10559.939, "p_A"=154.3722, "p_A1"=0.05578125}, {"timer"=10559.838, "p_A"=155.15344, "p_A1"=-0.002812501}, {"timer"=10559.738, "p_A"=153.92297, "p_A1"=-0.041875}, {"timer"=10559.639, "p_A"=154.88, "p_A1"=0.1534375}, {"timer"=10559.539, "p_A"=154.5675, "p_A1"=-0.002812501}, {"timer"=10559.439, "p_A"=154.3136, "p_A1"=0.016718749}, {"timer"=10559.338, "p_A"=155.07532, "p_A1"=0.03625}, {"timer"=10559.238, "p_A"=154.0597, "p_A1"=0.075312495}, {"timer"=10559.139, "p_A"=154.9972, "p_A1"=0.05578125}, {"timer"=10559.039, "p_A"=154.72375, "p_A1"=-0.041875}, {"timer"=10558.939, "p_A"=154.88, "p_A1"=0.075312495}, {"timer"=10558.838, "p_A"=155.505, "p_A1"=0.114374995}, {"timer"=10558.738, "p_A"=153.98157, "p_A1"=0.075312495}, {"timer"=10558.619, "p_A"=155.07532, "p_A1"=0.075312495}, {"timer"=10558.539, "p_A"=154.60657, "p_A1"=-0.002812501}, {"timer"=10558.439, "p_A"=154.50891, "p_A1"=0.016718749}, {"timer"=10558.338, "p_A"=155.13391, "p_A1"=0.03625}, {"timer"=10558.219, "p_A"=154.27454, "p_A1"=-0.041875}, {"timer"=10558.139, "p_A"=154.21594, "p_A1"=-0.002812501}, {"timer"=10558.039, "p_A"=154.76282, "p_A1"=0.05578125}, {"timer"=10557.939, "p_A"=154.3722, "p_A1"=-0.022343751}, {"timer"=10557.838, "p_A"=154.97766, "p_A1"=0.094843745}, {"timer"=10557.738, "p_A"=153.84485, "p_A1"=-0.041875}, {"timer"=10557.639, "p_A"=155.05579, "p_A1"=-0.002812501}, {"timer"=10557.539, "p_A"=154.46985, "p_A1"=0.05578125}, {"timer"=10557.439, "p_A"=154.35266, "p_A1"=0.094843745}, {"timer"=10557.338, "p_A"=155.09485, "p_A1"=0.05578125}, {"timer"=10557.238, "p_A"=154.0597, "p_A1"=0.03625}, {"timer"=10557.139, "p_A"=155.1925, "p_A1"=0.114374995}, {"timer"=10557.039, "p_A"=154.33313, "p_A1"=0.1534375}, {"timer"=10556.939, "p_A"=154.52844, "p_A1"=0.03625}, {"timer"=10556.838, "p_A"=154.9972, "p_A1"=0.114374995}, {"timer"=10556.738, "p_A"=154.07922, "p_A1"=0.114374995}, {"timer"=10556.639, "p_A"=155.07532, "p_A1"=0.05578125}, {"timer"=10556.539, "p_A"=154.11829, "p_A1"=0.03625}, {"timer"=10556.439, "p_A"=154.3722, "p_A1"=0.13390625}, {"timer"=10556.338, "p_A"=155.03625, "p_A1"=-0.002812501}, {"timer"=10556.219, "p_A"=153.82532, "p_A1"=0.03625}, {"timer"=10556.139, "p_A"=154.07922, "p_A1"=-0.06140625}, {"timer"=10556.039, "p_A"=154.33313, "p_A1"=-0.022343751}, {"timer"=10555.939, "p_A"=154.86047, "p_A1"=0.016718749}, {"timer"=10555.838, "p_A"=154.9972, "p_A1"=0.094843745}, {"timer"=10555.738, "p_A"=154.09875, "p_A1"=0.13390625}, {"timer"=10555.639, "p_A"=154.91907, "p_A1"=-0.022343751}, {"timer"=10555.539, "p_A"=154.3136, "p_A1"=0.075312495}, {"timer"=10555.439, "p_A"=154.35266, "p_A1"=-0.002812501}, {"timer"=10555.338, "p_A"=154.9972, "p_A1"=-0.002812501}, {"timer"=10555.238, "p_A"=154.0011, "p_A1"=0.05578125}, {"timer"=10555.139, "p_A"=155.09485, "p_A1"=0.03625}, {"timer"=10555.039, "p_A"=154.3136, "p_A1"=0.075312495}, {"timer"=10554.939, "p_A"=154.45032, "p_A1"=0.05578125}, {"timer"=10554.838, "p_A"=154.86047, "p_A1"=0.114374995}, {"timer"=10554.738, "p_A"=154.0011, "p_A1"=-0.002812501}, {"timer"=10554.639, "p_A"=155.07532, "p_A1"=0.094843745}, {"timer"=10554.539, "p_A"=154.39172, "p_A1"=0.016718749}, {"timer"=10554.439, "p_A"=154.64563, "p_A1"=0.016718749}, {"timer"=10554.338, "p_A"=155.03625, "p_A1"=0.114374995}, {"timer"=10554.238, "p_A"=153.90344, "p_A1"=0.016718749}, {"timer"=10554.139, "p_A"=154.9386, "p_A1"=-0.041875}, {"timer"=10554.039, "p_A"=154.0011, "p_A1"=0.03625}, {"timer"=10553.939, "p_A"=154.29407, "p_A1"=-0.002812501}, {"timer"=10553.838, "p_A"=154.66516, "p_A1"=0.13390625}, {"timer"=10553.738, "p_A"=153.90344, "p_A1"=0.114374995}, {"timer"=10553.639, "p_A"=155.15344, "p_A1"=-0.041875}, {"timer"=10553.539, "p_A"=154.6847, "p_A1"=0.094843745}, {"timer"=10553.439, "p_A"=154.82141, "p_A1"=0.03625}, {"timer"=10553.338, "p_A"=155.21204, "p_A1"=0.13390625}, {"timer"=10553.238, "p_A"=154.3136, "p_A1"=0.075312495}, {"timer"=10553.139, "p_A"=155.38782, "p_A1"=0.016718749}, {"timer"=10553.039, "p_A"=154.41125, "p_A1"=-0.080937505}, {"timer"=10552.939, "p_A"=154.6847, "p_A1"=-0.022343751}, {"timer"=10552.838, "p_A"=155.2511, "p_A1"=-0.002812501}, {"timer"=10552.738, "p_A"=154.39172, "p_A1"=-0.002812501}, {"timer"=10552.639, "p_A"=155.29016, "p_A1"=0.114374995}, {"timer"=10552.539, "p_A"=154.76282, "p_A1"=-0.002812501}, {"timer"=10552.439, "p_A"=155.13391, "p_A1"=0.075312495}, {"timer"=10552.338, "p_A"=154.5675, "p_A1"=-0.022343751}, {"timer"=10552.238, "p_A"=154.07922, "p_A1"=0.075312495}, {"timer"=10552.139, "p_A"=155.34875, "p_A1"=-0.041875}, {"timer"=10552.039, "p_A"=154.74329, "p_A1"=-0.041875}, {"timer"=10551.939, "p_A"=154.97766, "p_A1"=0.05578125}, {"timer"=10551.818, "p_A"=155.21204, "p_A1"=0.03625}, {"timer"=10551.738, "p_A"=155.5636, "p_A1"=-0.041875}, {"timer"=10551.619, "p_A"=155.27063, "p_A1"=0.075312495}, {"timer"=10551.539, "p_A"=154.9972, "p_A1"=0.05578125}, {"timer"=10551.439, "p_A"=154.76282, "p_A1"=0.05578125}, {"timer"=10551.338, "p_A"=155.2511, "p_A1"=-0.002812501}, {"timer"=10551.238, "p_A"=154.15735, "p_A1"=0.05578125}, {"timer"=10551.139, "p_A"=154.5675, "p_A1"=0.094843745}, {"timer"=10551.039, "p_A"=154.88, "p_A1"=-0.002812501}, {"timer"=10550.939, "p_A"=154.64563, "p_A1"=0.03625}, {"timer"=10550.838, "p_A"=155.34875, "p_A1"=0.03625}, {"timer"=10550.738, "p_A"=154.33313, "p_A1"=0.05578125}, {"timer"=10550.639, "p_A"=155.36829, "p_A1"=0.05578125}, {"timer"=10550.539, "p_A"=154.95813, "p_A1"=0.1534375}, {"timer"=10550.439, "p_A"=154.66516, "p_A1"=-0.002812501}, {"timer"=10550.338, "p_A"=155.11438, "p_A1"=0.075312495}, {"timer"=10550.238, "p_A"=154.29407, "p_A1"=-0.022343751}, {"timer"=10550.139, "p_A"=155.23157, "p_A1"=0.075312495}, {"timer"=10550.039, "p_A"=154.89954, "p_A1"=-0.06140625}, {"timer"=10549.939, "p_A"=154.27454, "p_A1"=0.114374995}, {"timer"=10549.838, "p_A"=155.3097, "p_A1"=-0.022343751}, {"timer"=10549.738, "p_A"=154.19641, "p_A1"=0.016718749}, {"timer"=10549.639, "p_A"=155.15344, "p_A1"=-0.120000005}, {"timer"=10549.539, "p_A"=154.64563, "p_A1"=0.03625}, {"timer"=10549.439, "p_A"=154.255, "p_A1"=0.1925}, {"timer"=10549.338, "p_A"=154.50891, "p_A1"=0.016718749}, {"timer"=10549.238, "p_A"=154.48938, "p_A1"=0.05578125}, {"timer"=10549.139, "p_A"=155.07532, "p_A1"=0.05578125}, {"timer"=10549.039, "p_A"=155.32922, "p_A1"=0.016718749}, {"timer"=10548.939, "p_A"=154.3722, "p_A1"=0.094843745}, {"timer"=10548.838, "p_A"=155.27063, "p_A1"=0.03625}, {"timer"=10548.738, "p_A"=154.5675, "p_A1"=0.016718749}, {"timer"=10548.639, "p_A"=154.64563, "p_A1"=-0.022343751}, {"timer"=10548.539, "p_A"=155.27063, "p_A1"=0.03625}, {"timer"=10548.439, "p_A"=154.15735, "p_A1"=-0.041875}, {"timer"=10548.338, "p_A"=155.34875, "p_A1"=-0.002812501}, {"timer"=10548.238, "p_A"=154.60657, "p_A1"=-0.022343751}, {"timer"=10548.139, "p_A"=154.54797, "p_A1"=0.03625}, {"timer"=10548.039, "p_A"=155.36829, "p_A1"=0.016718749}, {"timer"=10547.939, "p_A"=154.45032, "p_A1"=0.094843745}, {"timer"=10547.838, "p_A"=155.05579, "p_A1"=-0.002812501}, {"timer"=10547.738, "p_A"=154.74329, "p_A1"=-0.002812501}, {"timer"=10547.639, "p_A"=154.15735, "p_A1"=0.114374995}, {"timer"=10547.539, "p_A"=155.2511, "p_A1"=0.016718749}, {"timer"=10547.439, "p_A"=154.27454, "p_A1"=-0.002812501}, {"timer"=10547.338, "p_A"=154.9386, "p_A1"=0.13390625}, {"timer"=10547.238, "p_A"=155.29016, "p_A1"=0.075312495}, {"timer"=10547.139, "p_A"=154.29407, "p_A1"=0.075312495}, {"timer"=10547.039, "p_A"=155.38782, "p_A1"=0.075312495}, {"timer"=10546.939, "p_A"=154.74329, "p_A1"=0.016718749}, {"timer"=10546.838, "p_A"=154.5675, "p_A1"=0.016718749}, {"timer"=10546.738, "p_A"=155.11438, "p_A1"=0.016718749}, {"timer"=10546.639, "p_A"=154.13782, "p_A1"=0.03625}, {"timer"=10546.539, "p_A"=155.13391, "p_A1"=0.075312495}, {"timer"=10546.439, "p_A"=154.97766, "p_A1"=0.075312495}, {"timer"=10546.338, "p_A"=154.50891, "p_A1"=0.016718749}, {"timer"=10546.238, "p_A"=155.40735, "p_A1"=0.016718749}, {"timer"=10546.139, "p_A"=154.50891, "p_A1"=0.075312495}, {"timer"=10546.039, "p_A"=155.15344, "p_A1"=-0.002812501}, {"timer"=10545.939, "p_A"=155.09485, "p_A1"=0.016718749}, {"timer"=10545.838, "p_A"=154.255, "p_A1"=0.094843745}, {"timer"=10545.738, "p_A"=155.11438, "p_A1"=0.05578125}, {"timer"=10545.639, "p_A"=154.5675, "p_A1"=0.016718749}, {"timer"=10545.539, "p_A"=154.9386, "p_A1"=-0.06140625}, {"timer"=10545.439, "p_A"=155.34875, "p_A1"=0.114374995}, {"timer"=10545.338, "p_A"=154.29407, "p_A1"=0.05578125}, {"timer"=10545.238, "p_A"=155.13391, "p_A1"=-0.002812501}, {"timer"=10545.139, "p_A"=154.84094, "p_A1"=0.03625}, {"timer"=10545.039, "p_A"=154.45032, "p_A1"=0.016718749}, {"timer"=10544.939, "p_A"=155.34875, "p_A1"=0.094843745}, {"timer"=10544.838, "p_A"=154.29407, "p_A1"=0.03625}, {"timer"=10544.738, "p_A"=155.05579, "p_A1"=-0.022343751}, {"timer"=10544.639, "p_A"=154.95813, "p_A1"=0.03625}, {"timer"=10544.539, "p_A"=154.45032, "p_A1"=-0.022343751}, {"timer"=10544.439, "p_A"=155.68079, "p_A1"=0.075312495}, {"timer"=10544.338, "p_A"=154.19641, "p_A1"=-0.002812501}, {"timer"=10544.238, "p_A"=154.91907, "p_A1"=-0.022343751}, {"timer"=10544.139, "p_A"=155.15344, "p_A1"=-0.100468755}, {"timer"=10544.039, "p_A"=154.255, "p_A1"=-0.002812501}, {"timer"=10543.939, "p_A"=155.1925, "p_A1"=0.05578125}, {"timer"=10543.838, "p_A"=154.5675, "p_A1"=0.075312495}, {"timer"=10543.738, "p_A"=154.6847, "p_A1"=0.075312495}, {"timer"=10543.639, "p_A"=155.505, "p_A1"=0.05578125}, {"timer"=10543.539, "p_A"=154.39172, "p_A1"=0.016718749}, {"timer"=10543.439, "p_A"=155.11438, "p_A1"=0.05578125}, {"timer"=10543.338, "p_A"=154.9972, "p_A1"=0.016718749}, {"timer"=10543.238, "p_A"=154.15735, "p_A1"=-0.100468755}, {"timer"=10543.139, "p_A"=155.3097, "p_A1"=0.075312495}, {"timer"=10543.039, "p_A"=154.52844, "p_A1"=0.05578125}, {"timer"=10542.939, "p_A"=154.9972, "p_A1"=0.03625}, {"timer"=10542.838, "p_A"=155.40735, "p_A1"=0.05578125}, {"timer"=10542.738, "p_A"=154.41125, "p_A1"=0.016718749}, {"timer"=10542.639, "p_A"=155.60266, "p_A1"=0.016718749}, {"timer"=10542.539, "p_A"=154.80188, "p_A1"=-0.002812501}, {"timer"=10542.439, "p_A"=154.60657, "p_A1"=0.03625}, {"timer"=10542.338, "p_A"=155.32922, "p_A1"=0.075312495}, {"timer"=10542.238, "p_A"=154.21594, "p_A1"=-0.002812501}, {"timer"=10542.139, "p_A"=154.78235, "p_A1"=0.03625}, {"timer"=10542.039, "p_A"=154.89954, "p_A1"=0.03625}, {"timer"=10541.939, "p_A"=154.64563, "p_A1"=0.075312495}, {"timer"=10541.838, "p_A"=155.40735, "p_A1"=0.094843745}, {"timer"=10541.738, "p_A"=154.46985, "p_A1"=0.03625}, {"timer"=10541.639, "p_A"=155.05579, "p_A1"=0.016718749}, {"timer"=10541.539, "p_A"=155.1925, "p_A1"=0.05578125}, {"timer"=10541.439, "p_A"=154.3136, "p_A1"=0.114374995}, {"timer"=10541.338, "p_A"=155.21204, "p_A1"=0.05578125}, {"timer"=10541.238, "p_A"=154.48938, "p_A1"=0.13390625}, {"timer"=10541.139, "p_A"=154.64563, "p_A1"=-0.022343751}, {"timer"=10541.039, "p_A"=155.15344, "p_A1"=0.016718749}, {"timer"=10540.939, "p_A"=154.46985, "p_A1"=0.075312495}, {"timer"=10540.838, "p_A"=155.36829, "p_A1"=0.075312495}, {"timer"=10540.738, "p_A"=154.66516, "p_A1"=-0.002812501}, {"timer"=10540.639, "p_A"=154.66516, "p_A1"=-0.002812501}, {"timer"=10540.539, "p_A"=155.46594, "p_A1"=0.094843745}, {"timer"=10540.439, "p_A"=154.29407, "p_A1"=0.05578125}, {"timer"=10540.338, "p_A"=155.13391, "p_A1"=0.016718749}, {"timer"=10540.238, "p_A"=154.80188, "p_A1"=-0.06140625}, {"timer"=10540.139, "p_A"=154.29407, "p_A1"=-0.002812501}, {"timer"=10540.039, "p_A"=155.42688, "p_A1"=0.075312495}]
  in  "reset_plots":bool
  in  "plot_limiter_(sec)":i32=60
  in  "Limit plot size?":bool=TRUE
  out "time_at_plot_start":dbl=14729.029296875
  out "plot_timer":dbl=10600.119140625
  out "timer":dbl=25329.1484375
  # "LOG CONTROL"
  # "LOG"
  # "PLOT CONTROL"
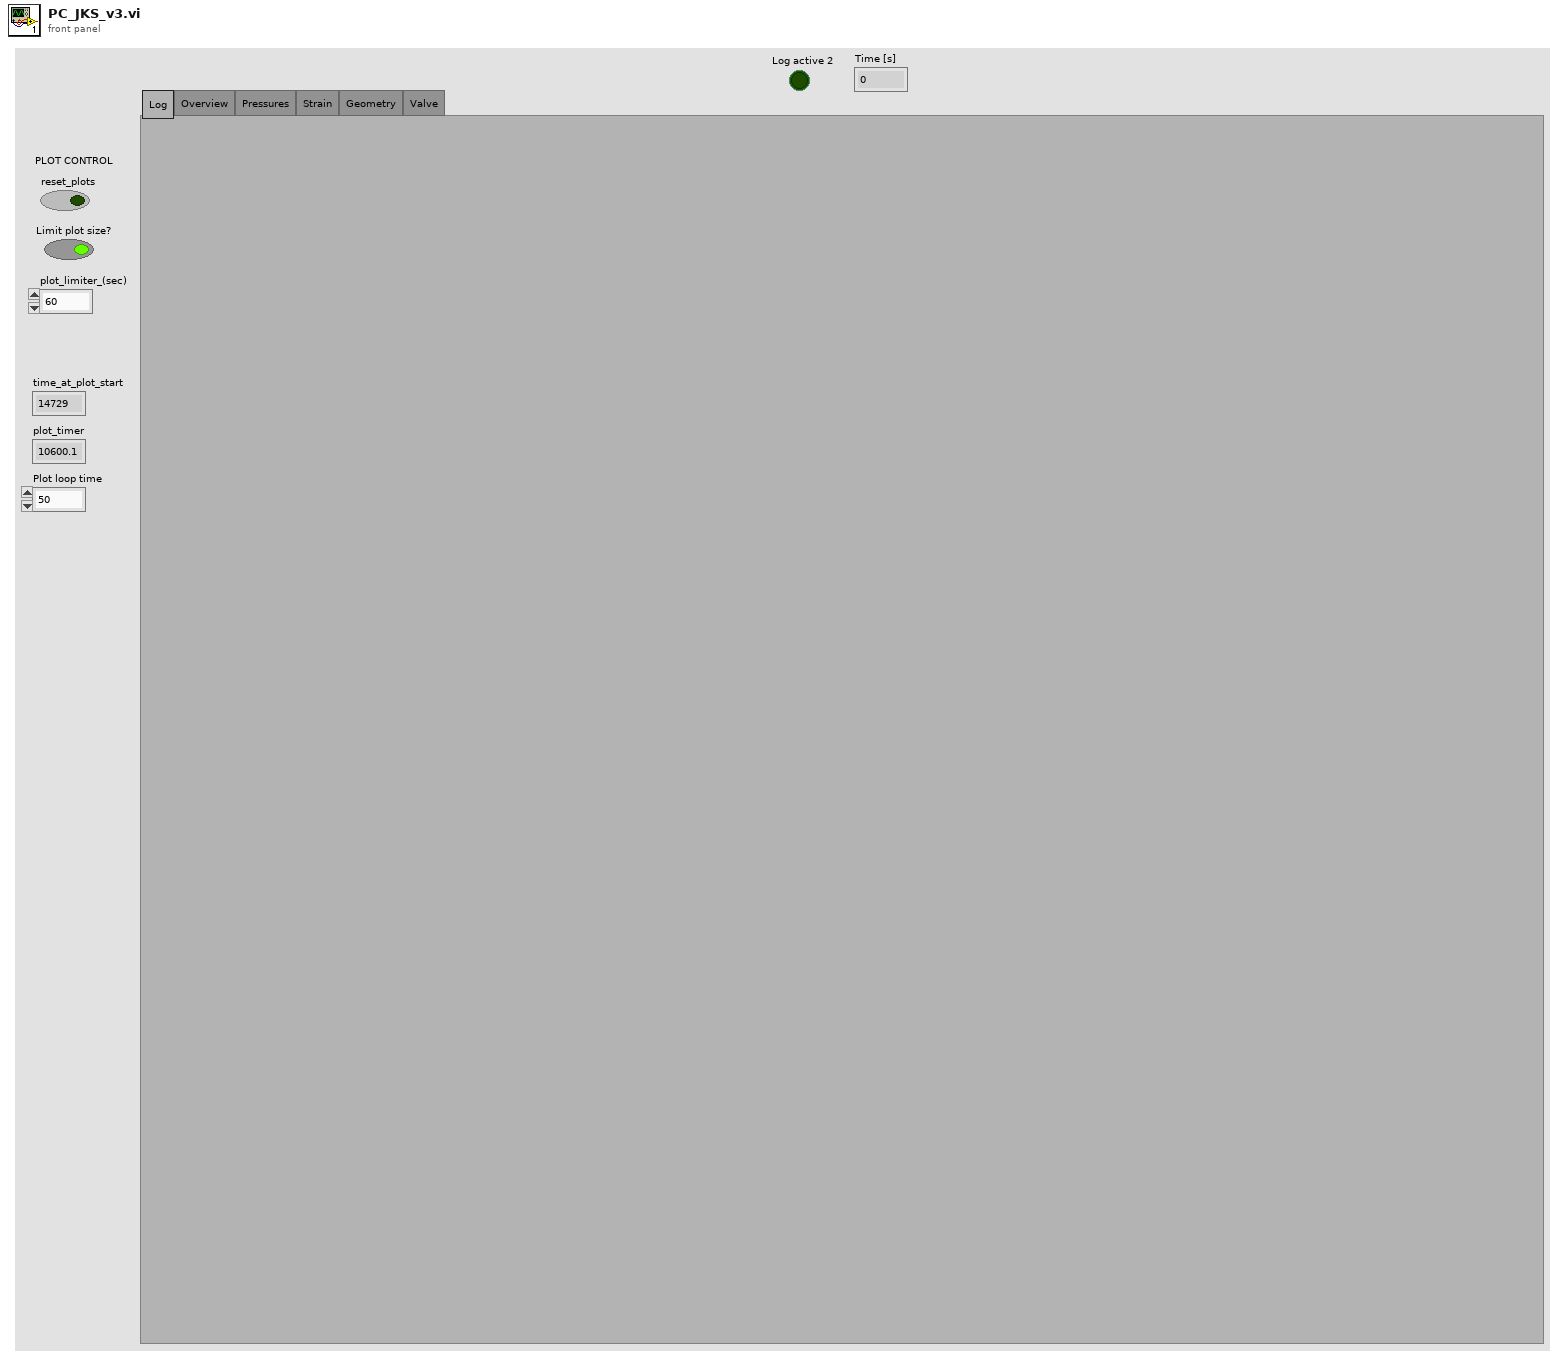
[diagram p1: front panel]
types:
  T1 = enum32{"Log", "Overview", "Pressures", "Strain", "Geometry", "Valve"}
  T2 = cluster{"plot_timer":dbl, "P.A":dbl, "P.B":dbl}[]
  T3 = cluster{cluster{"plot_timer":dbl, "P.comp":dbl, "P.comp":dbl}[]}[]
  T4 = cluster{"plot3":cluster{"timer":sgl, "p_A":sgl, "p_A1":sgl}[]}[]
  T5 = cluster{"plot_timer":dbl, "dl.cyl":dbl, "dl.cyl":dbl}[]
  T6 = cluster{"plot_timer":dbl, "l.cyl":dbl, "l.cyl":dbl}[]
  T7 = cluster{"plot_timer":dbl, "Q.B":dbl, "Q.B":dbl}[]
  T8 = cluster{cluster{"plot_timer":dbl, "u_Bosch":dbl, "u_Bosch":dbl}[]}[]
  T9 = cluster{"plot_timer":dbl, "u_Bosch":dbl, "u_Bosch":dbl}
  T10 = cluster{"plot_timer":dbl, "u_DCV":dbl, "u_DCV_comp":dbl}
  T11 = cluster{"plot_timer":dbl, "Strain_unfiltered":dbl, "Strain_filtered":dbl}
  T12 = cluster{"plot_timer":dbl, "x.c.dot":dbl, "x.c.dot":dbl}
  T13 = cluster{"plot_timer":dbl, "P.comp":dbl, "P.comp":dbl}
  T14 = cluster{"plot_timer":dbl, "P.B":dbl, "P.B.LP":dbl}
  T15 = cluster{"plot_timer":dbl, "P.A1":dbl, "P.comp":dbl}
  T16 = cluster{"plot_timer":dbl, "P.pump":dbl, "P.return":dbl}
  T17 = cluster{"p_pump_p_return":cluster{"timer":sgl, "p_A":sgl, "p_A1":sgl}[]}[]
  T18 = cluster{cluster{"plot_timer":dbl, "P.A":dbl, "P.B":dbl}[]}[]
  T19 = enum16{"open", "open or create", "create or replace", "create", "open (read-only)"}
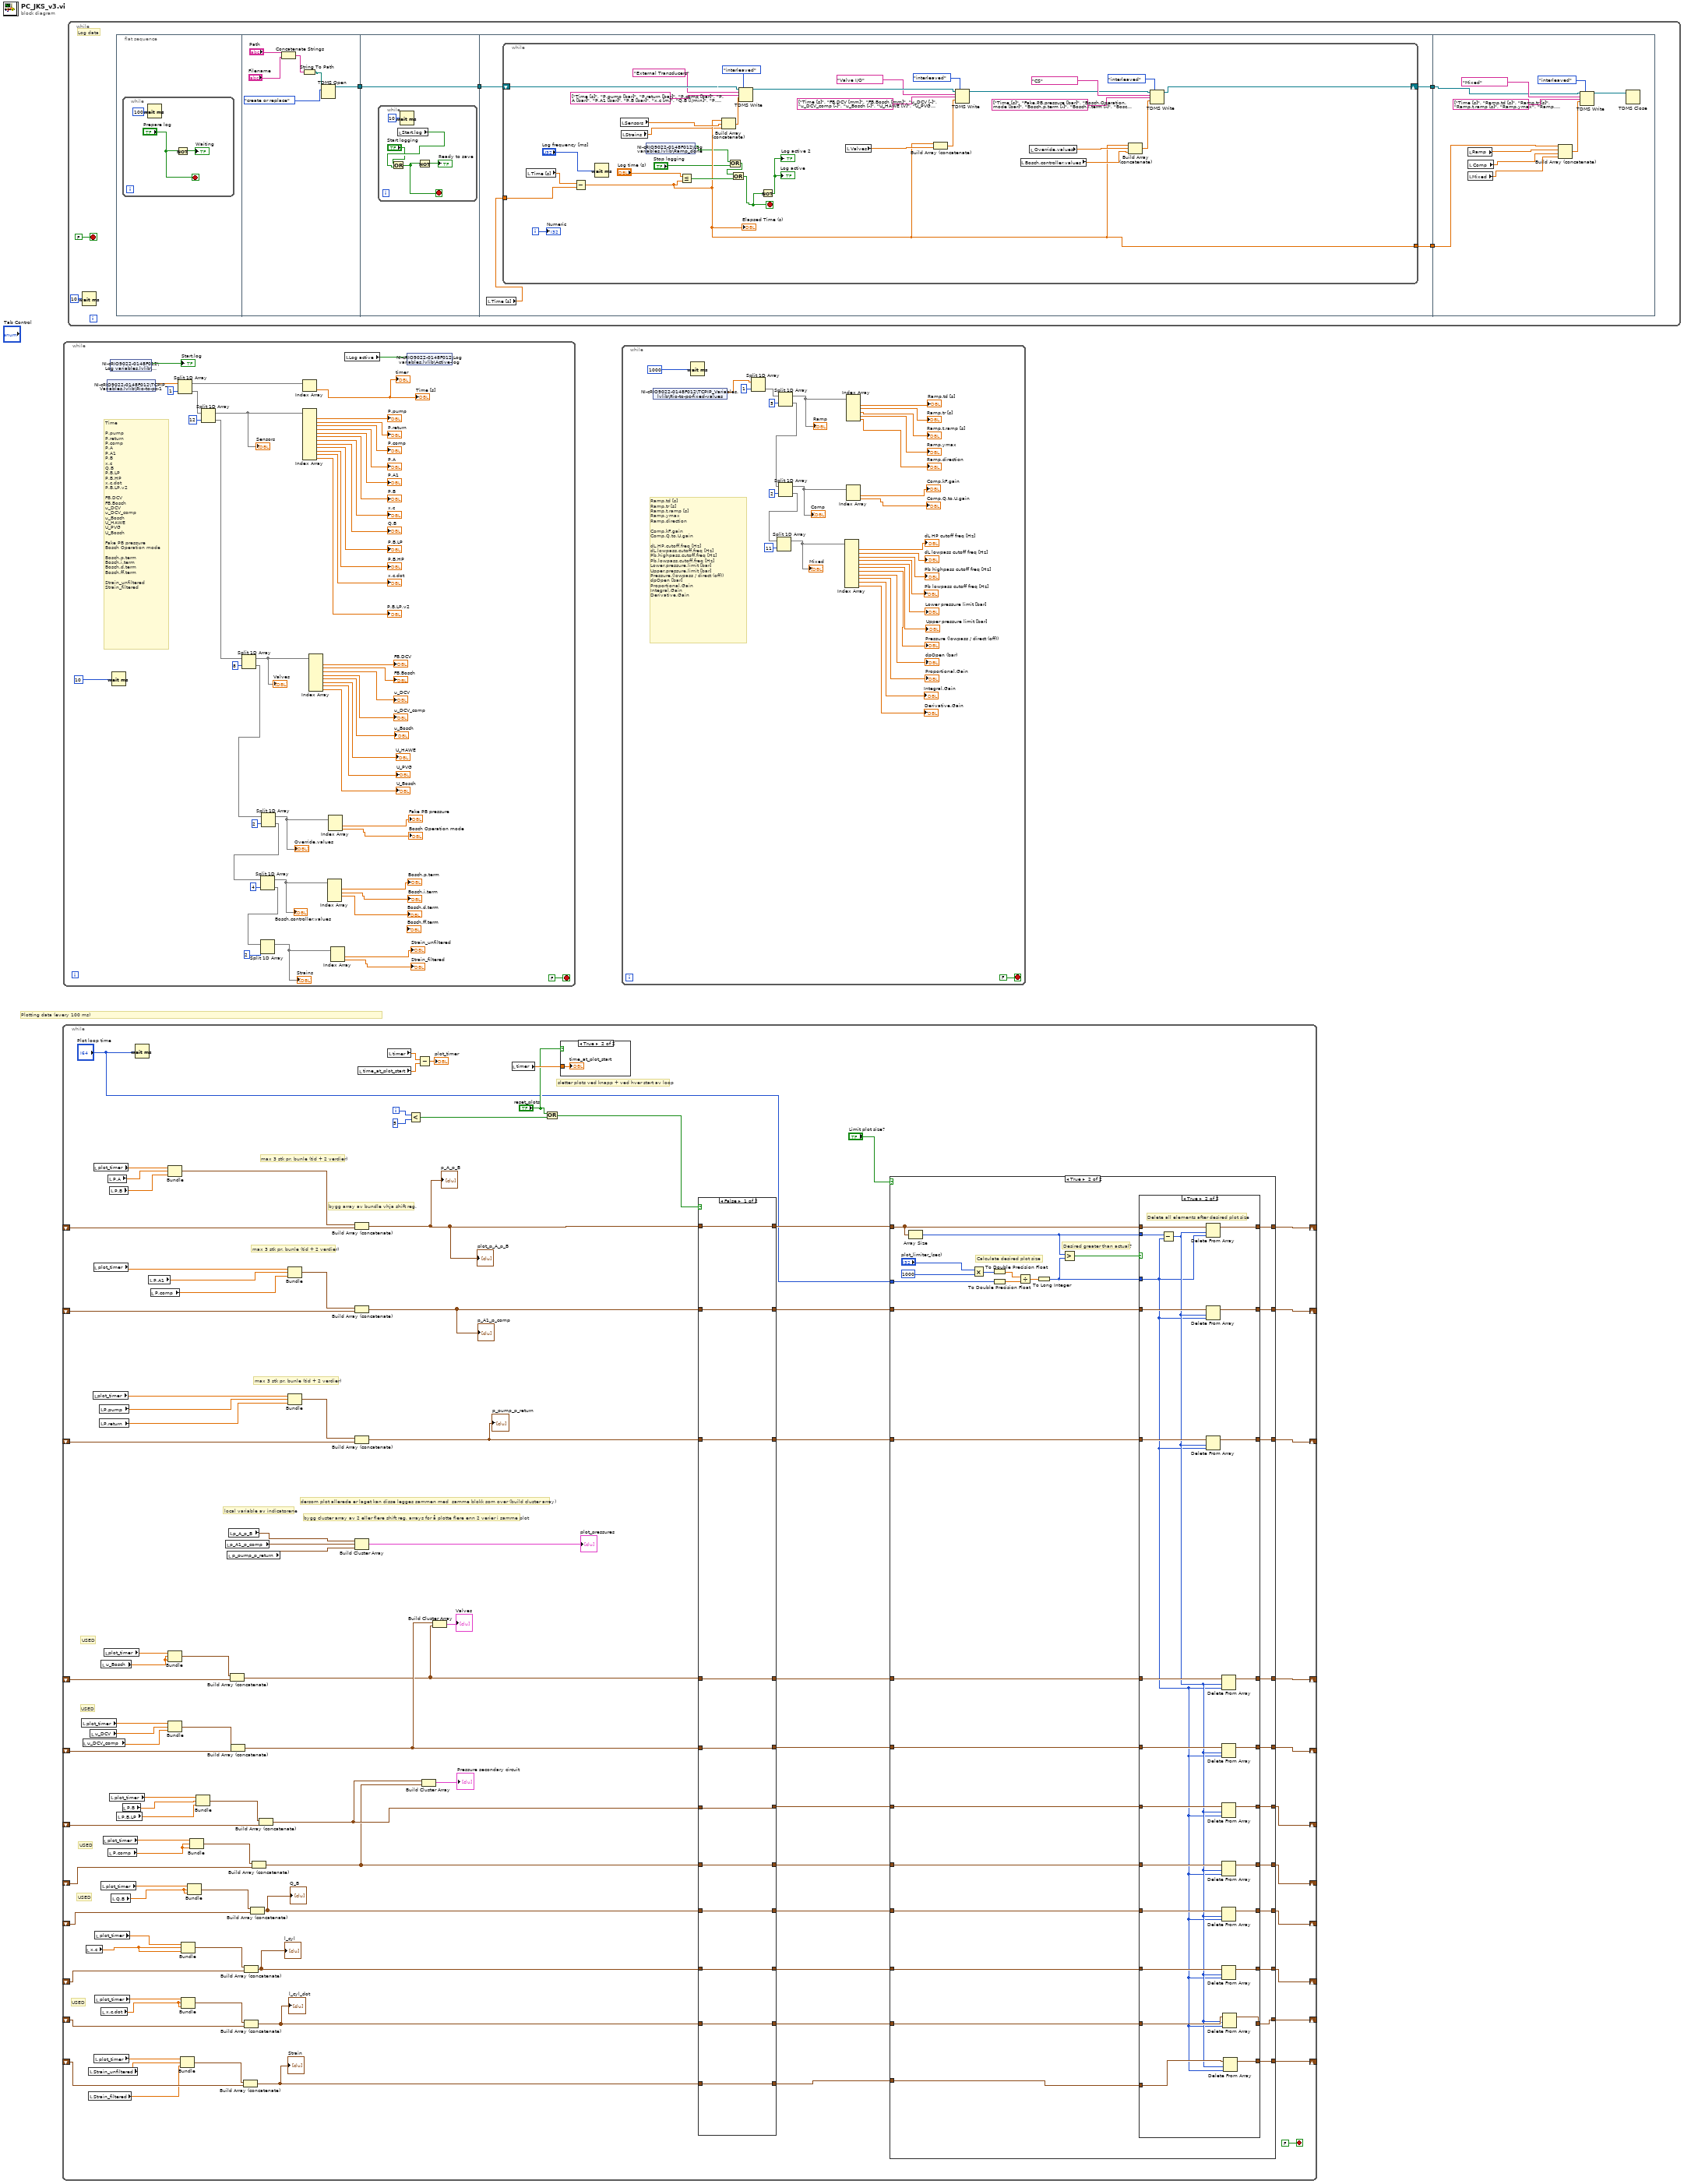
[diagram p0: block diagram]
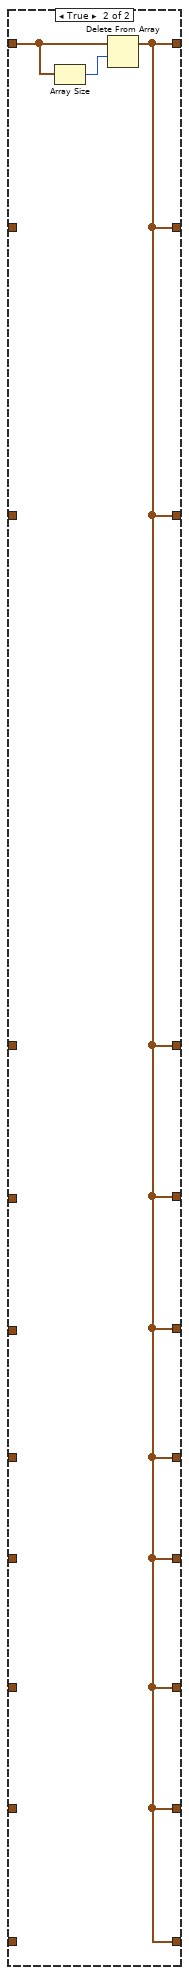
[diagram p5: hidden frame]
diagram:
  # "Plotting data (every 100 ms)"
  n1 = while {
    shift-right: [w77] -> _
    shift-left: _ -> [w101]
    shift-right: [w80] -> _
    shift-left: _ -> [w99]
    shift-right: [w78] -> _
    shift-left: _ -> [w89]
    shift-right: [w71] -> _
    shift-left: _ -> [w69]
    shift-right: [w65] -> _
    shift-left: _ -> [w68]
    shift-right: [w53] -> _
    shift-left: _ -> [w55]
    shift-right: [w43] -> _
    shift-left: _ -> [w46]
    shift-right: [w37] -> _
    shift-left: _ -> [w40]
    shift-right: [w33] -> _
    shift-left: _ -> [w36]
    shift-right: [w27] -> _
    shift-left: _ -> [w32]
    shift-right: [w3] -> _
    shift-left: _ -> [w2]
    i -> [w61]
    stop <- FALSE stop-if-true
    # "USED"
    # "USED"
    # "USED"
    # "USED"
    # "USED"
    # "sletter plots ved knapp + ved hver start av loop"
    # "local variable av indicatorene"
    # "dersom plot allerede er laget kan disse legges sammen med  samme blokk som over (build cluster array)"
    # "bygg array av bundle vhja shift reg."
    # "bygg cluster array av 2 eller flere shift reg. arrays for å plotte flere enn 2 verier i samme plot"
    # "max 3 stk pr. bunle (tid + 2 verdier)"
    # "max 3 stk pr. bunle (tid + 2 verdier)"
    # "max 3 stk pr. bunle (tid + 2 verdier)"
    n2 = local read "plot_timer"() -> (w67:dbl)
    n3 = local read "u_DCV_comp"() -> (w23:dbl)
    n4 = local read "x.c"() -> (w18:dbl)
    n5 = local read "Strain_unfiltered"() -> (w8:dbl)
    n6 = local read "Strain_filtered"() -> (w1:dbl)
    n7 = local read "u_DCV"() -> (w24:dbl)
    n8 = local read "plot_timer"() -> (w91:dbl)
    n9 = local read "plot_timer"() -> (w98:dbl)
    n10 = local read "plot_timer"() -> (w93:dbl)
    n11 = local read "plot_timer"() -> (w7:dbl)
    n12 = local read "plot_timer"() -> (w25:dbl)
    n13 = local read "plot_timer"() -> (w30:dbl)
    n14 = local read "P.pump"() -> (w76:dbl)
    n15 = local read "P.return"() -> (w75:dbl)
    n16 = local read "u_Bosch"() -> (w20:dbl)
    n17 = local read "plot_timer"() -> (w41:dbl)
    n18 = local read "x.c.dot"() -> (w29:dbl)
    n19 = local read "plot_timer"() -> (w48:dbl)
    n20 = local read "plot_timer"() -> (w72:dbl)
    n21 = local read "P.A"() -> (w97:dbl)
    n22 = local read "P.comp"() -> (w47:dbl)
    n23 = local read "P.B"() -> (w96:dbl)
    n24 = local read "plot_timer"() -> (w56:dbl)
    n25 = local read "Q.B"() -> (w9:dbl)
    n26 = local read "P.B.LP"() -> (w10:dbl)
    n27 = local read "P.B"() -> (w11:dbl)
    n28 = Wait (ms)(milliseconds to wait="Plot loop time") -> ()  [unwired: 1 out]
    n29 = local read "P.A1"() -> (w94:dbl)
    n30 = local read "P.comp"() -> (w95:dbl)
    n31 = Bundle("plot_timer"=w72, "u_Bosch"=w20, "u_Bosch"=w20) -> (w51:T9)  [unwired: 1 in]
    n32 = Bundle("plot_timer"=w98, "P.A"=w97, "P.B"=w96) -> (w100:cluster{"plot_timer":dbl, "P.A":dbl, "P.B":dbl})  [unwired: 1 in]
    n33 = Bundle("plot_timer"=w67, "u_DCV"=w24, "u_DCV_comp"=w23) -> (w50:T10)  [unwired: 1 in]
    n34 = Bundle("plot_timer"=w7, "Strain_unfiltered"=w8, "Strain_filtered"=w1) -> (w6:T11)  [unwired: 1 in]
    n35 = Bundle("plot_timer"=w25, "x.c"=w18, "x.c"=w18) -> (w35:cluster{"plot_timer":dbl, "x.c":dbl, "x.c":dbl})  [unwired: 1 in]
    n36 = Bundle("plot_timer"=w30, "x.c.dot"=w29, "x.c.dot"=w29) -> (w31:T12)  [unwired: 1 in]
    n37 = Bundle("plot_timer"=w41, "Q.B"=w9, "Q.B"=w9) -> (w42:cluster{"plot_timer":dbl, "Q.B":dbl, "Q.B":dbl})  [unwired: 1 in]
    n38 = Bundle("plot_timer"=w48, "P.comp"=w47, "P.comp"=w47) -> (w45:T13)  [unwired: 1 in]
    n39 = Bundle("plot_timer"=w56, "P.B"=w11, "P.B.LP"=w10) -> (w49:T14)  [unwired: 1 in]
    n40 = local read "p_A1_p_comp"() -> (w87:cluster{"timer":sgl, "p_A":sgl, "p_A1":sgl}[])
    n41 = local read "p_pump_p_return"() -> (w86:cluster{"timer":sgl, "p_A":sgl, "p_A1":sgl}[])
    n42 = local read "p_A_p_B"() -> (w88:cluster{"timer":sgl, "p_A":sgl, "p_A1":sgl}[])
    n43 = Build Array (concatenate)(w51, w69) -> (w19:T2)
    n44 = Build Array (concatenate)(w50, w68) -> (w22:T2)
    n45 = Build Array (concatenate)(w6, w2) -> (w4:T2)
    "Strain" <- w4
    n46 = Build Array (concatenate)(w35, w36) -> (w17:T2)
    "l_cyl" <- w17
    n47 = Build Array (concatenate)(w31, w32) -> (w26:T2)
    "l_cyl_dot" <- w26
    n48 = Build Array (concatenate)(w42, w40) -> (w39:T2)
    "Q_B" <- w39
    n49 = Build Array (concatenate)(w45, w46) -> (w15:T2)
    n50 = Build Array (concatenate)(w49, w55) -> (w16:T2)
    n51 = Bundle("plot_timer"=w93, "P.A1"=w94, "P.comp"=w95) -> (w92:T15)  [unwired: 1 in]
    n52 = Bundle("plot_timer"=w91, "P.pump"=w76, "P.return"=w75) -> (w90:T16)  [unwired: 1 in]
    n53 = Build Array (concatenate)(w100, w101) -> (w52:T2)
    "p_A_p_B" <- w52
    "plot_p_A_p_B" <- w52
    n54 = Build Array (concatenate)(w92, w99) -> (w74:T2)
    "p_A1_p_comp" <- w74
    n55 = Build Array (concatenate)(w90, w89) -> (w73:T2)
    "p_pump_p_return" <- w73
    n56 = Build Cluster Array(w88, w87, w86) -> (→"plot_pressures":T17)
    n57 = local read "time_at_plot_start"() -> (w59:dbl)
    n58 = local read "timer"() -> (w60:dbl)
    n59 = Less?(x=w61, y=5) -> (x < y?=w84:bool)
    n60 = Subtract(x=w60, y=w59) -> (x-y=→"plot_timer":dbl)
    n61 = Build Cluster Array(w16, w15) -> (→"Pressure secondary circuit":T18)
    n62 = Build Cluster Array(w22, w19) -> (→"Valves":T18)
    n63 = local read "timer"() -> (w62:dbl)
    n64 = Or(x="reset_plots", y=w84) -> (x .or. y?=w63:bool)
    n65 = case shown="True" "reset_plots" {
      tunnel: w62 -> [_ w102]
      frame False {
      }
      frame True {
        "time_at_plot_start" <- w102
      }
    }
    n66 = case shown="False" w63 {
      tunnel: [w192 w193] -> w82
      tunnel: w52 -> [w192 w194]
      tunnel: [w191 w193] -> w81
      tunnel: w74 -> [w191 _]
      tunnel: w73 -> [w190 _]
      tunnel: [w190 w193] -> w79
      tunnel: w19 -> [w189 _]
      tunnel: [w189 w193] -> w70
      tunnel: [w188 w193] -> w66
      tunnel: w22 -> [w188 _]
      tunnel: [w187 w193] -> w54
      tunnel: w16 -> [w187 _]
      tunnel: w15 -> [w186 _]
      tunnel: [w186 w193] -> w44
      tunnel: w39 -> [w185 _]
      tunnel: [w185 w193] -> w38
      tunnel: w17 -> [w184 _]
      tunnel: [w184 w193] -> w34
      tunnel: w26 -> [w183 _]
      tunnel: [w183 w193] -> w28
      tunnel: [w182 w193] -> w5
      tunnel: w4 -> [w182 _]
      frame False {
      }
      frame True {
        n67 = Array Size(array=w194) -> (size(s)=w195:i32)
        n68 = Delete From Array(array=w194, length=w195) -> (array with subset deleted=w193:T2)  [unwired: 1 in, 1 out]
      }
    }
    n69 = case shown="True" "Limit plot size?" {
      tunnel: [w113 w135] -> w77
      tunnel: w82 -> [w113 w140]
      tunnel: [w112 w132] -> w80
      tunnel: w81 -> [w112 w131]
      tunnel: [w111 w134] -> w78
      tunnel: w79 -> [w111 w133]
      tunnel: [w110 w130] -> w71
      tunnel: w70 -> [w110 w129]
      tunnel: w66 -> [w109 w127]
      tunnel: [w109 w128] -> w65
      tunnel: w54 -> [w108 w126]
      tunnel: [w108 w125] -> w53
      tunnel: "Plot loop time" -> [_ w124]
      tunnel: w44 -> [w107 w123]
      tunnel: [w107 w122] -> w43
      tunnel: w38 -> [w106 w121]
      tunnel: [w106 w120] -> w37
      tunnel: w34 -> [w105 w119]
      tunnel: [w105 w118] -> w33
      tunnel: w28 -> [w104 w116]
      tunnel: [w104 w117] -> w27
      tunnel: w5 -> [w103 w115]
      tunnel: [w103 w114] -> w3
      frame False {
      }
      frame True {
        # "Desired greater than actual?"
        # "Calculate desired plot size"
        n70 = Array Size(array=w140) -> (size(s)=w136:i32)
        n71 = Multiply(x="plot_limiter_(sec)", y=1000) -> (x*y=w139:i32)
        n72 = To Double Precision Float(number=w139) -> (double precision float=w143:dbl)
        n73 = To Double Precision Float(number=w124) -> (double precision float=w142:dbl)
        n74 = Divide(x=w143, y=w142) -> (x/y=w138:dbl)
        n75 = To Long Integer(number=w138) -> (32bit integer=w137:i32)
        n76 = Greater?(x=w136, y=w137) -> (0:w141:bool)
        n77 = case shown="True" w141 {
          tunnel: w140 -> [w156 w181]
          tunnel: [w156 w179] -> w135
          tunnel: w137 -> [_ w157]
          tunnel: w136 -> [_ w180]
          tunnel: [w154 w177] -> w134
          tunnel: w133 -> [w154 w178]
          tunnel: [w155 w175] -> w132
          tunnel: w131 -> [w155 w176]
          tunnel: w129 -> [w153 w173]
          tunnel: [w153 w174] -> w130
          tunnel: w127 -> [w152 w172]
          tunnel: [w152 w171] -> w128
          tunnel: [w151 w169] -> w125
          tunnel: w126 -> [w151 w170]
          tunnel: w123 -> [w150 w168]
          tunnel: [w150 w167] -> w122
          tunnel: w121 -> [w149 w166]
          tunnel: [w149 w165] -> w120
          tunnel: w119 -> [w148 w164]
          tunnel: [w148 w163] -> w118
          tunnel: [w147 w161] -> w117
          tunnel: w116 -> [w147 w162]
          tunnel: w115 -> [w146 w160]
          tunnel: [w146 w159] -> w114
          frame False {
          }
          frame True {
            # "Delete all elements after desired plot size"
            n78 = Subtract(x=w180, y=w157) -> (x-y=w158:i32)
            n79 = Delete From Array(array=w181, length=w158, index=w157) -> (array with subset deleted=w179:T2)  [unwired: 1 out]
            n80 = Delete From Array(array=w176, length=w158, index=w157) -> (array with subset deleted=w175:T2)  [unwired: 1 out]
            n81 = Delete From Array(array=w178, length=w158, index=w157) -> (array with subset deleted=w177:T2)  [unwired: 1 out]
            n82 = Delete From Array(array=w173, length=w158, index=w157) -> (array with subset deleted=w174:T2)  [unwired: 1 out]
            n83 = Delete From Array(array=w172, length=w158, index=w157) -> (array with subset deleted=w171:T2)  [unwired: 1 out]
            n84 = Delete From Array(array=w170, length=w158, index=w157) -> (array with subset deleted=w169:T2)  [unwired: 1 out]
            n85 = Delete From Array(array=w168, length=w158, index=w157) -> (array with subset deleted=w167:T2)  [unwired: 1 out]
            n86 = Delete From Array(array=w166, length=w158, index=w157) -> (array with subset deleted=w165:T2)  [unwired: 1 out]
            n87 = Delete From Array(array=w164, length=w158, index=w157) -> (array with subset deleted=w163:T2)  [unwired: 1 out]
            n88 = Delete From Array(array=w162, length=w158, index=w157) -> (array with subset deleted=w161:T2)  [unwired: 1 out]
            n89 = Delete From Array(array=w160, length=w158, index=w157) -> (array with subset deleted=w159:T2)  [unwired: 1 out]
          }
        }
      }
    }
  }
  n90 = while {
    stop <- FALSE stop-if-true
    # "Time\n\nP.pump\nP.return\nP.comp\nP.A\nP.A1\nP.B\nx.c\nQ.B\nP.B.LP\nP.B.HP\nx.c.dot\nP.B.LP.v2\n\nFB.DCV\nFB.Bosch\nu_DCV\nu_DCV_comp\nu_Bosch\nU_HAWE\nU_PVG\nU_Bosch\n\nFake PB pressure\nBosch Operation mode\n\nBosch.p.term\nBosch.i.term\nBosch.d.term\nBosch.ff.term\n\nStrain_unfiltered\nStrain_filtered"
    n91 = shared-variable "NI-cRIO9022-0148F012\\TCPIP_Variables.lvlib\\Rio-to-pc-1"() -> (w236:dbl[])  [unwired: 1 in, 1 out]
    n92 = shared-variable "NI-cRIO9022-0148F012\\Log variables.lvlib\\Start-log"() -> (→"Start.log":bool)  [unwired: 1 in, 1 out]
    n93 = Wait (ms)(milliseconds to wait=i64 10 ("Period")) -> ()  [unwired: 1 out]
    n94 = Split 1D Array(array=w236, index=1) -> (first subarray=w234:dbl[], second subarray=w233:dbl[])
    n95 = Split 1D Array(array=w233, index=12) -> (first subarray=w231:dbl[], second subarray=w229:dbl[])
    "Sensors" <- w231
    n96 = Split 1D Array(array=w229, index=8) -> (first subarray=w228:dbl[], second subarray=w207:dbl[])
    "Valves" <- w228
    n97 = Split 1D Array(array=w207, index=2) -> (first subarray=w210:dbl[], second subarray=w202:dbl[])
    "Override.values" <- w210
    n98 = Split 1D Array(array=w202, index=4) -> (first subarray=w204:dbl[], second subarray=w196:dbl[])
    "Bosch.controller.values" <- w204
    n99 = Split 1D Array(array=w196, index=2) -> (first subarray=w198:dbl[])  [unwired: 1 out]
    "Strains" <- w198
    n100 = Index Array(array=w234) -> (element=→"timer" →"Time [s]":dbl)  [unwired: 1 in]
    n101 = Index Array(array=w231) -> (element #1=→"P.pump":dbl, element #2=→"P.return":dbl, element #3=→"P.comp":dbl, element #4=→"P.A":dbl, element #5=→"P.A1":dbl, element #6=→"P.B":dbl, element #7=→"x.c":dbl, element #8=→"Q.B":dbl, element #9=→"P.B.LP":dbl, element #10=→"P.B.HP":dbl, element #11=→"x.c.dot":dbl, element #12=→"P.B.LP.v2":dbl)  [unwired: 12 in]
    n102 = Index Array(array=w228) -> (element #1=→"FB.DCV":dbl, element #2=→"FB.Bosch":dbl, element #3=→"u_DCV":dbl, element #4=→"u_DCV_comp":dbl, element #5=→"u_Bosch":dbl, element #6=→"U_HAWE":dbl, element #7=→"U_PVG":dbl, element #8=→"U_Bosch":dbl)  [unwired: 8 in]
    n103 = Index Array(array=w204) -> (element #1=→"Bosch.p.term":dbl, element #2=→"Bosch.i.term":dbl, element #3=→"Bosch.d.term":dbl)  [unwired: 4 in, 1 out]
    n104 = Index Array(array=w210) -> (element #1=→"Fake PB pressure":dbl, element #2=→"Bosch Operation mode":dbl)  [unwired: 2 in]
    n105 = Index Array(array=w198) -> (element #1=→"Strain_unfiltered":dbl, element #2=→"Strain_filtered":dbl)  [unwired: 2 in]
    n106 = local read "Log active"() -> (w218:bool)
    n107 = shared-variable "NI-cRIO9022-0148F012\\Log variables.lvlib\\Active-log"(w218) -> ()  [unwired: 1 in, 1 out]
  }
  n108 = while {
    stop <- FALSE stop-if-true
    # "Log data"
    n109 = Wait (ms)(milliseconds to wait=u32 10) -> ()  [unwired: 1 out]
    n110 = flat-sequence {
      tunnel: [w259] -> w249
      tunnel: [w261] -> w248
      tunnel: w249 -> [w261]
      tunnel: w248 -> [w270]
      tunnel: [w269] -> w247
      tunnel: [w267] -> w246
      tunnel: w247 -> [w307]
      tunnel: w246 -> [w305]
      frame #0 {
        n111 = while {
          stop <- "Prepare log" stop-if-true
          n112 = Wait (ms)(milliseconds to wait=u32 100) -> ()  [unwired: 1 out]
          n113 = Not(x="Prepare log") -> (.not. x?=→"Waiting":bool)
        }
      }
      frame #1 {
        n114 = Concatenate Strings("Path", "Filename") -> (w256:string)
        n115 = String To Path(string=w256) -> (path=w258:path)
        n116 = TDMS Open(10:T19."create or replace" ("operation (0:open)"), 11:w258) -> (3:w259:refnum<k34>)  [unwired: 5 in, 1 out]
      }
      frame #2 {
        n117 = while {
          stop <- w262 stop-if-true
          n118 = local read "Start.log"() -> (w264:bool)
          n119 = Or(x="Start logging", y=w264) -> (x .or. y?=w262:bool)
          n120 = Wait (ms)(milliseconds to wait=u32 10) -> ()  [unwired: 1 out]
          n121 = Not(x=w262) -> (.not. x?=→"Ready to save":bool)
        }
      }
      frame #3 {
        n122 = local read "Time [s]"() -> (w268:dbl)
        n123 = while {
          shift-right: [w275] -> w269
          shift-left: w270 -> [w300]
          tunnel: w268 -> [w294]
          tunnel: [w276] -> w267
          i -> [w303]
          stop <- w284 stop-if-true
          n124 = local read "Time [s]"() -> (w291:dbl)
          n125 = Subtract(x=w291, y=w294) -> (x-y=w276:dbl)
          "Elapsed Time (s)" <- w276
          n126 = Wait (ms)(milliseconds to wait="Log frequency [ms]") -> ()  [unwired: 1 out]
          n127 = local read "Sensors"() -> (w287:dbl[])
          n128 = local read "Strains"() -> (w271:dbl[])
          n129 = shared-variable "NI-cRIO9022-0148F012\\Log variables.lvlib\\Ramp_done"() -> (w274:bool)  [unwired: 1 in, 1 out]
          n130 = Less Or Equal?(x="Log time (s)", y=w276) -> (x <= y?=w285:bool)
          n131 = Build Array (concatenate)(w276, w287, w271) -> (w295:dbl[])
          n132 = Or(x=w274, y="Stop logging") -> (x .or. y?=w272:bool)
          n133 = Or(x=w272, y=w285) -> (x .or. y?=w284:bool)
          n134 = TDMS Write(0:w300, 1:enum16{"decimated", "interleaved"}."interleaved" ("data layout (0:decimated)"), 5:"External Transducers" ("group name in (Untitled)"), 7:string[] ["Time [s]", "P.pump [bar]", "P.return [bar]", "P.comp [bar]", "P.A [bar]", "P.A1 [bar]", "P.B [bar]", "x.c [m]", "Q.B [l/min]", "P.B.LP [bar]", "P.B.HP [bar/s]", "x.c.dot [m/s]", "P.B.LP.v2 [bar]", "Strain_unfiltered", "Strain_filtered"] ("channel name(s) in (Untitled)"), 9:w295) -> (4:w299:refnum<k34>)  [unwired: 1 in, 3 out]
          n135 = Not(x=w284) -> (.not. x?=→"Log active" →"Log active 2":bool)
          n136 = local read "Valves"() -> (w286:dbl[])
          n137 = Build Array (concatenate)(w276, w286) -> (w289:dbl[])
          n138 = TDMS Write(0:w299, 1:enum16{"decimated", "interleaved"}."interleaved" ("data layout (0:decimated)"), 5:"Valve I/O" ("group name in (Untitled)"), 7:string[] ["Time [s]", "FB.DCV [mm]", "FB.Bosch [mm]", "u_DCV [-]", "u_DCV_comp [-]", "u_Bosch [-]", "U_HAWE [V]", "U_PVG [V]", "U_Bosch [V]"] ("channel name(s) in (Untitled)"), 9:w289) -> (4:w278:refnum<k34>)  [unwired: 1 in, 3 out]
          n139 = local read "Bosch.controller.values"() -> (w277:dbl[])
          n140 = local read "Override.values"() -> (w283:dbl[])
          n141 = Build Array (concatenate)(w276, w283, w277) -> (w282:dbl[])
          n142 = TDMS Write(0:w278, 1:enum16{"decimated", "interleaved"}."interleaved" ("data layout (0:decimated)"), 5:"CS" ("group name in (Untitled)"), 7:string[] ["Time [s]", "Fake.PB.pressure [bar]", "Bosch.Operation.mode [bar]", "Bosch.p.term [-]", "Bosch.i.term [-]", "Bosch.d.term [-]", "Bosch.ff.term [-]"] ("channel name(s) in (Untitled)"), 9:w282) -> (4:w275:refnum<k34>)  [unwired: 1 in, 3 out]
          "Numeric" <- w303
        }
      }
      frame #4 {
        n143 = local read "Ramp"() -> (w312:dbl[])
        n144 = local read "Mixed"() -> (w304:dbl[])
        n145 = local read "Comp"() -> (w313:dbl[])
        n146 = Build Array (concatenate)(w305, w312, w313, w304) -> (w308:dbl[])
        n147 = TDMS Write(0:w307, 1:enum16{"decimated", "interleaved"}."interleaved" ("data layout (0:decimated)"), 5:"Mixed" ("group name in (Untitled)"), 7:string[] ["Time [s]", "Ramp.td [s]", "Ramp.tr [s]", "Ramp.t.ramp [s]", "Ramp.ymax", "Ramp.direction", "Comp.kF.gain", "Comp.Q.to.U.gain", "dL.HP.cutoff.freq [Hz", "dL.lowpass.cutoff.freq [Hz]", "Pb.highpass.cutoff.freq [Hz]", "Pb.lowpass.cutoff.freq [Hz]", "Lower.pressure.limit [bar]", "Upper.pressure.limit [bar]", "Pressure.(lowpass / direct (off))", "dpOpen [bar]", "Proportional.Gain", "Integral.Gain", "Derivative.Gain"] ("channel name(s) in (Untitled)"), 9:w308) -> (4:w306:refnum<k34>)  [unwired: 1 in, 3 out]
        n148 = TDMS Close(11:w306) -> ()  [unwired: 1 in, 2 out]
      }
    }
  }
  n149 = while {
    stop <- FALSE stop-if-true
    # "Ramp.td [s]\nRamp.tr [s]\nRamp.t.ramp [s]\nRamp.ymax\nRamp.direction\n\nComp.kF.gain\nComp.Q.to.U.gain\n\ndL.HP.cutoff.freq [Hz]\ndL.lowpass.cutoff.freq [Hz]\nPb.highpass.cutoff.freq [Hz]\nPb.lowpass.cutoff.freq [Hz]\nLower.pressure.limit [bar]\nUpper.pressure.limit [bar]\nPressure.(lowpass / direct (off))\ndpOpen [bar]\nProportional.Gain\nIntegral.Gain\nDerivative.Gain"
    n150 = shared-variable "NI-cRIO9022-0148F012\\TCPIP_Variables.lvlib\\Rio-to-pc-fixed-values"() -> (w315:dbl[])  [unwired: 1 in, 1 out]
    n151 = Wait (ms)(milliseconds to wait=i64 1000 ("Period")) -> ()  [unwired: 1 out]
    n152 = Split 1D Array(array=w315, index=1) -> (second subarray=w314:dbl[])  [unwired: 1 out]
    n153 = Split 1D Array(array=w314, index=5) -> (first subarray=w333:dbl[], second subarray=w342:dbl[])
    "Ramp" <- w333
    n154 = Split 1D Array(array=w342, index=2) -> (first subarray=w341:dbl[], second subarray=w328:dbl[])
    "Comp" <- w341
    n155 = Split 1D Array(array=w328, index=11) -> (first subarray=w330:dbl[])  [unwired: 1 out]
    "Mixed" <- w330
    n156 = Index Array(array=w330) -> (element #1=→"dL HP cutoff freq [Hz]":dbl, element #2=→"dL lowpass cutoff freq [Hz]":dbl, element #3=→"Pb highpass cutoff freq [Hz]":dbl, element #4=→"Pb lowpass cutoff freq [Hz]":dbl, element #5=→"Lower pressure limit [bar]":dbl, element #6=→"Upper pressure limit [bar]":dbl, element #7=→"Pressure (lowpass / direct (off))":dbl, element #8=→"dpOpen (bar)":dbl, element #9=→"Proportional.Gain":dbl, element #10=→"Integral.Gain":dbl, element #11=→"Derivative.Gain":dbl)  [unwired: 11 in]
    n157 = Index Array(array=w333) -> (element #1=→"Ramp.td [s]":dbl, element #2=→"Ramp.tr [s]":dbl, element #3=→"Ramp.t.ramp [s]":dbl, element #4=→"Ramp.ymax":dbl, element #5=→"Ramp.direction":dbl)  [unwired: 5 in]
    n158 = Index Array(array=w341) -> (element #1=→"Comp.kF.gain":dbl, element #2=→"Comp.Q.to.U.gain":dbl)  [unwired: 2 in]
  }
